vi "Core_Chem_User_Interface_v3.1.vi"() -> ()   [LabVIEW 2014]
uses:
  <vilib>/dex/Stream Element Allocation Mode.ctl
  C:/Program Files (x86)/National Instruments/LabVIEW 2014/examples/Data Communication/Network Streams/Simple Network Streams/support/Network Stream Command.ctl
  <vilib>/Platform/TimedLoop/XDataNode/timing_clust.ctl
  <vilib>/Platform/TimedLoop/XDataNode/nitl_modes.ctl
  <vilib>/Platform/TimedLoop/XDataNode/wakeup.ctl
  <vilib>/Utility/tcp.llb/UDP Multicast Read-Only Open.vi
  <vilib>/platform/TimedLoop/XDataNode/XDataNode.xnode
  <vilib>/Platform/TimedLoop/XDataNode/XDNodeRunTimeDep.lvlib
  <vilib>/FTP/NI_FTP.lvlib
panel:
  out "Network disconnected":bool
  out "cRIO connection status":bool
  out "Network Check error out":errorcluster
  out "SO2 Zeroing (Inflight)\nTime Remain (sec)":u32
  in  "eV6 User set time \n(Inflight) (sec)":i32=120
  in  "SO2 Inflight \nZeroing":bool
  out "Create folder error out 2":errorcluster
  out "Create folder error out":errorcluster
  in  "Confirm Flight Number":bool
  out "PRTAFT_UDP_In":string
  out "TWBOZO01":string
  out "CABOZO01":string
  out "TEIOZO01":string
  out "CHTSOO01":string
  out "CHFGGA01":string
  out "AL52CO01":string
  in  "Flight Number":string
  in  "Tab Control":T1(tab)
  out "FGGA preflight Des 17":string="Preflight - Start minimum 2 hours before take-off\n\n1. Ensure no bags/jackets are stowed on seat backs and behind seats in front of core chemistry rack at all times.\n\n2. Remove inlet covers if applicable.\n\n3. Connect Lilliput mini TFT/LCD VGA cable to FGGA VIDEO (back panel) and PS2 Keyboard/Mouse cables to FGGA Connectors (back panel). TFT/LCD screen kept in WAS/GAS rack Zargers Box. Keyboard/Mouse kept bottom of chemistry rack. (DO NOT disconnect PS2 cable). Connect TFT/LCD AC/DC PSU to 6026-8-98 Amphenol (SSP9) and make 230 Vac CB.\n\n4. Ensure all circuit breakers are pushed in, except 230Vac and 28Vdc, UPS switch off (down) and AL5002 CO Plasma Lamp switch off (down), WoW key to normal (horizontal).\n\n5. Wait for ALL network switches on the aircraft to be up and running before start-up. On the Flight Manager's Interface on the Flight Manager laptop, check SSP icons status (top row) should be all green.  \n\n6. Check AboutTime has synchronised laptop clock to aircraft timeservers (Filiberto/Gaston).\n\nClick the PowerUp Tab."
  out "FGGA preflight Des 16":string="PowerUp\n\n1.\tSSP9 forward face\tMake 3 CBs\n\n2.\tPWRDIST \t\tMake 230Vac CB \n                     Switch UPS On \t[UP]\n                     Make 28Vdc CB\n                     Check 28VDC OK Green Light comes on\n\n3.\tCore Chemistry e-Log\nComplete Core Chemistry e-Log in WordPad (Bnnn_CoreChemLog_v2.2), save on Flight Manager's laptop (192.168.101.180/      flt_folders/Bnnn); Fill in header with date, flight number and your name/initials.\n\n4. Wait for MFM flow rate to display non zero value.\n\n5.\tSAMPUMP\t\t\n - Switch WoW override key (vertical) to check pump starts, and MFM flowrate increase (>20 LPM) on the right hand plot. \n - Switch off WoW override\t\t\t\t [NORM, key horizontal]\n\nClick the 2B Ozone tab if operated, otherwise, click the UDP tab.\n\n\n"
  out "MFM":dbl(graph)
  in  "Ambient = OFF\nCabin = ON":bool
  out "FGGA preflight Des 15":string="2B Ozone Preflight\n\n1.\tSelect either Ambient or Cabin Air mode (default should be OFF for Ambient air mode).\n\n2. Check flowrate is greater than 2000 sccm on the right hand plot.\n\nClick the UDP tab."
  out "2B Ozone concentration":dbl(graph)
  out "2B Ozone flow rate":dbl(graph)
  out "2BOzone Event error out":errorcluster
  out "2BOzone command sender error out":errorcluster
  out "FGGA preflight Des 20":string="4. Check derived parameters in DECADES (192.168.101.110 & 192.168.101.108). 574 Ozone TEi49C; 588 CO AL5002; 611 SO2 TEi43i; 903 - 905 FGGA; 910 / 920 Ozone 2B."
  out "FGGA preflight Des 14":string="UDP Preflight\n1. Check all UDP packets are updating.  Unix time increasing by 1 sec (3rd parameter).\n2. Check flight number is correct.\n3. Confirm flight number and check it appears in the UDP packet (6th parameter). "
  in  "name":string="239.1.4.6"
  in  "Port":u16=50001
  out "FGGA":string
  out "CO":string
  out "TEi49 Ozone":string
  out "2B Cabin Ozone":string
  out "2B Ambient Ozone":string
  out "SO2":string
  in  "Ozone Zeroing Abort":bool
  out "Ozone Zeroing\nTime Remain (sec)":u32
  in  "Ozone Zeroing":bool
  out "TEI49 Sample Flow B":dbl(graph)
  out "TEi49 Concentration":dbl(graph)
  out "TEI49 Sample Flow A":dbl(graph)
  out "FGGA preflight Des 13":string="TEi49 Ozone PRE-FLIGHT - LAST ACTIONS BEFORE SEAT-BELTING DOWN (PRIOR TO ENGINES START)\n\n1. Ozone monitor zeroing\t\t[10 min minimum]\n\n\n2. Check TEi49 zero value and note down value in e-Log. \n"
  out "FGGA preflight Des 12":string="TEi49 Ozone Preflight\n\n1. Check nominal sample flowrate on both channels is ~0.7 LPM."
  out "Ozone Event error out":errorcluster
  out "Ozone command sender error out":errorcluster
  in  "Ozone UDP Time Offset":i32=1
  in  "eV8 span\n(sec)":i32=120
  in  "eV9 span\nflush (sec)":i32=60
  in  "SO2 Span Calibration":bool
  in  "eV9 zero\nflush (sec)":i32=15
  in  "SO2 Zero Calibration":bool
  in  "eV8 zero\n(sec)":i32=30
  in  "SO2 Calibration Abort":bool
  out "SO2 react pressure":dbl(graph)
  in  "Prepare SO2 Zero Gas":bool
  in  "Prepare SO2 Span Gas":bool
  in  "Auto Zeroing \ninterval (sec)":i32=600
  out "Next Auto Zero\nStarts in (sec)":u32
  out "Auto Zero\nIndicator":string="Auto Zero Inactive; Manual Zero Allow"
  out "SO2 Resume Zeroing\nCount down timer (sec)":u32
  in  "SO2 Pause\nAuto Zeroing":bool
  out "TEi43i Concentration scaled / raw":cluster{dbl, dbl}(graph)
  in  "SO2 Auto Zeroing":bool
  out "mean zero\ncal status":bool
  out "SO2 Sensitivity":dbl format="%.2g"
  out "SO2 Zero":dbl format="%.2g"
  in  "eV9 Flush User\nset time (sec)":i32=15
  in  "MFC_3 User Set Value":dbl=2.0
  in  "MFC_2 User Set Value":dbl=2.5
  in  "eV6 User\nset time (sec)":i32=600
  out "SO2 Flush\nTime Remain (sec)":u32
  out "TEI43i MFC3 Sample Flow":dbl(graph)
  out "TEI43C Sample Flow":dbl(graph)
  out "TEI43i MFC2 Cal Flow":dbl(graph)
  out "SO2 Zero CAL\nTime Remain (sec)":u32
  out "SO2 Zero CAL Flush\nTime Remain (sec)":u32
  in  "SO2 Zero CAL":bool
  out "FGGA preflight Des 11":string="TEi43 SO2 Inflight Zero Calibration"
  in  "SO2 GND Zeroing":bool
  out "SO2 Zeroing\nTime Remain (sec)":u32
  out "FGGA preflight Des 10":string="TEi43 SO2 PRE-FLIGHT - LAST ACTIONS BEFORE SEAT-BELTING DOWN (PRIOR TO ENGINES START)\n\n1. SO2 monitors zeroing\t\t[10 min minimum]\n\n2. Check TEi43i or TEi43C zero value and note down value in e-Log.\n\n3. Enable SO2 auto zeroing (if required) and check zeroing interval. "
  in  "SO2 Flush":bool
  out "FGGA preflight Des 9":string="TEi43 SO2 Preflight\n\n1. Check nominal sample flowrate is (2.0 LPM / 1.5 LPM) on the (TEi43i / TEi43c) right hand plot.\n\nSPAN GAS\n1. Connect SO2 Calibration gas to caldeck, then.\n\n2. Press SO2 flush button, MFC2 cal flow should increase to 2.5 SLPM.\nMonitor MFC2 flow rate to make sure the reading decreases from 2.5 SLPM to 0.0 SLPM.\nCheck pressure content and delivery gauges also reads zero.\nIf pressure content & delivery gauges do NOT read zero, press SO2 flush button again until they do.\n\n3. Back out V2, Quickly open and close cylinder valve 1, Set delivery pressure to 3 bar on V2. \n\n4. Repeat step 2) to 3) three times.\n\n5. Open cylinder valve 1, system is ready. Note down content pressure in elog.\n\n6. Press SO2 Span Calibration button to start Span calibration. \n\nZERO AIR\n1. Connect BTCA Zero Air gas to caldeck, then.\n\n2. Set ev9 flush user time to 60 secs and press SO2 Flush button.\n\n3. Press SO2 Zero Calibration button to start Zero Air calibration."
  in  "eV9 flush User\nset time (sec)":i32=30
  in  "eV8 User\nset time (sec)":i32=60
  out "SO2 Event error out":errorcluster
  out "SO2 command sender \nerror out":errorcluster
  in  "SO2 UDP Time Offset":i32=1
  in  "CO Monitor Troubleshooting":bool
  out "Lamp Temperature":dbl(graph)
  out "CO CAL Status":bool
  in  "CO CAL":bool
  out "FGGA preflight Des 8":string="CO Preflight and Inflight Calibrations\nHold down the CAL button for 2 secs then release, CAL status should then lit up.\nCheck CO LED lit up at front instrument. If not, refer to\nInflight calibration performed on 45 minutes interval or more frequently if lamp temperature > 35.5 degC."
  in  "Prepare Gases":bool
  out "FGGA preflight Des 7":string="AL5002 CO Preflight Checks\n\n1.\n\n2. Start CO Vacuum. NB: If there is problem with the software control, use manual override switch [up] on CALDECK front panel\n\n3. CO Checks - charts on the right hand side\n    Lamp Flow Controller ~ 40 ml/min\n    Monochromator Flow Controller ~ 30 ml/min\n    Fluorescence Cell Pressure ~ 7.5 Torr\n\nIf Lamp/Mono flows are low, manual valves (V1 -> V5) may still be shut, or pressure adjusting valves (ALREG1 & 2) have not been set > 2 bar\n\nIf Cell pressure is 10 Torr (max range), check that COPUMP is running and eV7 is opened (CO Vacuum eV7 is ON).\n\n4. Switch Plasma Lamp at the front panel UP\n\nDetector count rate (on 'Raw Signal' or F2 instrument touchscreen) should increase to >=10000 Hz within a minute.  Recycle plasma lamp switch (off/on) if no significant increase in count rate after 10 mins.  CO concentration should increase (100s ppb). \n     \n\n"
  in  "CO Vaccum (eV7)":bool
  out "Raw Signal":dbl(graph)
  out "CO Concentration":dbl(graph)
  out "Fluorescence Cell Pressure":dbl(graph)
  out "Monochromator Flow":dbl(graph)
  out "Lamp Flow Controller":dbl(graph)
  in  "CO UDP Time Offset":i32=1
  out "CO2 Pressure\nDelivery (PSIA)":dbl(slide) scale=0.0..100.0
  out "Std\nContent (barG)":dbl(slide) scale=0.0..220.0
  out "N2\nContent (barG)":dbl(slide) scale=0.0..220.0
  out "CO2\nContent (barG)":dbl(slide) scale=0.0..170.0
  out "CO Event error out":errorcluster
  out "CO command sender error out":errorcluster
  out "CO Zero":T2(array[cluster])
  out "CO Sensitivity":T3(array[cluster])
  in  "FGGA Calibration Abort":bool
  out "Ring Down Time RDA & RDB":cluster{dbl, dbl}(graph)
  in  "Line Lock Setting Change":bool
  out "Cell temperature":dbl(graph)
  out "Cell pressure":dbl(graph)
  in  "Manual FGGA Pump":bool
  out "CO2":dbl(graph)
  out "CH4":dbl(graph)
  out "H2O":dbl(graph)
  out "WoW Flag":string="0"
  in  "FGGA pump\nsync to WoW":bool
  out "CH4 Dry":dbl(graph)
  out "CO2 Dry":dbl(graph)
  out "MFC1 Cal Flow":dbl(graph)
  out "Flush Target Tank\nTime Remain (sec)":u32
  out "Flush Low Tank\nTime Remain (sec)":u32
  out "Flush High Tank\nTime Remain (sec)":u32
  in  "Flush Target Tank":bool
  in  "Flush Low Tank":bool
  in  "Flush High Tank":bool
  in  "FGGA Restart":bool
  out "FGGA preflight Des 6":string="FGGA Instrument Controls"
  in  "High Cal":bool
  out "High Cal\nFlush Time Remain (sec)":u32
  out "High Cal\nCal Time Remain (sec)":u32
  in  "Low Cal":bool
  in  "Target Cal":bool
  in  "Span Cal - \nHigh Cal, CO Cal, Low Cal":bool
  out "Low Cal\nFlush Time Remain (sec)":u32
  out "Low Cal\nCal Time Remain (sec)":u32
  out "Target Cal\nFlush Time Remain (sec)":u32
  out "Target Cal\nCal Time Remain (sec)":u32
  in  "MFC_1 User Set Value":dbl=2.0
  out "FGGA preflight Des 5":string="FGGA Inflight Calibrations"
  out "FGGA preflight Des 4":string="FGGA Ground Preflight Checks\n\n1. Switch FGGA pump ON\n\n2. Check cavity pressure ~50 Torr\n\n3. Switch FGGA pump OFF\n\n4. Enable FGGA pump sync to WoW\n\n5.. Check Time Synchronisation\n\n6. Check CO2 & CH4 values\n\nIf CO2 & CH4 values are -1 ppm, follow the \nchange linelock settings procedure.\n\n\n\n\n\nLAST ACTION BEFORE SEAT-BELTING \nDOWN (PRIOR TO ENGINES START)\n\n1. Disconnect Monitor & stow away. Leave Keyboard & Mouse connected. Place keyboard at the bottom\nof the rack.\n\n"
  out "FGGA preflight Des 3":string="FGGA CAL Gas Purge\n\nFor each cylinder in gas stowage, check that,\n\n1. V1 Closed\n    V3 Closed\n    V4 Make sure arrow positioned downwards (i.e. flow points to gas line)\n\n2. V3 Open (turn anti-clockwise)\n\n3. Use the button on the right according to the operating cylinder to flush the line. Monitor the MFC flow rate to make sure the reading decreases from 3 to zero. (ie fully flushed). Pressure content & delivery gauges should also read zero.\n\n4. V3 Close (turn clockwise)\n\n5. V1 Open / Close quickly\n         Check delivery pressure gauge is ~ 40 PSI \n         (Use V2 to increase if necessary)\n\n6. Repeat steps 2) to 5) three times\n\n7. V3 Close (turn clockwise)\n\n8. V1 Open, check V2 ~ 40 PSIG\n\n9. V3 Open - System is ready"
  out "FGGA command sender error out":errorcluster
  out "FGGA Event Error out":errorcluster
  in  "FGGA UDP Time Offset":i32=1
  in  "FGGA Shutdown":bool
  in  "Postflight Procedures":bool
  in  "FTP ASCII Files to Local":bool
  in  "Transfer FGGA Files":bool
  out "FGGA preflight Des 18":string="Postflight\n\n1. Perform SO2 Span Gas Calibration (if necessary). \n\n2. Press the FTP ASCII File to Local button to transfer ASCII files to flight folder.\n\n\n3. Press the Transfer FGGA Files button to transfer FGGA files to flight folder. \n\n\n4. Shutdown FGGA.\n\n\n5. View Postflight Procedures."
  out "File List":string[](array[string])
  out "FGGA File Transfer Error out":errorcluster
  out "Move to FM Error out":errorcluster
  out "USB Disk Space Used %":dbl(slide) scale=0.0..100.0
  out "PTP Sync":bool
  out "CPU Total %":dbl(graph)
  out "PRTAFT_DLU":string
  in  "Pause Auto Zero Count \nDown set time (sec)":i32=600
  out "Calibration gas cylinder \nconcentration (ppb)":dbl format="%.4g"
  in  "Save Calibration gas\ncylinder concentration to file":bool
  in  "Calibration gas cylinder \nconcentration (ppb)":dbl=500.0 format="%.4g"
  in  "Simulate MOCCA Conc":dbl
  in  "MOCCA window \ndelay time (sec)":i32=30
  in  "MOCCA Limit":i32=800
  in  "SO2 Inflight MOCCA Alarm\n(default = OFF)":bool
  in  "Offset Mean Zero Calculation (default = ON)\nOFF = User input\nOn = Mean zero calculated with ev8":bool=TRUE
  out "FGGA preflight Des 19":string="This tab controls ONLY for advanced operators."
  in  "Inst_alm_thresh":i32=220
  in  "3hr_alm_thresh":i32=80
  in  "Simulate Inst Conc":i32
  in  "Simulate 3hr Average Conc":dbl
  in  "Simulate 2B Conc":bool
  in  "Ozone eV6":bool
  in  "Simulate Conc":bool
  in  "8hr TWA Limit":i32=490
  in  "10mins STEL Limit":i32=800
  in  "SO2 Sensitivity":dbl=1.1
  in  "SO2 Zero":dbl
  in  "Simulate TWA Conc":dbl
  in  "Simulate STEL Conc":dbl
  in  "MFC_3\nSLPM Value":dbl=2.0
  in  "MFC_2\nSLPM Value":dbl
  in  "SO2 eV6":bool
  in  "eV8":bool
  in  "eV9":bool
  in  "eV4":bool
  in  "eV3":bool
  in  "MFC_1\nSLPM Value":dbl
  in  "eV2":bool
  in  "eV1":bool
  in  "cRIO File IO Stop\n(USB Flash Drive Unmount)":bool
  # "Unix time"
  # "Flight Number"
  # "concentration (scaled)\npmt_volt\nlamp_volt\nlamp_intens\ninternal_temper\nreact_temper\nreact_press\nflow\nflags\nten_min_so2\neight_hr_so2\nten_min_so2_alm\neight_hr_so2_alm\nMFC_2absolute_pres\nMFC_2temperature\nMFC_2volumetic_flow\nMFC_2mass_flow\nMFC_2set_point\nMFC_3_absolute_pres\nMFC_3_temperature\nMFC_3volumetic_flow\nMFC_3mass_flow\nMFC_3set_point\nV6\nV8\nV9\nMFC2_Set_Value\nMFC3_Set_Value\nconcentration (raw)\nmean calculation status\noffset\nsensitivity\nev8_user_set_time\nauto_zeroing_control\nev8_zero_interval\nMOCCA_inflight_alarm\nMOCCA_time_window_delay\nMOCCA_SO2_limit\n10 min STEL limit\n8 hour TWA limit\nSO2 cal gas cylin conc\nsimulate_SO2_conc_control\nMOCCA_SO2_sim_value\nMOCCA_SO2_alarm"
  # "Unix time"
  # "Unix time"
  # "Unix time"
  # "Unix time"
  # "Flight Number"
  # "Flight Number"
  # "Flight Number"
  # "Flight Number"
  # "conc\ntemp\npress\nflow\nthreehr_oz\nInst_alarm\nthreehr_alarm"
  # "ch4\nco2\nh2o\npress_torr\ntemp_c\nfit_flag\nrda_usec\nrdb_usec\nch4_dry\nco2_dry\nMFC_1_absolute_pres\nMFC_1_temperature\nMFC_1volumetic_flow\nMFC_1mass_flow\nMFC_1set_point\nV1\nV2\nV3\nV4\nrestart_FGGA\nFGGA_Pump\nCAL_MFC_1Set_Value"
  # "conc\ntemp\npress\nflow"
  # "conc\nbenchtemp\npress\ncellAint\ncellBint\nFlowA\nFlowB\nlamptemp\nflag\nV6"
  # "conc\ncounts\nsens\nzero\nlampflow\nlamptemp\nmonoflow\nmonotemp\nmonopress\ncellpress\ncalpress\ntemppmt\ncalconc\nerr\ncal_counter\nerr_counter\nCO_vacuum_status\nIn_Cal\nALEG1_press_delivery\nALREG1_press_content\nALREG2_press_content\nALREG3_press_content"
  # "TEi43c"
  # "TEi43i"
  # "SO2 Inflight ZERO CAL SETTINGS"
  # "FGGA"
  # "2B Ozone"
  # "TEi49C  - Ozone"
  # "TEi43 - SO2"
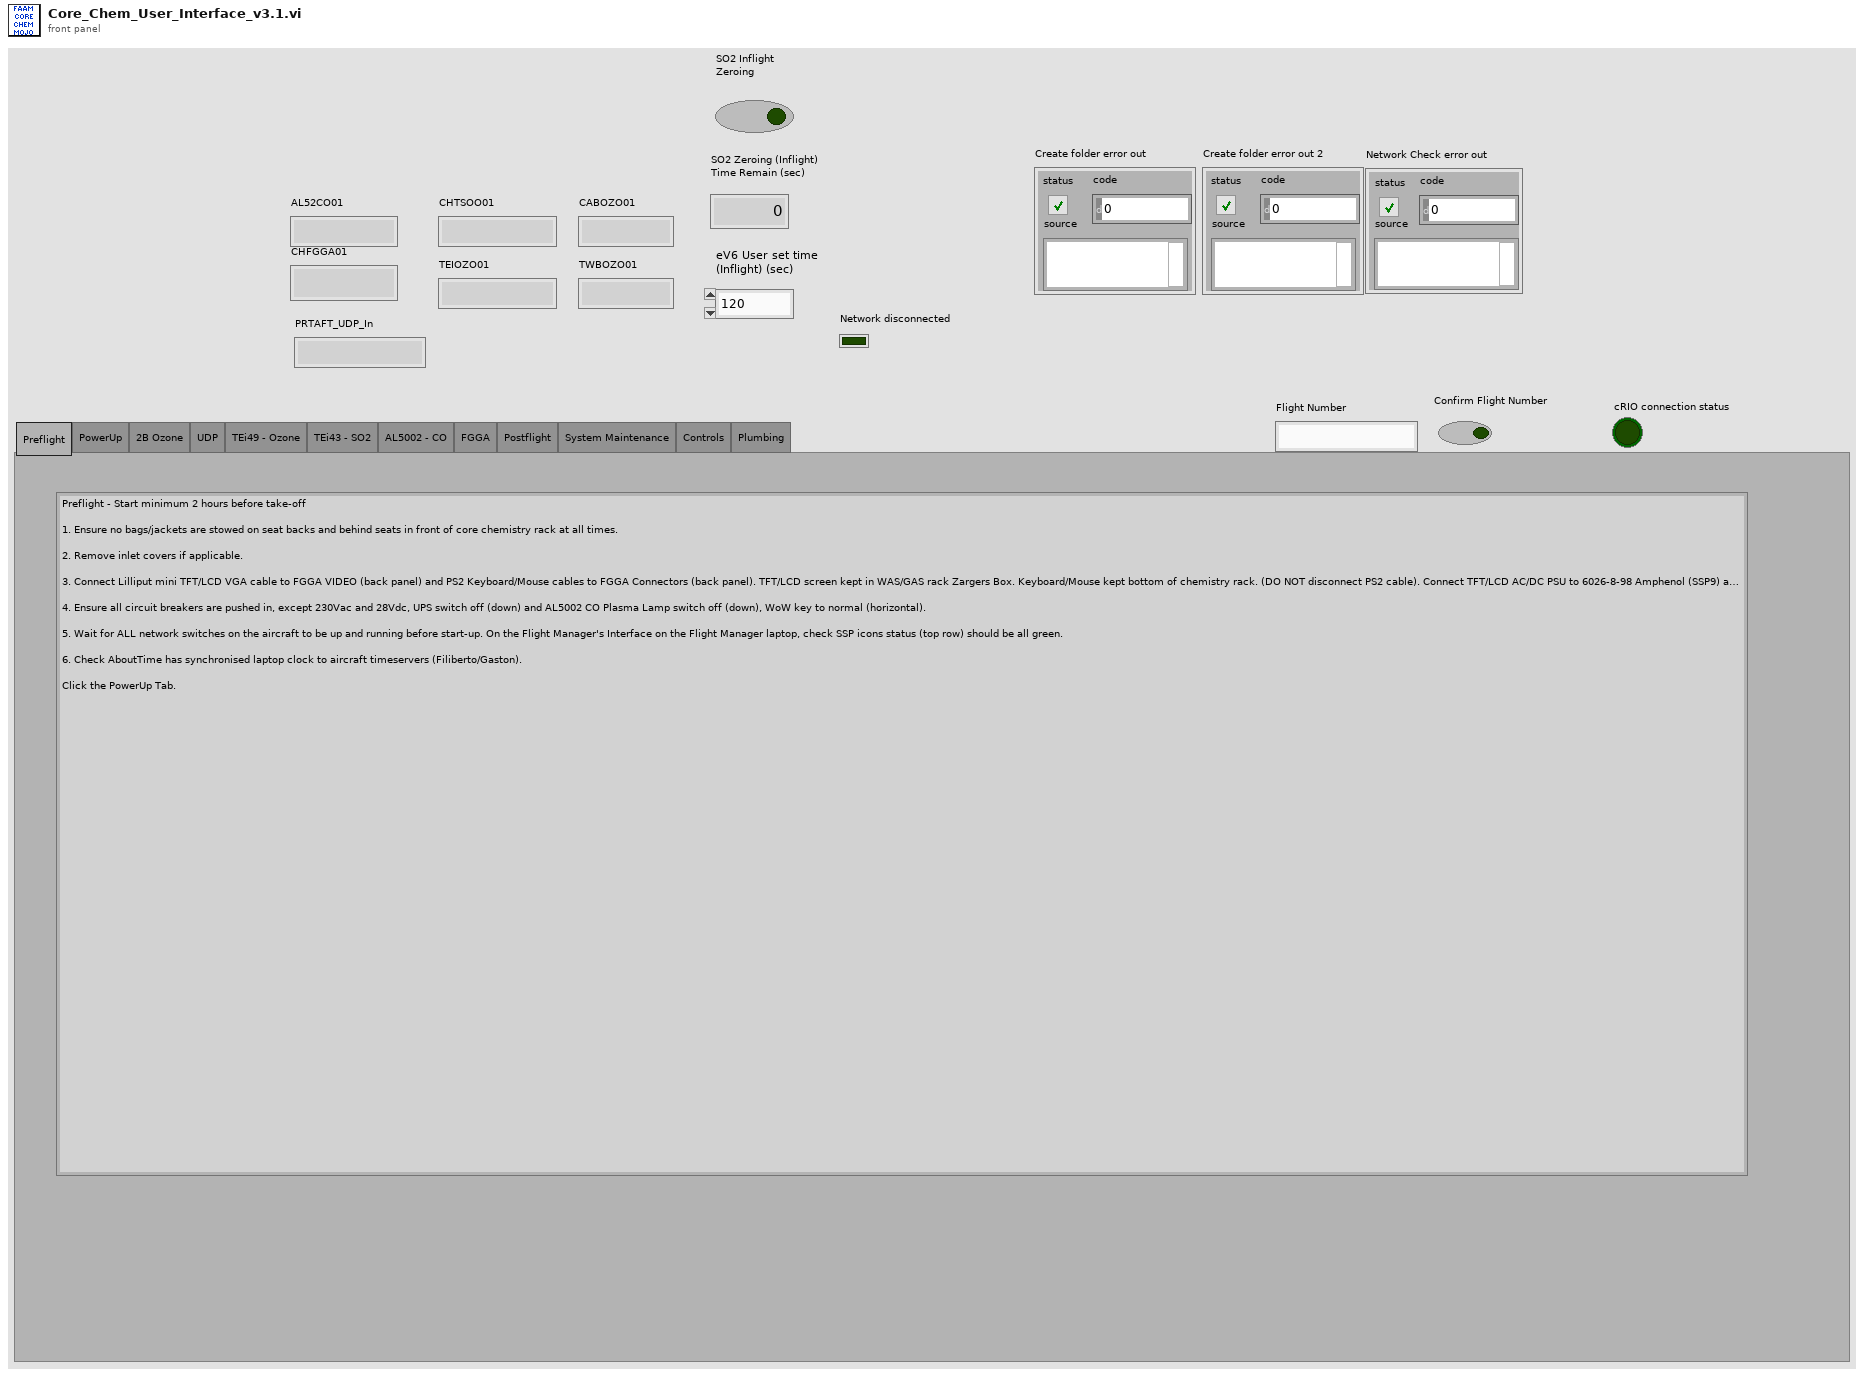
[diagram p1: front panel]
types:
  T1 = enum32{"Preflight", "PowerUp", "2B Ozone", "UDP", "TEi49 - Ozone", "TEi43 - SO2", "AL5002 - CO", "FGGA", "Postflight", "System Maintenance", "Controls", "Plumbing"}
  T2 = cluster{"time stamp":timestamp, "CO Offset":dbl}[]
  T3 = cluster{"time stamp":timestamp, "CO Sensitivity":dbl}[]
  T4 = typedef "Network Stream Command.ctl" = cluster{"Message":string, "Message Data":variant}
  T5 = typedef "Stream Element Allocation Mode.ctl" = u32
  T6 = typedef "XDNodeRunTimeDep.lvlib/timing_clust.ctl" = cluster{"Expected End [f-1]":u64, "Actual End [f-1]":u64, "Finished Late? [f-1]":bool, "Expected End [i-1]":u64, "Actual End [i-1]":u64, "Finished Late? [i-1]":bool, "Expected Start [i]":u64, "Actual Start [i]":u64, "Expected Start [f]":u64, "Actual Start [f]":u64, "Source Name":string, "Structure Name":string, "Period":i64, "Deadline":i64, "Offset":i64, "Start":i64, "Priority":i32, "Timeout":i32, "Mode":T7, "Wakeup Reason":T8, "Error":errorcluster, "Source Type":string, "Secondary Source Type":string, "Global End Time":u64, "Global Start Time":u64, "Frame Duration":u64, "Iteration Duration":u64, "Assigned CPU":i32, "I/O Scan Engine Mode":u32}
  T7 = typedef "XDNodeRunTimeDep.lvlib/nitl_modes.ctl" = enum32{"No Change", "Process missed periods, maintain original phase", "Discard missed periods, maintain original phase", "Process missed periods, ignore original phase", "Discard missed periods, ignore original phase"}
  T8 = typedef "XDNodeRunTimeDep.lvlib/wakeup.ctl" = enum32{"Normal", "Aborted", "Asynchronous wakeup", "Timing source error", "Timed loop error", "Timeout"}
  T9 = typedef "NI_FTP.lvlib/FTP Session.ctl" = refnum<k5>
  T10 = typedef "NI_FTP.lvlib/FTP File Info.ctl" = cluster{"type":enum16{"unknown", "file", "dir", "link"}, "permissions":string, "owner":string, "group":string, "size":i32, "date":string, "name":string, "link name":string}
  T11 = cluster{"Message":string, "Message 2":string, "Message 3":string}
  T12 = cluster{"Message":string, "Message 2":string, "Message 3":string, "Message 4":string}
  T13 = cluster{"Message":string, "Message 3":string, "Message 4":string}
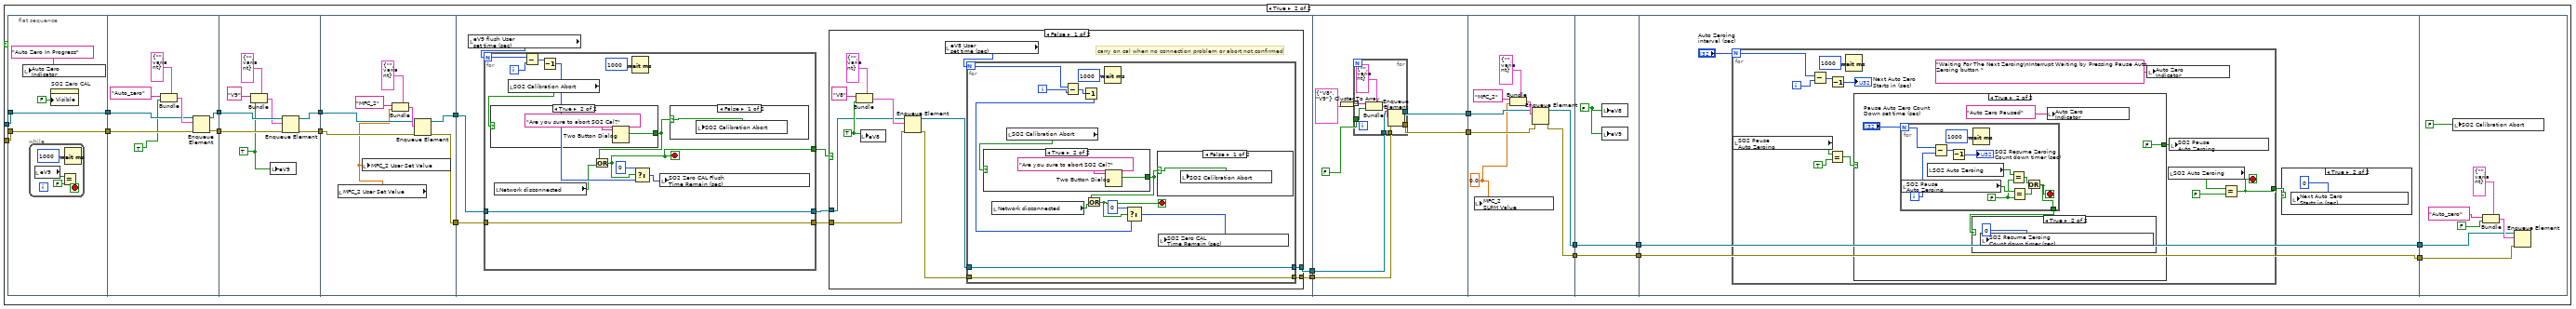
[diagram p6: hidden frame]
diagram:
  w8 = "XXXX"
  w10 = 0
  w11 = 0.0
  w17 = T4 {"Message"="", "Message Data"=variant} ("Message Cluster")
  w23 = T5 0 items=["allocate as needed", "pre-allocate"] ("element allocation mode")
  w29 = T4 {"Message"="", "Message Data"=variant} ("Message Cluster")
  w35 = T5 0 items=["allocate as needed", "pre-allocate"] ("element allocation mode")
  w40 = T4 {"Message"="", "Message Data"=variant} ("Message Cluster")
  w45 = T5 0 items=["allocate as needed", "pre-allocate"] ("element allocation mode")
  w54 = T5 0 items=["allocate as needed", "pre-allocate"] ("element allocation mode")
  w56 = T4 {"Message"="", "Message Data"=variant} ("Message Cluster")
  w63 = T5 0 items=["allocate as needed", "pre-allocate"] ("element allocation mode")
  w65 = T4 {"Message"="", "Message Data"=variant} ("Message Cluster")
  n1 = local write "cRIO File IO Stop\n(USB Flash Drive Unmount)"(FALSE ("Stop File Write")) -> ()
  n2 = local write "Flight Number"(w8) -> ()
  n3 = while {
    shift-right: [w69] -> _
    shift-left: w8 -> [w68]
    stop <- FALSE stop-if-true
    n4 = Not Equal?(x=w68, y="Flight Number") -> (x != y?=w71:bool)
    n5 = case shown="True" w71 {
      tunnel: [w74 w75] -> w69
      tunnel: "Flight Number" -> [_ w75]
      tunnel: w68 -> [w74 _]
      frame False {
      }
      frame True {
        n6 = One Button Dialog(message="Flight Number changed,\nPress flight number button to confirm") -> ()  [unwired: 1 in, 1 out]
      }
    }
    n7 = Wait (ms)(milliseconds to wait=u32 1000) -> ()  [unwired: 1 out]
  }
  n8 = while {
    stop <- FALSE stop-if-true
    # "UDP Read"
    n9 = String To IP(1:"name") -> (0:w82:u32)
    n10 = call-poly <vilib>:"UDP Multicast Open.vi"("multicast addr"=w82, "port"="Port") -> ("error out"=w80:errorcluster, "connection ID"=w79:refnum<k16>)  [unwired: 7 in, 1 out]
    n11 = Wait (ms)(milliseconds to wait=u32 1000) -> ()  [unwired: 1 out]
    n12 = case shown="No Error" w80 {
      selector: w80 -> [w86 _]
      tunnel: w79 -> [w85 _]
      frame No Error {
        w84 = ""
        n13 = while {
          tunnel: w86 -> [w132]
          tunnel: w85 -> [w131]
          shift-right: [w127] -> _
          shift-left: w84 -> [w128]
          shift-right: [w118] -> _
          shift-left: w84 -> [w120]
          shift-right: [w112] -> _
          shift-left: w84 -> [w114]
          shift-right: [w106] -> _
          shift-left: w84 -> [w107]
          shift-right: [w100] -> _
          shift-left: w84 -> [w101]
          shift-right: [w94] -> _
          shift-left: w84 -> [w95]
          shift-right: [w88] -> _
          shift-left: w84 -> [w89]
          stop <- w130 stop-if-true
          n14 = UDP Read(connection ID=w131, 8:w132) -> (data out=w87:string, error out=w130:errorcluster)  [unwired: 2 in, 3 out]
          n15 = Match Pattern(string=w87, regular expression="$TEIOZO") -> (match substring=w126:string, after substring=w125:string)  [unwired: 1 in, 2 out]
          n16 = Match Pattern(string=w87, regular expression="$TWBOZO01,") -> (match substring=w104:string, after substring=w103:string)  [unwired: 1 in, 2 out]
          n17 = Match Pattern(string=w87, regular expression="$CABOZO01,") -> (match substring=w110:string, after substring=w109:string)  [unwired: 1 in, 2 out]
          n18 = Match Pattern(string=w87, regular expression="$CHTSOO") -> (match substring=w98:string, after substring=w97:string)  [unwired: 1 in, 2 out]
          n19 = Match Pattern(string=w87, regular expression="$CHFGGA01,") -> (match substring=w122:string, after substring=w121:string)  [unwired: 1 in, 2 out]
          n20 = Match Pattern(string=w87, regular expression="$AL52CO01,") -> (match substring=w116:string, after substring=w115:string)  [unwired: 1 in, 2 out]
          n21 = Match Pattern(string=w87, regular expression="$PRTAFT01,") -> (match substring=w93:string, after substring=w92:string)  [unwired: 1 in, 2 out]
          n22 = Concatenate Strings(w126, w125) -> (w124:string)
          n23 = Concatenate Strings(w104, w103) -> (w102:string)
          n24 = Concatenate Strings(w110, w109) -> (w108:string)
          n25 = Concatenate Strings(w98, w97) -> (w96:string)
          n26 = Concatenate Strings(w122, w121) -> (w119:string)
          n27 = Concatenate Strings(w116, w115) -> (w113:string)
          n28 = Concatenate Strings(w93, w92) -> (w90:string)
          n29 = Replace Substring(4:w102, 5:w101) -> (1:w100:string)  [unwired: 2 in, 1 out]
          "TWBOZO01" <- w100
          n30 = Replace Substring(4:w124, 5:w128) -> (1:w127:string)  [unwired: 2 in, 1 out]
          "TEIOZO01" <- w127
          n31 = Replace Substring(4:w108, 5:w107) -> (1:w106:string)  [unwired: 2 in, 1 out]
          "CABOZO01" <- w106
          n32 = Replace Substring(4:w96, 5:w95) -> (1:w94:string)  [unwired: 2 in, 1 out]
          "CHTSOO01" <- w94
          n33 = Replace Substring(4:w113, 5:w114) -> (1:w112:string)  [unwired: 2 in, 1 out]
          "AL52CO01" <- w112
          n34 = Replace Substring(4:w119, 5:w120) -> (1:w118:string)  [unwired: 2 in, 1 out]
          "CHFGGA01" <- w118
          n35 = Replace Substring(4:w90, 5:w89) -> (1:w88:string)  [unwired: 2 in, 1 out]
          "PRTAFT_UDP_In" <- w88
        }
      }
      frame Error {
      }
    }
  }
  n36 = Obtain Queue(name (unnamed)="CO_Command", element data type=w65) -> (queue out=w16:refnum<queue>, error out=w59:errorcluster)  [unwired: 3 in, 1 out]
  n37 = Create Network Stream Writer Endpoint(6:w63, 7:10 ("writer buffer size"), 9:w65, 10:"//192.168.101.17/command/reader/CO" ("reader url"), 11:"/command/writer/CO" ("writer name")) -> (0:w62:errorcluster, 3:w61:refnum<k21>)  [unwired: 2 in]
  n38 = while {
    tunnel: w16 -> [w136]
    tunnel: w59 -> [w135]
    tunnel: [w133] -> _
    stop <- FALSE stop-if-true
    # "CO UI Event Handler Loop"
    n39 = event shown="[4] \"Confirm Flight Number\": Value Change" {
      selector: _ -> [_ _ _ _ _]
      dyn-events: _ -> [_ _ _ _ _]
      timeout: _ -> [_ _ _ _ _]
      tunnel: w136 -> [w143 w150 w154 w161 w169]
      tunnel: w135 -> [w142 w149 w153 w160 w168]
      tunnel: [w137 w144 w152 w159 w167] -> w133
      event "CO CAL": Value Change {
        n40 = event-data() -> ("NewVal"=w140:bool)  [unwired: 1 in]
        n41 = Bundle(cluster=T4 {"Message"="", "Message Data"=variant} ("Message Cluster"), "Message"="CO CAL", "Message Data"=w140) -> (w138:T4)
        n42 = Enqueue Element(queue=w143, element=w138, error in (no error)=w142) -> (error out=w137:errorcluster)  [unwired: 1 in, 2 out]
      }
      event "CO UDP Time Offset": Value Change {
        n43 = event-data() -> ("NewVal"=w147:i32)  [unwired: 1 in]
        n44 = Bundle(cluster=T4 {"Message"="", "Message Data"=variant} ("Message Cluster"), "Message"="UDP Time Offset", "Message Data"=w147) -> (w145:T4)
        n45 = Enqueue Element(queue=w150, element=w145, error in (no error)=w149) -> (error out=w144:errorcluster)  [unwired: 1 in, 2 out]
      }
      event "CO Vaccum (eV7)": Value Change {
        n46 = event-data() -> ("NewVal"=w151:bool)  [unwired: 1 in]
        n47 = Bundle(cluster=T4 {"Message"="", "Message Data"=variant} ("Message Cluster"), "Message"="CO Vacuum", "Message Data"=w151) -> (w155:T4)
        n48 = Enqueue Element(queue=w154, element=w155, error in (no error)=w153) -> (error out=w152:errorcluster)  [unwired: 1 in, 2 out]
      }
      event "cRIO File IO Stop\n(USB Flash Drive Unmount)": Value Change {
        n49 = event-data() -> ("NewVal"=w158:bool)  [unwired: 1 in]
        n50 = Bundle(cluster=T4 {"Message"="", "Message Data"=variant} ("Message Cluster"), "Message"="Stop File Write", "Message Data"=w158) -> (w162:T4)
        n51 = Enqueue Element(queue=w161, element=w162, error in (no error)=w160) -> (error out=w159:errorcluster)  [unwired: 1 in, 2 out]
      }
      event "Confirm Flight Number": Value Change {
        n52 = event-data() -> ()  [unwired: 1 in, 1 out]
        n53 = flat-sequence {
          tunnel: w168 -> [w171]
          tunnel: w169 -> [w172]
          tunnel: [w172] -> w166
          tunnel: [w171] -> w165
          tunnel: [w174] -> w167
          tunnel: w166 -> [w176]
          tunnel: w165 -> [w175]
          frame #0 {
            n54 = local write "cRIO File IO Stop\n(USB Flash Drive Unmount)"(FALSE ("cRIO File IO Stop\n(USB Flash Drive Unmount)")) -> ()
          }
          frame #1 {
            n55 = local read "Flight Number"() -> (w173:string)
            n56 = Bundle(cluster=T4 {"Message"="", "Message Data"=variant} ("Message Cluster"), "Message"="Flight Number", "Message Data"=w173) -> (w177:T4)
            n57 = Enqueue Element(queue=w176, element=w177, error in (no error)=w175) -> (error out=w174:errorcluster)  [unwired: 1 in, 2 out]
          }
        }
      }
    }
    "CO Event error out" <- w133
  }
  n58 = while {
    tunnel: w16 -> [w187]
    shift-right: [w182] -> _
    shift-left: w61 -> [w184]
    shift-right: [w180] -> w50
    shift-left: w62 -> [w186]
    tunnel: w59 -> [w181]
    stop <- w180 stop-if-true
    # "CO UI Command Sender"
    n59 = Dequeue Element(queue=w187, error in (no error)=w181) -> (element=w183:T4)  [unwired: 1 in, 3 out]
    n60 = Unbundle By Name(w183) -> ("Message"=w185:string)
    n61 = case shown="\"UDP Time Offset\"" w185 {
      tunnel: w186 -> [w188 w192 w199 w206 w213 w220]
      tunnel: w184 -> [w189 w195 w202 w209 w216 w223]
      tunnel: w183 -> [_ w194 w201 w208 w215 w222]
      tunnel: [w188 w191 w198 w205 w212 w219] -> w180
      tunnel: [w189 w190 w197 w204 w211 w218] -> w182
      frame "False", Default {
      }
      frame "CO CAL" {
        n62 = shared-variable-write(w195, w192, w194) -> (w193:refnum<k21>, w196:errorcluster)  [unwired: 1 in, 1 out]
        n63 = Flush Stream(8:w196, 11:w193) -> (0:w191:errorcluster, 3:w190:refnum<k21>)  [unwired: 2 in, 1 out]
      }
      frame "UDP Time Offset" {
        n64 = shared-variable-write(w202, w199, w201) -> (w200:refnum<k21>, w203:errorcluster)  [unwired: 1 in, 1 out]
        n65 = Flush Stream(8:w203, 11:w200) -> (0:w198:errorcluster, 3:w197:refnum<k21>)  [unwired: 2 in, 1 out]
      }
      frame "Stop File Write" {
        n66 = shared-variable-write(w209, w206, w208) -> (w207:refnum<k21>, w210:errorcluster)  [unwired: 1 in, 1 out]
        n67 = Flush Stream(8:w210, 11:w207) -> (0:w205:errorcluster, 3:w204:refnum<k21>)  [unwired: 2 in, 1 out]
      }
      frame "Flight Number" {
        n68 = shared-variable-write(w216, w213, w215) -> (w214:refnum<k21>, w217:errorcluster)  [unwired: 1 in, 1 out]
        n69 = Flush Stream(8:w217, 11:w214) -> (0:w212:errorcluster, 3:w211:refnum<k21>)  [unwired: 2 in, 1 out]
      }
      frame "CO Vacuum" {
        n70 = shared-variable-write(w223, w220, w222) -> (w221:refnum<k21>, w224:errorcluster)  [unwired: 1 in, 1 out]
        n71 = Flush Stream(8:w224, 11:w221) -> (0:w219:errorcluster, 3:w218:refnum<k21>)  [unwired: 2 in, 1 out]
      }
    }
  }
  "CO command sender error out" <- w50
  n72 = node-c288() -> (w15:T6)  [unwired: 4 in]
  n73 = Initialize Array(cluster{"time stamp":timestamp, "Y":dbl} {"time stamp"=timestamp(0 s since 1904-01-01), "Y"=0.0}, 30 ("dimension size")) -> (w12:cluster{"time stamp":timestamp, "Y":dbl}[])
  n74 = timed-loop {
    timing: w15 -> [_]
    timing-out: [_] -> w14
    stop <- _ stop-if-true
    # "PC Tasks"
    n75 = node-c288() -> ()  [unwired: 1 in, 1 out]
    n76 = event shown="[0] \"FTP ASCII Files to Local\": Value Change" {
      selector: _ -> [_ _ _ _]
      dyn-events: _ -> [_ _ _ _]
      timeout: _ -> [_ _ _ _]
      event "FTP ASCII Files to Local": Value Change {
        n77 = event-data() -> ()  [unwired: 1 in, 1 out]
        n78 = flat-sequence {
          tunnel: [w233] -> w227
          tunnel: [w245] -> w232
          tunnel: [w244] -> w230
          tunnel: [w243] -> w228
          tunnel: w227 -> [w243]
          tunnel: w232 -> [w303]
          tunnel: [w303] -> w231
          tunnel: w230 -> [w299]
          tunnel: [w298] -> w229
          tunnel: w228 -> [w298]
          tunnel: w231 -> [w309]
          tunnel: w229 -> [w304]
          frame #0 {
            n79 = local read "Flight Number"() -> (w235:string)
            n80 = Concatenate Strings("Confirm Flight Number" ("message"), "\n", w235) -> (w239:string)
            n81 = Two Button Dialog(message=w239, 1:"No" ("F button name (\"Cancel\")"), 2:"Yes" ("T button name (\"OK\")")) -> (T button?=w236:bool)
            n82 = case shown="False" w236 {
              tunnel: w235 -> [_ w242]
              tunnel: [w241 w242] -> w233
              frame False {
                n83 = call "Prompt User for Flight Number2"() -> ("Flight Number BXXX"=w241:string)  [unwired: 17 in, 2 out]
              }
              frame True {
              }
            }
          }
          frame #1 {
            n84 = Get Date/Time In Seconds() -> (seconds since 1Jan1904=w249:timestamp)
            n85 = Format Date/Time String(time format string (%c)="%Y%m%d", seconds (now)=w249) -> (date/time string=w247:string)  [unwired: 1 in]
            n86 = call <vilib>:"FTP Open Session.vi"("address"="192.168.101.17") -> ("error out"=w264:errorcluster, "ftp session"=w265:T9)  [unwired: 7 in, 2 out]
            n87 = Concatenate Strings("Use Today's Date" ("message"), "\r", w247) -> (w253:string)
            n88 = call <vilib>:"FTP Logon.vi"("error in (no error)"=w264, "password"="", "user"="anonymous", "ftp session"=w265) -> ("error out"=w261:errorcluster, "ftp session out"=w260:T9)  [unwired: 4 in, 2 out]
            n89 = Two Button Dialog(message=w253, 1:"No" ("F button name (\"Cancel\")"), 2:"Yes" ("T button name (\"OK\")")) -> (T button?=w250:bool)
            n90 = case shown="False" w250 {
              tunnel: [w268 w269] -> w244
              tunnel: w247 -> [_ w269]
              frame False {
                n91 = call "Prompt User for Date"() -> ("Date"=w268:string)  [unwired: 17 in, 2 out]
              }
              frame True {
              }
            }
            n92 = call <vilib>:"FTP Directory Listing.vi"("error in (no error)"=w261, "directory path"="/U:/data", "ftp session"=w260) -> ("dir list"=w259:T10[])  [unwired: 4 in, 4 out]
            n93 = for {
              tunnel: w259 -> [w289] mode=indexing
              tunnel: [w288] -> w256 mode=indexing
              tunnel: w244 -> [w287]
              # "Extract File Name According to the Date"
              n94 = Unbundle By Name(w289) -> ("name"=w295:string, "name"=w294:string)
              n95 = Match Pattern(string=w294, regular expression="_[0-9]+") -> (match substring=w292:string)  [unwired: 1 in, 3 out]
              n96 = String Subset(string=w292, offset (0)=1) -> (substring=w290:string)  [unwired: 1 in]
              n97 = Equal?(x=w290, y=w287) -> (x = y?=w296:bool)
              n98 = case shown="False" w296 {
                tunnel: w295 -> [_ w297]
                tunnel: [_ w297] -> w288
                frame False {
                }
                frame True {
                }
              }
            }
            n99 = Array Size(array=w256) -> (size(s)=w258:i32)
            n100 = for {
              N: w258 -> [_]
              shift-right: [w276] -> w246
              shift-left: w256 -> [w277]
              shift-right: [w274] -> _
              shift-left: 0 -> [w275]
              # "Remove Empty Array"
              n101 = Index Array(array=w277, index=w275) -> (element=w279:string)
              n102 = Equal?(x=w279, y="") -> (x = y?=w278:bool)
              n103 = case shown="True" w278 {
                tunnel: w277 -> [w283 w286]
                tunnel: w275 -> [w282 w284]
                tunnel: [w283 w285] -> w276
                tunnel: [w281 w284] -> w274
                frame False {
                  n104 = Increment(x=w282) -> (x+1=w281:i32)
                }
                frame True {
                  n105 = Delete From Array(array=w286, index=w284) -> (array with subset deleted=w285:string[])  [unwired: 1 in, 1 out]
                }
              }
            }
            "File List" <- w246
            n106 = for {
              tunnel: w246 -> [w272] mode=indexing
              tunnel: [w270] -> w245 mode=indexing
              # "Specify destination path for each file"
              n107 = Concatenate Strings("C:\\temp\\", w272) -> (w271:string)
              n108 = String To Path(string=w271) -> (path=w270:path)
            }
          }
          frame #2 {
            # "FTP a list of files"
            n109 = call <vilib>:"System Exec.vi"("wait until completion? (T)"=TRUE, "working directory"=path "C:/temp", "standard input"=w299, "command line"="C:\\temp\\transfer_ascii_files.bat") -> ()  [unwired: 4 in, 4 out]
          }
          frame #3 {
            # "Move file from local PC to Flight Folder"
            n110 = Build Path(base path=path "\\\\192.168.101.180\\flt_folders" ("path"), name or relative path=w304) -> (appended path=w311:path)
            n111 = Concatenate Strings(w304, "_" ("string"), "corechem" ("string")) -> (w310:string)
            n112 = Build Path(base path=w311, name or relative path=w310) -> (appended path=w306:path)
            n113 = Create Folder(path (use dialog)=w306) -> (created path=w305:path, error out=→"Create folder error out 2":errorcluster)  [unwired: 2 in, 1 out]
            n114 = for {
              tunnel: w305 -> [w318]
              tunnel: [w317] -> w308
              tunnel: w309 -> [w315] mode=indexing
              n115 = Copy(9:TRUE ("overwrite (F)"), 10:w318, 11:w315) -> (0:w317:errorcluster)  [unwired: 2 in, 2 out]
            }
            "Move to FM Error out" <- w308
          }
          frame #4 {
            n116 = local write "FTP ASCII Files to Local"(FALSE ("FTP Files to Local")) -> ()
          }
        }
      }
      event "Transfer FGGA Files": Value Change {
        n117 = event-data() -> ()  [unwired: 1 in, 6 out]
        n118 = flat-sequence {
          tunnel: [w324] -> w323
          tunnel: w323 -> [w336]
          tunnel: [w336] -> w322
          tunnel: [w335] -> w321
          tunnel: [w334] -> w320
          tunnel: w322 -> [w346]
          tunnel: w321 -> [w345]
          tunnel: w320 -> [w347]
          frame #0 {
            n119 = local read "Flight Number"() -> (w325:string)
            n120 = Concatenate Strings("Confirm Flight Number" ("message"), "\n", w325) -> (w327:string)
            n121 = Two Button Dialog(message=w327, 1:"No" ("F button name (\"Cancel\")"), 2:"Yes" ("T button name (\"OK\")")) -> (T button?=w331:bool)
            n122 = case shown="False" w331 {
              tunnel: w325 -> [_ w333]
              tunnel: [w332 w333] -> w324
              frame False {
                n123 = call "Prompt User for Flight Number"() -> ("Flight Number BXXX"=w332:string)  [unwired: 17 in, 2 out]
              }
              frame True {
              }
            }
          }
          frame #1 {
            n124 = Two Button Dialog(message="Get FGGA Files\nof Today's Date?", 1:"No" ("F button name (\"Cancel\")"), 2:"Yes" ("T button name (\"OK\")")) -> (T button?=w340:bool)
            n125 = case shown="False" w340 {
              selector: w340 -> [w342 w343]
              tunnel: [w342 w343] -> w334
              tunnel: [w341 _] -> w335
              frame False {
                n126 = call "Prompt User for Date"() -> ("Date"=w341:string)  [unwired: 17 in, 2 out]
              }
              frame True {
              }
            }
          }
          frame #2 {
            n127 = Build Path(base path=path "\\\\192.168.101.180\\flt_folders" ("path"), name or relative path=w346) -> (appended path=w351:path)
            n128 = Concatenate Strings(w346, "_" ("string"), "corechem" ("string")) -> (w350:string)
            n129 = Build Path(base path=w351, name or relative path=w350) -> (appended path=w344:path)
            n130 = Create Folder(path (use dialog)=w344) -> (error out=→"Create folder error out":errorcluster)  [unwired: 2 in, 2 out]
            n131 = call "labSSH_FGGA_Files_Transfer.vi"("Flight_num"=w346, "Get current?"=w347, "Date"=w345, "Flight Folder Path"=w344) -> ("error IO"=→"FGGA File Transfer Error out":errorcluster)  [unwired: 11 in]
          }
          frame #3 {
            n132 = local write "Transfer FGGA Files"(FALSE) -> ()
          }
        }
      }
      event "FGGA Restart": Value Change {
        n133 = event-data() -> ()  [unwired: 1 in, 6 out]
        n134 = flat-sequence {
          frame #0 {
            n135 = Two Button Dialog(message="FGGA will be restarted,\nARE YOU SURE?") -> (T button?=w357:bool)  [unwired: 2 in]
            n136 = case shown="True" w357 {
              frame False {
              }
              frame True {
                n137 = call "labSSH_Commands.vi"("Data"="reboot") -> ()  [unwired: 14 in, 1 out]
              }
            }
          }
          frame #1 {
            n138 = local write "FGGA Restart"(FALSE ("FGGA Restart")) -> ()
          }
        }
      }
      event "FGGA Shutdown": Value Change {
        n139 = event-data() -> ()  [unwired: 1 in, 6 out]
        n140 = flat-sequence {
          frame #0 {
            n141 = Two Button Dialog(message="FGGA will be shutdown,\nARE YOU SURE?") -> (T button?=w361:bool)  [unwired: 2 in]
            n142 = case shown="True" w361 {
              frame False {
              }
              frame True {
                n143 = call "labSSH_Commands.vi"("Data"="halt") -> ()  [unwired: 14 in, 1 out]
              }
            }
          }
          frame #1 {
            n144 = local write "FGGA Shutdown"(FALSE ("FGGA Restart")) -> ()
          }
        }
      }
    }
    n145 = node-c288() -> ()  [unwired: 1 in, 1 out]
  }
  n146 = local write "Network disconnected"(FALSE ("Network disconnect")) -> ()
  n147 = while {
    shift-right: [w485] -> _
    shift-left: w11 -> [w483]
    shift-right: [w487] -> _
    shift-left: w10 -> [w488]
    shift-right: [w486] -> _
    shift-left: w12 -> [w490]
    shift-right: [w479] -> _
    shift-left: w12 -> [w481]
    shift-right: [w476] -> _
    shift-left: w11 -> [w475]
    shift-right: [w478] -> _
    shift-left: w10 -> [w480]
    stop <- FALSE stop-if-true
    w421 = ""
    w416 = "%s" ("format string")
    w607 = "%s" ("format string")
    w612 = "%s" ("format string")
    w617 = "%s" ("format string")
    w623 = "%s" ("format string")
    w629 = "%s" ("format string")
    w633 = "%s" ("format string")
    # "UDP Data Processing"
    n148 = local read "CHFGGA01"() -> (w636:string)
    n149 = local read "TWBOZO01"() -> (w611:string)
    n150 = local read "AL52CO01"() -> (w628:string)
    n151 = local read "CABOZO01"() -> (w616:string)
    n152 = local read "TEIOZO01"() -> (w622:string)
    n153 = local read "CHTSOO01"() -> (w606:string)
    n154 = local read "Ambient = OFF\nCabin = ON"() -> (w511:bool)
    n155 = Spreadsheet String To Array(delimiter (Tab)=",", format string=w633, spreadsheet string=w636, array type (2D Dbl)=string[] []) -> (array=w583:string[])
    n156 = Spreadsheet String To Array(delimiter (Tab)=",", format string=w629, spreadsheet string=w628, array type (2D Dbl)=string[] []) -> (array=w604:string[])
    n157 = Spreadsheet String To Array(delimiter (Tab)=",", format string=w617, spreadsheet string=w616, array type (2D Dbl)=string[] []) -> (array=w508:string[])
    n158 = Spreadsheet String To Array(delimiter (Tab)=",", format string=w623, spreadsheet string=w622, array type (2D Dbl)=string[] []) -> (array=w581:string[])
    n159 = Spreadsheet String To Array(delimiter (Tab)=",", format string=w612, spreadsheet string=w611, array type (2D Dbl)=string[] []) -> (array=w507:string[])
    n160 = Spreadsheet String To Array(delimiter (Tab)=",", format string=w607, spreadsheet string=w606, array type (2D Dbl)=string[] []) -> (array=w579:string[])
    n161 = Array To Spreadsheet String(delimiter (Tab)="\r", array=w583, 3:w633) -> (spreadsheet string=→"FGGA":string)
    n162 = Array To Spreadsheet String(delimiter (Tab)="\r", array=w604, 3:w629) -> (spreadsheet string=→"CO":string)
    n163 = Array To Spreadsheet String(delimiter (Tab)="\r", array=w508, 3:w617) -> (spreadsheet string=→"2B Cabin Ozone":string)
    n164 = Array To Spreadsheet String(delimiter (Tab)="\r", array=w581, 3:w623) -> (spreadsheet string=→"TEi49 Ozone":string)
    n165 = Array To Spreadsheet String(delimiter (Tab)="\r", array=w507, 3:w612) -> (spreadsheet string=→"2B Ambient Ozone":string)
    n166 = Array To Spreadsheet String(delimiter (Tab)="\r", array=w579, 3:w607) -> (spreadsheet string=→"SO2":string)
    n167 = Select(t=w508, s=w511, f=w507) -> (s? t:f=w506:string[])
    n168 = Index Array(array=w579, index #1=6 ("index"), index #2=4 ("index"), index #3=3 ("index"), index #4=7 ("index"), index #5=8 ("index"), index #6=15 ("index"), index #7=24 ("index"), index #8=29 ("index"), index #9=36 ("index"), index #10=37 ("index"), index #11=38 ("index"), index #12=39 ("index"), index #13=48 ("index"), index #14=14 ("index")) -> (element #1=w498:string, element #2=w562:string, element #3=w557:string, element #4=w550:string, element #5=w526:string, element #6=w525:string, element #7=w439:string, element #8=w438:string, element #9=w387:string, element #10=w383:string, element #11=w379:string, element #12=w377:string, element #13=w369:string, element #14=w367:string)
    n169 = Index Array(array=w506, index #1=8 ("index"), index #2=11 ("index")) -> (element #1=w500:string, element #2=w501:string)
    n170 = Index Array(array=w581, index #1=6 ("index"), index #2=4 ("index"), index #3=3 ("index"), index #4=7 ("index"), index #5=9 ("index"), index #6=14 ("index"), index #7=15 ("index")) -> (element #1=w575:string, element #2=w563:string, element #3=w558:string, element #4=w543:string, element #5=w517:string, element #6=w516:string, element #7=w515:string)
    n171 = Scan Value(string=w500, format string="%f") -> (value=→"2B Ozone concentration":dbl)  [unwired: 1 in, 1 out]
    n172 = Scan Value(string=w501, format string="%4f") -> (value=→"2B Ozone flow rate":dbl)  [unwired: 1 in, 1 out]
    n173 = Index Array(array=w583, index #1=6 ("index"), index #2=4 ("index"), index #3=3 ("index"), index #4=7 ("index"), index #5=8 ("index"), index #6=9 ("index"), index #7=10 ("index"), index #8=17 ("index"), index #9=16 ("index"), index #10=11 ("index"), index #11=12 ("index"), index #12=21 ("index"), index #13=14 ("index"), index #14=15 ("index")) -> (element #1=w577:string, element #2=w565:string, element #3=w560:string, element #4=w545:string, element #5=w463:string, element #6=w460:string, element #7=w455:string, element #8=w453:string, element #9=w450:string, element #10=w445:string, element #11=w444:string, element #12=w431:string, element #13=w397:string, element #14=w396:string)
    n174 = Index Array(array=w604, index #1=2 ("index"), index #2=27 ("index"), index #3=28 ("index"), index #4=29 ("index"), index #5=30 ("index"), index #6=31 ("index"), index #7=6 ("index"), index #8=4 ("index"), index #9=3 ("index"), index #10=8 ("index"), index #11=14 ("index"), index #12=16 ("index"), index #13=19 ("index"), index #14=12 ("index"), index #15=13 ("index"), index #16=10 ("index"), index #17=11 ("index"), index #18=15 ("index")) -> (element #1=w473:string, element #2=w547:string, element #3=w594:string, element #4=w588:string, element #5=w586:string, element #6=w587:string, element #7=w576:string, element #8=w564:string, element #9=w559:string, element #10=w548:string, element #11=w535:string, element #12=w532:string, element #13=w531:string, element #14=w493:string, element #15=w492:string, element #16=w427:string, element #17=w408:string, element #18=w402:string)
    n175 = Scan Value(string=w369, format string="%f") -> (value=→"Calibration gas cylinder \nconcentration (ppb)":dbl)  [unwired: 1 in, 1 out]
    n176 = Scan Value(string=w439, format string="%f") -> (value=→"TEI43i MFC2 Cal Flow":dbl)  [unwired: 1 in, 1 out]
    n177 = Scan Value(string=w438, format string="%f") -> (value=→"TEI43i MFC3 Sample Flow":dbl)  [unwired: 1 in, 1 out]
    n178 = Scan Value(string=w387, format string="%f") -> (value=w373:dbl)  [unwired: 1 in, 1 out]
    n179 = Scan Value(string=w383, format string="%d", default (0 dbl)=0) -> (value=w381:i32)  [unwired: 1 out]
    n180 = Scan Value(string=w367, format string="%f") -> (value=→"SO2 react pressure":dbl)  [unwired: 1 in, 1 out]
    n181 = Scan Value(string=w377, format string="%f") -> (value=→"SO2 Sensitivity":dbl)  [unwired: 1 in, 1 out]
    n182 = Scan Value(string=w379, format string="%f") -> (value=→"SO2 Zero":dbl)  [unwired: 1 in, 1 out]
    n183 = Scan Value(string=w526, format string="%f") -> (value=w374:dbl)  [unwired: 1 in, 1 out]
    n184 = Scan Value(string=w525, format string="%f") -> (value=→"TEI43C Sample Flow":dbl)  [unwired: 1 in, 1 out]
    n185 = Not Equal To 0?(x=w381) -> (x != 0?=→"mean zero\ncal status":bool)
    n186 = Decimal String To Number(string=w473) -> (number=w471:i32)  [unwired: 2 in, 1 out]
    n187 = call "Find_Data_SubVI.vi"("FGGA"=w577, "CO"=w576, "Ozone"=w575, "SO2"=w498) -> ("Output Value"=→"CPU Total %":dbl)  [unwired: 11 in]
    n188 = call "Find_Data_SubVI.vi"("FGGA"=w565, "CO"=w564, "Ozone"=w563, "SO2"=w562) -> ("Output Value"=→"MFM":dbl)  [unwired: 11 in]
    n189 = call "Find_Data_SubVI.vi"("FGGA"=w560, "CO"=w559, "Ozone"=w558, "SO2"=w557) -> ("Output Value"=w556:dbl)  [unwired: 11 in]
    n190 = call "Find_Data_SubVI.vi"("FGGA"=w545, "CO"=w548, "Ozone"=w543, "SO2"=w550) -> ("Output Value"=→"USB Disk Space Used %":dbl)  [unwired: 11 in]
    n191 = Not Equal To 0?(x=w556) -> (x != 0?=→"PTP Sync":bool)
    n192 = Add(x=w471, y=u32 2082844800) -> (x+y=w470:u32)
    n193 = Scan Value(string=w431, format string="%f") -> (value=→"MFC1 Cal Flow":dbl)  [unwired: 1 in, 1 out]
    n194 = Scan Value(string=w397, format string="%f") -> (value=w395:dbl)  [unwired: 1 in, 1 out]
    n195 = Scan Value(string=w396, format string="%f") -> (value=w393:dbl)  [unwired: 1 in, 1 out]
    n196 = Scan Value(string=w444, format string="%f") -> (value=→"Cell temperature":dbl)  [unwired: 1 in, 1 out]
    n197 = Scan Value(string=w445, format string="%f") -> (value=→"Cell pressure":dbl)  [unwired: 1 in, 1 out]
    n198 = Scan Value(string=w450, format string="%f") -> (value=→"CH4 Dry":dbl)  [unwired: 1 in, 1 out]
    n199 = Scan Value(string=w453, format string="%f") -> (value=→"CO2 Dry":dbl)  [unwired: 1 in, 1 out]
    n200 = Scan Value(string=w455, format string="%f") -> (value=→"H2O":dbl)  [unwired: 1 in, 1 out]
    n201 = Scan Value(string=w460, format string="%f") -> (value=→"CO2":dbl)  [unwired: 1 in, 1 out]
    n202 = Scan Value(string=w463, format string="%f") -> (value=→"CH4":dbl)  [unwired: 1 in, 1 out]
    n203 = local read "PRTAFT_UDP_In"() -> (w414:string)
    n204 = Scan Value(string=w587, format string="%f") -> (value=→"Std\nContent (barG)":dbl)  [unwired: 1 in, 1 out]
    n205 = Scan Value(string=w547, format string="%d", default (0 dbl)=u32 0) -> (value=w601:u32)  [unwired: 1 out]
    n206 = Scan Value(string=w586, format string="%f") -> (value=→"N2\nContent (barG)":dbl)  [unwired: 1 in, 1 out]
    n207 = Scan Value(string=w588, format string="%f") -> (value=→"CO2\nContent (barG)":dbl)  [unwired: 1 in, 1 out]
    n208 = Scan Value(string=w594, format string="%f") -> (value=→"CO2 Pressure\nDelivery (PSIA)":dbl)  [unwired: 1 in, 1 out]
    n209 = Bundle(w374, w373) -> (→"TEi43i Concentration scaled / raw":cluster{dbl, dbl})  [unwired: 1 in]
    n210 = To Time Stamp(1:w470) -> (0:w474:timestamp)
    n211 = Scan Value(string=w535, format string="%f") -> (value=→"Lamp Flow Controller":dbl)  [unwired: 1 in, 1 out]
    n212 = Scan Value(string=w408, format string="%f") -> (value=→"Raw Signal":dbl)  [unwired: 1 in, 1 out]
    n213 = Scan Value(string=w402, format string="%f") -> (value=→"Lamp Temperature":dbl)  [unwired: 1 in, 1 out]
    n214 = Scan Value(string=w427, format string="%f") -> (value=→"CO Concentration":dbl)  [unwired: 1 in, 1 out]
    n215 = Scan Value(string=w532, format string="%f") -> (value=→"Monochromator Flow":dbl)  [unwired: 1 in, 1 out]
    n216 = Scan Value(string=w531, format string="%f") -> (value=→"Fluorescence Cell Pressure":dbl)  [unwired: 1 in, 1 out]
    n217 = Not Equal To 0?(x=w601) -> (x != 0?=→"CO CAL Status":bool)
    n218 = Scan Value(string=w515, format string="%f") -> (value=→"TEI49 Sample Flow B":dbl)  [unwired: 1 in, 1 out]
    n219 = Scan Value(string=w517, format string="%f") -> (value=→"TEi49 Concentration":dbl)  [unwired: 1 in, 1 out]
    n220 = Scan Value(string=w516, format string="%f") -> (value=→"TEI49 Sample Flow A":dbl)  [unwired: 1 in, 1 out]
    n221 = Scan Value(string=w493, format string="%f") -> (value=w484:dbl)  [unwired: 1 in, 1 out]
    n222 = Scan Value(string=w492, format string="%f") -> (value=w477:dbl)  [unwired: 1 in, 1 out]
    n223 = Not Equal?(x=w483, y=w484) -> (x != y?=w489:bool)
    n224 = Not Equal?(x=w475, y=w477) -> (x != y?=w482:bool)
    n225 = Spreadsheet String To Array(delimiter (Tab)=",", format string=w416, spreadsheet string=w414, array type (2D Dbl)=string[] []) -> (array=w415:string[])
    n226 = case shown="True" w489 {
      tunnel: w490 -> [w657 w666]
      tunnel: w488 -> [w658 w665]
      tunnel: [w658 w664] -> w487
      tunnel: w474 -> [_ w660]
      tunnel: w484 -> [_ w661]
      tunnel: [w657 w663] -> w486
      tunnel: [w656 w662] -> w485
      tunnel: w484 -> [_ w662]
      tunnel: w483 -> [w656 _]
      frame False {
      }
      frame True {
        n227 = Bundle(w660, w661) -> (w659:cluster{timestamp, dbl})  [unwired: 1 in]
        n228 = Replace Array Subset(array=w666, new element=w659, index=w665) -> (w663:cluster{"time stamp":timestamp, "Y":dbl}[])
        n229 = Increment(x=w665) -> (x+1=w664:i32)
      }
    }
    "CO Sensitivity" <- w486
    n230 = case shown="True" w482 {
      tunnel: w481 -> [w646 w655]
      tunnel: w480 -> [w647 w654]
      tunnel: [w647 w653] -> w478
      tunnel: w474 -> [_ w652]
      tunnel: w477 -> [_ w651]
      tunnel: [w646 w650] -> w479
      tunnel: [w645 w649] -> w476
      tunnel: w477 -> [_ w649]
      tunnel: w475 -> [w645 _]
      frame False {
      }
      frame True {
        n231 = Bundle(w652, w651) -> (w648:cluster{timestamp, dbl})  [unwired: 1 in]
        n232 = Replace Array Subset(array=w655, new element=w648, index=w654) -> (w650:cluster{"time stamp":timestamp, "Y":dbl}[])
        n233 = Increment(x=w654) -> (x+1=w653:i32)
      }
    }
    "CO Zero" <- w479
    n234 = Array To Spreadsheet String(delimiter (Tab)="\r", array=w415, 3:w416) -> (spreadsheet string=→"PRTAFT_DLU":string)
    n235 = Index Array(array=w415, index #1=5 ("index"), index #2=19 ("index")) -> (element #1=w419:string, element #2=w417:string)
    n236 = Not Equal?(x=w419, y=w421) -> (x != y?=w420:bool)
    n237 = Not Equal?(x=w417, y=w421) -> (x != y?=w418:bool)
    n238 = Bundle(w395, w393) -> (→"Ring Down Time RDA & RDB":cluster{dbl, dbl})  [unwired: 1 in]
    n239 = case shown="False" w418 {
      tunnel: ["1" w642] -> w411
      tunnel: w417 -> [_ w642]
      frame False {
      }
      frame True {
      }
    }
    n240 = case shown="False" w420 {
      tunnel: ["XXXX" w644] -> w412
      tunnel: w419 -> [_ w644]
      frame False {
      }
      frame True {
      }
    }
    n241 = Wait (ms)(milliseconds to wait=u32 1000) -> ()  [unwired: 1 out]
    n242 = local write "WoW Flag"(w411) -> ()
    n243 = local write "Flight Number"(w412) -> ()
  }
  n244 = while {
    stop <- FALSE stop-if-true
    # "Check Connection with the cRIO continuously"
    n245 = node-c288() -> (w668:T6)  [unwired: 4 in]
    n246 = TCP Open Connection(address="192.168.101.17", remote port or service name=u16 7001) -> (connection ID=w677:refnum<k5>, error out=w678:errorcluster)  [unwired: 3 in]
    n247 = timed-loop {
      tunnel: w678 -> [w693]
      tunnel: w677 -> [w690]
      tunnel: [w686] -> w670
      tunnel: [w687] -> w674
      shift-right: [w682] -> _
      shift-left: FALSE -> [w683]
      timing: w668 -> [_]
      timing-out: [_] -> w667
      stop <- w686 stop-if-true
      # "Maintain live connecton to cRIO for connection watchdog"
      n248 = node-c288() -> ()  [unwired: 1 in, 1 out]
      n249 = TCP Write(connection ID=w690, data in="1", error in (no error)=w693, 9:2000 ("timeout ms (25000)")) -> (connection ID out=w691:refnum<k5>, bytes written=w688:i32, error out=w692:errorcluster)
      n250 = Select(t=FALSE, s=w683, f=TRUE) -> (s? t:f=w682:bool)
      "cRIO connection status" <- w682
      n251 = local write "Network disconnected"(FALSE ("Network disconnect")) -> ()
      n252 = TCP Read(connection ID=w691, bytes to read=w688, error in (no error)=w692, 9:2000 ("timeout ms (25000)")) -> (connection ID out=w687:refnum<k5>, error out=w686:errorcluster)  [unwired: 1 in, 1 out]
      n253 = node-c288() -> ()  [unwired: 1 in, 1 out]
    }
    n254 = node-c288(w667) -> ()  [unwired: 1 out]
    n255 = TCP Close Connection(connection ID=w674, error in (no error)=w670) -> (error out=w669:errorcluster)  [unwired: 1 in, 1 out]
    "Network Check error out" <- w669
    n256 = Unbundle By Name(w669) -> ("status"=w671:bool)
    "Network disconnected" <- w671
    n257 = case shown="True" w671 {
      frame False {
      }
      frame True {
        n258 = One Button Dialog(message="Connection to cRIO lost\nAll Calibration(s) will be terminated") -> ()  [unwired: 1 in, 1 out]
      }
    }
  }
  n259 = while {
    stop <- FALSE stop-if-true
    # "Preflight Sub VI Descriptions"
    n260 = Wait (ms)(milliseconds to wait=u32 500) -> ()  [unwired: 1 out]
    n261 = case shown="True" "Line Lock Setting Change" {
      frame False {
      }
      frame True {
        n262 = call "FGGA Linelock Settings Procedures.vi"() -> ()  [unwired: 12 in]
      }
    }
  }
  n263 = while {
    stop <- FALSE stop-if-true
    # "Postflight Sub VI Descriptions"
    n264 = case shown="True" "Postflight Procedures" {
      frame False {
      }
      frame True {
        n265 = call "PostFlight Procedures.vi"() -> ()  [unwired: 12 in]
      }
    }
    n266 = Wait (ms)(milliseconds to wait=u32 500) -> ()  [unwired: 1 out]
  }
  n267 = while {
    stop <- FALSE stop-if-true
    # "Preflight Sub VI Descriptions"
    n268 = case shown="True" "Prepare Gases" {
      frame False {
      }
      frame True {
        n269 = call "CO Gas Preparation.vi"() -> ()  [unwired: 12 in]
      }
    }
    n270 = Wait (ms)(milliseconds to wait=u32 500) -> ()  [unwired: 1 out]
  }
  n271 = while {
    stop <- FALSE stop-if-true
    # "Preflight Sub VI Descriptions"
    n272 = case shown="True" "Prepare SO2 Span Gas" {
      frame False {
      }
      frame True {
        n273 = call "SO2 Span Gas Preparation.vi"() -> ()  [unwired: 12 in]
      }
    }
    n274 = Wait (ms)(milliseconds to wait=u32 500) -> ()  [unwired: 1 out]
  }
  n275 = while {
    stop <- FALSE stop-if-true
    # "Preflight Sub VI Descriptions"
    n276 = case shown="True" "Prepare SO2 Zero Gas" {
      frame False {
      }
      frame True {
        n277 = call "SO2 ZeroAir Gas Preparation.vi"() -> ()  [unwired: 12 in]
      }
    }
    n278 = Wait (ms)(milliseconds to wait=u32 500) -> ()  [unwired: 1 out]
  }
  n279 = Obtain Queue(name (unnamed)="FGGA_Command", element data type=w56) -> (queue out=w6:refnum<queue>, error out=w5:errorcluster)  [unwired: 3 in, 1 out]
  n280 = while {
    stop <- FALSE stop-if-true
    # "Preflight Sub VI Descriptions"
    n281 = case shown="True" "CO Monitor Troubleshooting" {
      frame False {
      }
      frame True {
        n282 = call "CO Monitor Troubleshooting.vi"() -> ()  [unwired: 12 in]
      }
    }
    n283 = Wait (ms)(milliseconds to wait=u32 500) -> ()  [unwired: 1 out]
  }
  n284 = while {
    shift-right: [w720] -> _
    shift-left: u8 1 -> [w721]
    tunnel: w6 -> [w718]
    tunnel: w5 -> [w717]
    stop <- FALSE stop-if-true
    # "FGGA pump synchronise to WoW Wait on Wheel Flag"
    n285 = Wait (ms)(milliseconds to wait=u32 1000) -> ()  [unwired: 1 out]
    n286 = case shown="True" "FGGA pump\nsync to WoW" {
      tunnel: [w724 w729] -> w720
      tunnel: w721 -> [w724 w728]
      tunnel: w718 -> [_ w727]
      tunnel: w717 -> [_ w726]
      frame False {
      }
      frame True {
        n287 = local read "WoW Flag"() -> (w725:string)
        n288 = Scan Value(string=w725, format string="%d", default (0 dbl)=u8 0) -> (value=w729:u8)  [unwired: 1 out]
        n289 = Not Equal?(x=w729, y=w728) -> (x != y?=w732:bool)
        n290 = case shown="True" w732 {
          tunnel: w729 -> [_ w735]
          tunnel: w727 -> [_ w734]
          tunnel: w726 -> [_ w733]
          frame False {
          }
          frame True {
            n291 = Equal?(x=w735, y=u8 0) -> (x = y?=w740:bool)
            n292 = case shown="True" w740 {
              selector: w740 -> [w742 w743]
              tunnel: [w742 w743] -> w736
              frame False {
              }
              frame True {
              }
            }
            n293 = local write "Manual FGGA Pump"(w736) -> ()
            n294 = Bundle(cluster=T4 {"Message"="", "Message Data"=variant} ("Message Cluster"), "Message"="FGGA_pump", "Message Data"=w736) -> (w737:T4)
            n295 = Enqueue Element(queue=w734, element=w737, error in (no error)=w733) -> ()  [unwired: 1 in, 3 out]
          }
        }
      }
    }
  }
  n296 = while {
    tunnel: w6 -> [w745]
    tunnel: w5 -> [w744]
    tunnel: [w747] -> _
    tunnel: w16 -> [w746]
    stop <- FALSE stop-if-true
    # "FGGA UI Event Handler Loop"
    n297 = event shown="[9] \"Span Cal -  High Cal, CO Cal, Low Cal\": Value Change" {
      selector: _ -> [_ _ _ _ _ _ _ _ _ _ _ _ _ _ _ _ _]
      dyn-events: _ -> [_ _ _ _ _ _ _ _ _ _ _ _ _ _ _ _ _]
      timeout: _ -> [_ _ _ _ _ _ _ _ _ _ _ _ _ _ _ _ _]
      tunnel: w745 -> [w755 w759 w766 w773 w780 w788 w802 w809 w824 w965 w1216 w1286 w1356 w1412 w1526 w1625 w1632]
      tunnel: w744 -> [w754 w758 w765 w772 w779 w787 w801 w808 w823 w964 w1215 w1285 w1355 w1411 w1525 w1624 w1631]
      tunnel: [w749 w757 w764 w771 w778 w786 w800 w807 w814 w938 w1208 w1278 w1348 w1402 w1518 w1623 w1630] -> w747
      tunnel: w746 -> [_ _ _ _ _ _ _ _ _ w952 _ _ _ _ _ _ _]
      event "eV1": Value Change {
        n298 = event-data() -> ("NewVal"=w752:bool)  [unwired: 1 in]
        n299 = Bundle(cluster=T4 {"Message"="", "Message Data"=variant} ("Message Cluster"), "Message"="V1", "Message Data"=w752) -> (w750:T4)
        n300 = Enqueue Element(queue=w755, element=w750, error in (no error)=w754) -> (error out=w749:errorcluster)  [unwired: 1 in, 2 out]
      }
      event "eV2": Value Change {
        n301 = event-data() -> ("NewVal"=w756:bool)  [unwired: 1 in]
        n302 = Bundle(cluster=T4 {"Message"="", "Message Data"=variant} ("Message Cluster"), "Message"="V2", "Message Data"=w756) -> (w760:T4)
        n303 = Enqueue Element(queue=w759, element=w760, error in (no error)=w758) -> (error out=w757:errorcluster)  [unwired: 1 in, 2 out]
      }
      event "eV3": Value Change {
        n304 = event-data() -> ("NewVal"=w763:bool)  [unwired: 1 in]
        n305 = Bundle(cluster=T4 {"Message"="", "Message Data"=variant} ("Message Cluster"), "Message"="V3", "Message Data"=w763) -> (w767:T4)
        n306 = Enqueue Element(queue=w766, element=w767, error in (no error)=w765) -> (error out=w764:errorcluster)  [unwired: 1 in, 2 out]
      }
      event "eV4": Value Change {
        n307 = event-data() -> ("NewVal"=w770:bool)  [unwired: 1 in]
        n308 = Bundle(cluster=T4 {"Message"="", "Message Data"=variant} ("Message Cluster"), "Message"="V4", "Message Data"=w770) -> (w774:T4)
        n309 = Enqueue Element(queue=w773, element=w774, error in (no error)=w772) -> (error out=w771:errorcluster)  [unwired: 1 in, 2 out]
      }
      event "Manual FGGA Pump": Value Change {
        n310 = event-data() -> ("NewVal"=w777:bool)  [unwired: 1 in]
        n311 = Bundle(cluster=T4 {"Message"="", "Message Data"=variant} ("Message Cluster"), "Message"="FGGA_pump", "Message Data"=w777) -> (w781:T4)
        n312 = Enqueue Element(queue=w780, element=w781, error in (no error)=w779) -> (error out=w778:errorcluster)  [unwired: 1 in, 2 out]
      }
      event "Confirm Flight Number": Value Change {
        n313 = event-data() -> ()  [unwired: 1 in, 6 out]
        n314 = flat-sequence {
          tunnel: w787 -> [w790]
          tunnel: w788 -> [w791]
          tunnel: [w791] -> w785
          tunnel: [w790] -> w784
          tunnel: [w793] -> w786
          tunnel: w785 -> [w795]
          tunnel: w784 -> [w794]
          frame #0 {
            n315 = local write "cRIO File IO Stop\n(USB Flash Drive Unmount)"(FALSE ("cRIO File IO Stop\n(USB Flash Drive Unmount)")) -> ()
          }
          frame #1 {
            n316 = local read "Flight Number"() -> (w792:string)
            n317 = Bundle(cluster=T4 {"Message"="", "Message Data"=variant} ("Message Cluster"), "Message"="Flight Number", "Message Data"=w792) -> (w796:T4)
            n318 = Enqueue Element(queue=w795, element=w796, error in (no error)=w794) -> (error out=w793:errorcluster)  [unwired: 1 in, 2 out]
          }
        }
      }
      event "FGGA Restart": Value Change {
        n319 = event-data() -> ("NewVal"=w799:bool)  [unwired: 1 in]
        n320 = Bundle(cluster=T4 {"Message"="", "Message Data"=variant} ("Message Cluster"), "Message"="FGGA_restart", "Message Data"=w799) -> (w803:T4)
        n321 = Enqueue Element(queue=w802, element=w803, error in (no error)=w801) -> (error out=w800:errorcluster)  [unwired: 1 in, 2 out]
      }
      event "cRIO File IO Stop\n(USB Flash Drive Unmount)": Value Change {
        n322 = event-data() -> ("NewVal"=w806:bool)  [unwired: 1 in]
        n323 = Bundle(cluster=T4 {"Message"="", "Message Data"=variant} ("Message Cluster"), "Message"="Stop File Write", "Message Data"=w806) -> (w810:T4)
        n324 = Enqueue Element(queue=w809, element=w810, error in (no error)=w808) -> (error out=w807:errorcluster)  [unwired: 1 in, 2 out]
      }
      event "High Cal": Value Change {
        n325 = event-data() -> ()  [unwired: 1 in, 1 out]
        n326 = flat-sequence {
          tunnel: w824 -> [w829]
          tunnel: w823 -> [w828]
          tunnel: [w827] -> w822
          tunnel: [w826] -> w821
          tunnel: w822 -> [w845]
          tunnel: w821 -> [w844]
          tunnel: [w842] -> w820
          tunnel: [w841] -> w819
          tunnel: [w849] -> w818
          tunnel: [w850] -> w817
          tunnel: w819 -> [w854]
          tunnel: w820 -> [w853]
          tunnel: w818 -> [w907]
          tunnel: w817 -> [w906]
          tunnel: [w904] -> w816
          tunnel: [w903] -> w815
          tunnel: w816 -> [w921]
          tunnel: w815 -> [w920]
          tunnel: [w918] -> w813
          tunnel: [w926] -> w814
          tunnel: w813 -> [w926]
          frame #0 {
            w825 = TRUE
            n327 = Cluster To Array(cluster=T11 {"Message"="V2", "Message 2"="V3", "Message 3"="V4"}) -> (array=w830:string[])
            n328 = for {
              tunnel: w830 -> [w837] mode=indexing
              tunnel: w829 -> [w836]
              tunnel: w828 -> [w835]
              tunnel: [w834] -> w827
              tunnel: [w833] -> w826
              tunnel: w825 -> [w832]
              n329 = Bundle(cluster=T4 {"Message"="", "Message Data"=variant} ("Message Cluster"), "Message"=w837, "Message Data"=w832) -> (w839:T4)
              n330 = Enqueue Element(queue=w836, element=w839, error in (no error)=w835) -> (queue out=w834:refnum<queue>, error out=w833:errorcluster)  [unwired: 1 in, 1 out]
            }
            n331 = local write "eV2"(w825) -> ()
            n332 = local write "eV4"(w825) -> ()
            n333 = local write "eV3"(w825) -> ()
          }
          frame #1 {
            n334 = local read "MFC_1 User Set Value"() -> (w840:dbl)
            n335 = local write "MFC_1\nSLPM Value"(w840) -> ()
            n336 = Bundle(cluster=T4 {"Message"="", "Message Data"=variant} ("Message Cluster"), "Message"="MFC_1", "Message Data"=w840) -> (w843:T4)
            n337 = Enqueue Element(queue=w845, element=w843, error in (no error)=w844) -> (queue out=w842:refnum<queue>, error out=w841:errorcluster)  [unwired: 1 in, 1 out]
          }
          frame #2 {
            n338 = for {
              N: 45 -> [w897]
              tunnel: w854 -> [w887]
              tunnel: w853 -> [w888]
              tunnel: [w888] -> w852
              tunnel: [w887] -> w851
              tunnel: [w886] -> w848
              i -> [w896]
              stop <- w886 stop-if-true
              n339 = Subtract(x=w897, y=w896) -> (x-y=w895:i32)
              n340 = Decrement(x=w895) -> (x-1=w894:i32)
              n341 = local read "FGGA Calibration Abort"() -> (w891:bool)
              n342 = case shown="True" w891 {
                selector: w891 -> [w900 _]
                tunnel: [w900 w901] -> w889
                frame False {
                }
                frame True {
                  n343 = Two Button Dialog(message="Are you sure to abort FGGA High Cal?") -> (T button?=w901:bool)  [unwired: 2 in]
                }
              }
              n344 = Wait (ms)(milliseconds to wait=u32 1000) -> ()  [unwired: 1 out]
              n345 = local read "Network disconnected"() -> (w890:bool)
              n346 = Or(x=w890, y=w889) -> (x .or. y?=w886:bool)
              n347 = case shown="False" w889 {
                selector: w889 -> [w899 _]
                frame False {
                  n348 = local write "FGGA Calibration Abort"(w899) -> ()
                }
                frame True {
                }
              }
              n349 = Select(t=0, s=w886, f=w894) -> (s? t:f=→"High Cal\nFlush Time Remain (sec)":i32)
            }
            n350 = case shown="False" w848 {
              tunnel: w852 -> [w861 w885]
              tunnel: w851 -> [w860 w884]
              tunnel: [w857 w884] -> w850
              tunnel: [w856 w885] -> w849
              frame False {
                w862 = TRUE
                # "Carry on if connection to cRIO is made\nor calibration not abort"
                n351 = Bundle(cluster=T4 {"Message"="", "Message Data"=variant} ("Message Cluster"), "Message"="V1", "Message Data"=w862) -> (w863:T4)
                n352 = local write "eV1"(w862) -> ()
                n353 = Enqueue Element(queue=w861, element=w863, error in (no error)=w860) -> (queue out=w858:refnum<queue>, error out=w859:errorcluster)  [unwired: 1 in, 1 out]
                n354 = for {
                  N: 60 -> [w878]
                  tunnel: w859 -> [w868]
                  tunnel: w858 -> [w867]
                  tunnel: [w868] -> w857
                  tunnel: [w867] -> w856
                  i -> [w877]
                  stop <- w869 stop-if-true
                  n355 = local read "FGGA Calibration Abort"() -> (w872:bool)
                  n356 = Subtract(x=w878, y=w877) -> (x-y=w876:i32)
                  n357 = case shown="True" w872 {
                    selector: w872 -> [w881 _]
                    tunnel: [w881 w882] -> w870
                    frame False {
                    }
                    frame True {
                      n358 = Two Button Dialog(message="Are you sure to abort FGGA High Cal?") -> (T button?=w882:bool)  [unwired: 2 in]
                    }
                  }
                  n359 = local read "Network disconnected"() -> (w871:bool)
                  n360 = Wait (ms)(milliseconds to wait=u32 1000) -> ()  [unwired: 1 out]
                  n361 = Decrement(x=w876) -> (x-1=w873:i32)
                  n362 = Or(x=w871, y=w870) -> (x .or. y?=w869:bool)
                  n363 = case shown="False" w870 {
                    selector: w870 -> [w880 _]
                    frame False {
                      n364 = local write "FGGA Calibration Abort"(w880) -> ()
                    }
                    frame True {
                    }
                  }
                  n365 = Select(t=0, s=w869, f=w873) -> (s? t:f=→"High Cal\nCal Time Remain (sec)":i32)
                }
              }
              frame True {
              }
            }
          }
          frame #3 {
            w905 = FALSE
            n366 = Cluster To Array(cluster=T12 {"Message"="V2", "Message 2"="V3", "Message 3"="V4", "Message 4"="V1"}) -> (array=w908:string[])
            n367 = for {
              tunnel: w908 -> [w915] mode=indexing
              tunnel: [w914] -> w904
              tunnel: [w913] -> w903
              tunnel: w905 -> [w912]
              tunnel: w907 -> [w911]
              tunnel: w906 -> [w910]
              n368 = Bundle(cluster=T4 {"Message"="", "Message Data"=variant} ("Message Cluster"), "Message"=w915, "Message Data"=w912) -> (w917:T4)
              n369 = Enqueue Element(queue=w911, element=w917, error in (no error)=w910) -> (queue out=w914:refnum<queue>, error out=w913:errorcluster)  [unwired: 1 in, 1 out]
            }
            n370 = local write "eV2"(w905) -> ()
            n371 = local write "eV4"(w905) -> ()
            n372 = local write "eV3"(w905) -> ()
            n373 = local write "eV1"(w905) -> ()
          }
          frame #4 {
            w919 = 0.0 ("MFC_1\nSLPM Value")
            n374 = local write "MFC_1\nSLPM Value"(w919) -> ()
            n375 = Bundle(cluster=T4 {"Message"="", "Message Data"=variant} ("Message Cluster"), "Message"="MFC_1", "Message Data"=w919) -> (w923:T4)
            n376 = Enqueue Element(queue=w921, element=w923, error in (no error)=w920) -> (error out=w918:errorcluster)  [unwired: 1 in, 2 out]
          }
          frame #5 {
            w925 = FALSE ("High Cal")
            n377 = local write "High Cal"(w925) -> ()
            n378 = local write "FGGA Calibration Abort"(w925) -> ()
          }
        }
      }
      event "Span Cal - \nHigh Cal, CO Cal, Low Cal": Value Change {
        n379 = event-data() -> ()  [unwired: 1 in, 1 out]
        n380 = flat-sequence {
          tunnel: w965 -> [w971]
          tunnel: w964 -> [w970]
          tunnel: [w969] -> w963
          tunnel: [w968] -> w962
          tunnel: w963 -> [w987]
          tunnel: w962 -> [w986]
          tunnel: [w984] -> w960
          tunnel: [w983] -> w958
          tunnel: [w993] -> w961
          tunnel: w960 -> [w993]
          tunnel: [w992] -> w959
          tunnel: w958 -> [w992]
          tunnel: [w990] -> w937
          tunnel: [w990] -> w934
          tunnel: w961 -> [w1011]
          tunnel: w959 -> [w1012]
          tunnel: [w1012] -> w944
          tunnel: w952 -> [w1013]
          tunnel: [w1013] -> w942
          tunnel: [w1011] -> w940
          tunnel: w937 -> [w1010]
          tunnel: [w1009] -> w935
          tunnel: w934 -> [w1009]
          tunnel: w944 -> [w1023]
          tunnel: [w1023] -> w943
          tunnel: w942 -> [w1022]
          tunnel: [w1022] -> w941
          tunnel: w940 -> [w1020]
          tunnel: [w1020] -> w939
          tunnel: [w1019] -> w936
          tunnel: w935 -> [w1019]
          tunnel: [w1027] -> w957
          tunnel: [w1026] -> w956
          tunnel: w939 -> [w1028]
          tunnel: w941 -> [w1034]
          tunnel: w943 -> [w1029]
          tunnel: w936 -> [w1025]
          tunnel: [w1025] -> w930
          tunnel: [w1024] -> w927
          tunnel: w957 -> [w1073]
          tunnel: w956 -> [w1072]
          tunnel: [w1070] -> w955
          tunnel: [w1069] -> w954
          tunnel: [w1068] -> w931
          tunnel: w930 -> [w1068]
          tunnel: [w1067] -> w928
          tunnel: w927 -> [w1067]
          tunnel: w955 -> [w1090]
          tunnel: w954 -> [w1089]
          tunnel: [w1087] -> w953
          tunnel: [w1086] -> w949
          tunnel: [w1085] -> w932
          tunnel: w931 -> [w1085]
          tunnel: [w1084] -> w929
          tunnel: w928 -> [w1084]
          tunnel: w953 -> [w1099]
          tunnel: [w1099] -> w951
          tunnel: [w1097] -> w950
          tunnel: w949 -> [w1097]
          tunnel: [w1096] -> w933
          tunnel: w932 -> [w1095]
          tunnel: w929 -> [w1094]
          tunnel: [w1104] -> w948
          tunnel: [w1103] -> w947
          tunnel: w951 -> [w1101]
          tunnel: w950 -> [w1102]
          tunnel: w933 -> [w1100]
          tunnel: w948 -> [w1186]
          tunnel: w947 -> [w1185]
          tunnel: [w1183] -> w946
          tunnel: [w1182] -> w945
          tunnel: w946 -> [w1201]
          tunnel: w945 -> [w1200]
          tunnel: [w1198] -> w938
          frame #0 {
            w967 = TRUE
            n381 = Cluster To Array(cluster=T11 {"Message"="V2", "Message 2"="V3", "Message 3"="V4"}) -> (array=w972:string[])
            n382 = for {
              tunnel: w972 -> [w979] mode=indexing
              tunnel: w971 -> [w978]
              tunnel: w970 -> [w977]
              tunnel: [w976] -> w969
              tunnel: [w975] -> w968
              tunnel: w967 -> [w974]
              n383 = Bundle(cluster=T4 {"Message"="", "Message Data"=variant} ("Message Cluster"), "Message"=w979, "Message Data"=w974) -> (w981:T4)
              n384 = Enqueue Element(queue=w978, element=w981, error in (no error)=w977) -> (queue out=w976:refnum<queue>, error out=w975:errorcluster)  [unwired: 1 in, 1 out]
            }
            n385 = local write "High Cal"(TRUE ("High Cal")) -> ()
            n386 = local write "eV2"(w967) -> ()
            n387 = local write "eV4"(w967) -> ()
            n388 = local write "eV3"(w967) -> ()
          }
          frame #1 {
            n389 = local read "MFC_1 User Set Value"() -> (w982:dbl)
            n390 = local write "MFC_1\nSLPM Value"(w982) -> ()
            n391 = Bundle(cluster=T4 {"Message"="", "Message Data"=variant} ("Message Cluster"), "Message"="MFC_1", "Message Data"=w982) -> (w985:T4)
            n392 = Enqueue Element(queue=w987, element=w985, error in (no error)=w986) -> (queue out=w984:refnum<queue>, error out=w983:errorcluster)  [unwired: 1 in, 1 out]
          }
          frame #2 {
            n393 = for {
              N: 45 -> [w1003]
              tunnel: [w995] -> w990
              i -> [w1002]
              stop <- w995 stop-if-true
              n394 = local read "FGGA Calibration Abort"() -> (w996:bool)
              n395 = case shown="True" w996 {
                selector: w996 -> [w1006 _]
                tunnel: [w1006 w1007] -> w994
                frame False {
                }
                frame True {
                  n396 = Two Button Dialog(message="Are you sure to abort FGGA Span Cal?") -> (T button?=w1007:bool)  [unwired: 2 in]
                }
              }
              n397 = local read "Network disconnected"() -> (w997:bool)
              n398 = Subtract(x=w1003, y=w1002) -> (x-y=w1001:i32)
              n399 = Decrement(x=w1001) -> (x-1=w999:i32)
              n400 = Wait (ms)(milliseconds to wait=u32 1000) -> ()  [unwired: 1 out]
              n401 = Or(x=w997, y=w994) -> (x .or. y?=w995:bool)
              n402 = case shown="False" w994 {
                selector: w994 -> [w1005 _]
                frame False {
                  n403 = local write "FGGA Calibration Abort"(w1005) -> ()
                }
                frame True {
                }
              }
              n404 = Select(t=0, s=w995, f=w999) -> (s? t:f=w998:i32)
              n405 = local write "High Cal\nFlush Time Remain (sec)"(w998) -> ()
            }
          }
          frame #3 {
            n406 = case shown="False" w1010 {
              tunnel: w1013 -> [w1014 _]
              frame False {
                # "CO Cal if no network\ndisconnect or abort cal"
                n407 = Bundle(cluster=T4 {"Message"="", "Message Data"=variant} ("Message Cluster"), "Message"="CO CAL", "Message Data"=TRUE) -> (w1016:T4)
                n408 = Enqueue Element(queue=w1014, element=w1016) -> ()  [unwired: 2 in, 3 out]
              }
              frame True {
              }
            }
          }
          frame #4 {
            # "To Ensure\nCO CAL\nis certain"
            n409 = Wait (ms)(milliseconds to wait=u32 1000) -> ()  [unwired: 1 out]
          }
          frame #5 {
            n410 = Bundle(cluster=T4 {"Message"="", "Message Data"=variant} ("Message Cluster"), "Message"="CO CAL", "Message Data"=FALSE) -> (w1030:T4)
            n411 = Enqueue Element(queue=w1034, element=w1030) -> ()  [unwired: 2 in, 3 out]
            n412 = case shown="False" w1025 {
              selector: w1025 -> [_ w1064]
              tunnel: w1029 -> [w1041 w1065]
              tunnel: w1028 -> [w1040 w1066]
              tunnel: [w1037 w1066] -> w1027
              tunnel: [w1036 w1065] -> w1026
              tunnel: [w1035 w1064] -> w1024
              frame False {
                w1045 = TRUE
                # "Carry on if connection to cRIO is made\nor calibration not abort"
                n413 = Bundle(cluster=T4 {"Message"="", "Message Data"=variant} ("Message Cluster"), "Message"="V1", "Message Data"=w1045) -> (w1044:T4)
                n414 = local write "eV1"(w1045) -> ()
                n415 = Enqueue Element(queue=w1040, element=w1044, error in (no error)=w1041) -> (queue out=w1039:refnum<queue>, error out=w1038:errorcluster)  [unwired: 1 in, 1 out]
                n416 = for {
                  N: 60 -> [w1058]
                  tunnel: w1039 -> [w1049]
                  tunnel: w1038 -> [w1048]
                  tunnel: [w1049] -> w1037
                  tunnel: [w1048] -> w1036
                  tunnel: [w1047] -> w1035
                  i -> [w1057]
                  stop <- w1047 stop-if-true
                  n417 = local read "FGGA Calibration Abort"() -> (w1052:bool)
                  n418 = case shown="True" w1052 {
                    selector: w1052 -> [w1061 _]
                    tunnel: [w1061 w1062] -> w1050
                    frame False {
                    }
                    frame True {
                      n419 = Two Button Dialog(message="Are you sure to abort FGGA Span Cal?") -> (T button?=w1062:bool)  [unwired: 2 in]
                    }
                  }
                  n420 = Subtract(x=w1058, y=w1057) -> (x-y=w1056:i32)
                  n421 = Decrement(x=w1056) -> (x-1=w1054:i32)
                  n422 = Wait (ms)(milliseconds to wait=u32 1000) -> ()  [unwired: 1 out]
                  n423 = local read "Network disconnected"() -> (w1051:bool)
                  n424 = Or(x=w1051, y=w1050) -> (x .or. y?=w1047:bool)
                  n425 = Select(t=0, s=w1047, f=w1054) -> (s? t:f=w1053:i32)
                  n426 = local write "High Cal\nCal Time Remain (sec)"(w1053) -> ()
                  n427 = case shown="False" w1050 {
                    selector: w1050 -> [w1060 _]
                    frame False {
                      n428 = local write "FGGA Calibration Abort"(w1060) -> ()
                    }
                    frame True {
                    }
                  }
                }
              }
              frame True {
              }
            }
          }
          frame #6 {
            w1071 = FALSE
            n429 = Cluster To Array(cluster=T12 {"Message"="V2", "Message 2"="V3", "Message 3"="V4", "Message 4"="V1"}) -> (array=w1074:string[])
            n430 = for {
              tunnel: w1074 -> [w1081] mode=indexing
              tunnel: [w1080] -> w1070
              tunnel: [w1079] -> w1069
              tunnel: w1071 -> [w1078]
              tunnel: w1073 -> [w1077]
              tunnel: w1072 -> [w1076]
              n431 = Bundle(cluster=T4 {"Message"="", "Message Data"=variant} ("Message Cluster"), "Message"=w1081, "Message Data"=w1078) -> (w1083:T4)
              n432 = Enqueue Element(queue=w1077, element=w1083, error in (no error)=w1076) -> (queue out=w1080:refnum<queue>, error out=w1079:errorcluster)  [unwired: 1 in, 1 out]
            }
            n433 = local write "eV2"(w1071) -> ()
            n434 = local write "eV4"(w1071) -> ()
            n435 = local write "eV3"(w1071) -> ()
            n436 = local write "eV1"(w1071) -> ()
          }
          frame #7 {
            w1088 = 0.0 ("MFC_1\nSLPM Value")
            n437 = local write "MFC_1\nSLPM Value"(w1088) -> ()
            n438 = Bundle(cluster=T4 {"Message"="", "Message Data"=variant} ("Message Cluster"), "Message"="MFC_1", "Message Data"=w1088) -> (w1092:T4)
            n439 = Enqueue Element(queue=w1090, element=w1092, error in (no error)=w1089) -> (queue out=w1086:refnum<queue>, error out=w1087:errorcluster)  [unwired: 1 in, 1 out]
          }
          frame #8 {
            n440 = local write "High Cal"(FALSE ("High Cal")) -> ()
            n441 = Or(x=w1095, y=w1094) -> (x .or. y?=w1096:bool)
          }
          frame #9 {
            n442 = case shown="False" w1100 {
              tunnel: [w1107 w1181] -> w1104
              tunnel: [w1106 w1180] -> w1103
              tunnel: w1102 -> [w1116 w1181]
              tunnel: w1101 -> [w1114 w1180]
              frame False {
                w1112 = TRUE
                n443 = Cluster To Array(cluster=cluster{"Message":string, "Message 3":string} {"Message"="V2", "Message 3"="V4"}) -> (array=w1117:string[])
                n444 = for {
                  tunnel: w1117 -> [w1160] mode=indexing
                  tunnel: w1116 -> [w1159]
                  tunnel: [w1158] -> w1118
                  tunnel: [w1157] -> w1120
                  tunnel: w1112 -> [w1156]
                  tunnel: w1114 -> [w1155]
                  n445 = Bundle(cluster=T4 {"Message"="", "Message Data"=variant} ("Message Cluster"), "Message"=w1160, "Message Data"=w1156) -> (w1162:T4)
                  n446 = Enqueue Element(queue=w1159, element=w1162, error in (no error)=w1155) -> (queue out=w1158:refnum<queue>, error out=w1157:errorcluster)  [unwired: 1 in, 1 out]
                }
                n447 = local write "eV4"(w1112) -> ()
                n448 = local write "eV2"(w1112) -> ()
                n449 = local write "Low Cal"(TRUE ("Low Cal")) -> ()
                n450 = local read "MFC_1 User Set Value"() -> (w1121:dbl)
                n451 = local write "MFC_1\nSLPM Value"(w1121) -> ()
                n452 = Bundle(cluster=T4 {"Message"="", "Message Data"=variant} ("Message Cluster"), "Message"="MFC_1", "Message Data"=w1121) -> (w1122:T4)
                n453 = Enqueue Element(queue=w1118, element=w1122, error in (no error)=w1120) -> (queue out=w1111:refnum<queue>, error out=w1109:errorcluster)  [unwired: 1 in, 1 out]
                n454 = for {
                  N: 45 -> [w1174]
                  tunnel: [w1165] -> w1110
                  tunnel: w1111 -> [w1165]
                  tunnel: [w1164] -> w1108
                  tunnel: w1109 -> [w1164]
                  tunnel: [w1163] -> w1105
                  i -> [w1173]
                  stop <- w1163 stop-if-true
                  n455 = local read "FGGA Calibration Abort"() -> (w1168:bool)
                  n456 = case shown="True" w1168 {
                    selector: w1168 -> [w1177 _]
                    tunnel: [w1177 w1178] -> w1166
                    frame False {
                    }
                    frame True {
                      n457 = Two Button Dialog(message="Are you sure to abort FGGA Span Cal?") -> (T button?=w1178:bool)  [unwired: 2 in]
                    }
                  }
                  n458 = Subtract(x=w1174, y=w1173) -> (x-y=w1172:i32)
                  n459 = Decrement(x=w1172) -> (x-1=w1169:i32)
                  n460 = Wait (ms)(milliseconds to wait=u32 1000) -> ()  [unwired: 1 out]
                  n461 = local read "Network disconnected"() -> (w1167:bool)
                  n462 = Or(x=w1167, y=w1166) -> (x .or. y?=w1163:bool)
                  n463 = Select(t=0, s=w1163, f=w1169) -> (s? t:f=w1170:i32)
                  n464 = local write "Low Cal\nFlush Time Remain (sec)"(w1170) -> ()
                  n465 = case shown="False" w1166 {
                    selector: w1166 -> [w1176 _]
                    frame False {
                      n466 = local write "FGGA Calibration Abort"(w1176) -> ()
                    }
                    frame True {
                    }
                  }
                }
                n467 = case shown="False" w1105 {
                  tunnel: w1110 -> [w1130 w1154]
                  tunnel: w1108 -> [w1129 w1153]
                  tunnel: [w1127 w1154] -> w1107
                  tunnel: [w1125 w1153] -> w1106
                  frame False {
                    w1131 = TRUE
                    n468 = local write "eV1"(w1131) -> ()
                    n469 = Bundle(cluster=T4 {"Message"="", "Message Data"=variant} ("Message Cluster"), "Message"="V1", "Message Data"=w1131) -> (w1133:T4)
                    n470 = Enqueue Element(queue=w1130, element=w1133, error in (no error)=w1129) -> (queue out=w1128:refnum<queue>, error out=w1126:errorcluster)  [unwired: 1 in, 1 out]
                    n471 = for {
                      N: 60 -> [w1147]
                      tunnel: [w1137] -> w1127
                      tunnel: w1128 -> [w1137]
                      tunnel: w1126 -> [w1136]
                      tunnel: [w1136] -> w1125
                      i -> [w1146]
                      stop <- w1138 stop-if-true
                      n472 = local read "FGGA Calibration Abort"() -> (w1141:bool)
                      n473 = case shown="True" w1141 {
                        selector: w1141 -> [w1150 _]
                        tunnel: [w1150 w1151] -> w1139
                        frame False {
                        }
                        frame True {
                          n474 = Two Button Dialog(message="Are you sure to abort FGGA Span Cal?") -> (T button?=w1151:bool)  [unwired: 2 in]
                        }
                      }
                      n475 = Wait (ms)(milliseconds to wait=u32 1000) -> ()  [unwired: 1 out]
                      n476 = local read "Network disconnected"() -> (w1140:bool)
                      n477 = Subtract(x=w1147, y=w1146) -> (x-y=w1145:i32)
                      n478 = Decrement(x=w1145) -> (x-1=w1142:i32)
                      n479 = Or(x=w1140, y=w1139) -> (x .or. y?=w1138:bool)
                      n480 = Select(t=0, s=w1138, f=w1142) -> (s? t:f=w1143:i32)
                      n481 = local write "Low Cal\nCal Time Remain (sec)"(w1143) -> ()
                      n482 = case shown="False" w1139 {
                        selector: w1139 -> [w1149 _]
                        frame False {
                          n483 = local write "FGGA Calibration Abort"(w1149) -> ()
                        }
                        frame True {
                        }
                      }
                    }
                  }
                  frame True {
                    # "Ignore Cal if connection problem or abort button pressed"
                  }
                }
              }
              frame True {
                # "Ignore Cal if connection problem or abort button pressed"
              }
            }
          }
          frame #10 {
            w1184 = FALSE
            n484 = Cluster To Array(cluster=T13 {"Message"="V2", "Message 3"="V4", "Message 4"="V1"}) -> (array=w1187:string[])
            n485 = local write "eV1"(w1184) -> ()
            n486 = local write "eV2"(w1184) -> ()
            n487 = local write "eV4"(w1184) -> ()
            n488 = for {
              tunnel: w1187 -> [w1194] mode=indexing
              tunnel: [w1193] -> w1183
              tunnel: [w1192] -> w1182
              tunnel: w1184 -> [w1191]
              tunnel: w1186 -> [w1190]
              tunnel: w1185 -> [w1189]
              n489 = Bundle(cluster=T4 {"Message"="", "Message Data"=variant} ("Message Cluster"), "Message"=w1194, "Message Data"=w1191) -> (w1196:T4)
              n490 = Enqueue Element(queue=w1190, element=w1196, error in (no error)=w1189) -> (queue out=w1193:refnum<queue>, error out=w1192:errorcluster)  [unwired: 1 in, 1 out]
            }
          }
          frame #11 {
            w1197 = FALSE
            w1199 = 0.0 ("MFC_1\nSLPM Value")
            n491 = local write "MFC_1\nSLPM Value"(w1199) -> ()
            n492 = local write "Span Cal - \nHigh Cal, CO Cal, Low Cal"(w1197) -> ()
            n493 = local write "FGGA Calibration Abort"(w1197) -> ()
            n494 = local write "Low Cal"(w1197) -> ()
            n495 = Bundle(cluster=T4 {"Message"="", "Message Data"=variant} ("Message Cluster"), "Message"="MFC_1", "Message Data"=w1199) -> (w1203:T4)
            n496 = Enqueue Element(queue=w1201, element=w1203, error in (no error)=w1200) -> (error out=w1198:errorcluster)  [unwired: 1 in, 2 out]
          }
        }
      }
      event "Flush High Tank": Value Change {
        n497 = event-data() -> ()  [unwired: 1 in, 6 out]
        n498 = flat-sequence {
          tunnel: w1216 -> [w1221]
          tunnel: w1215 -> [w1220]
          tunnel: [w1219] -> w1214
          tunnel: [w1218] -> w1213
          tunnel: w1214 -> [w1237]
          tunnel: w1213 -> [w1236]
          tunnel: [w1234] -> w1212
          tunnel: [w1233] -> w1211
          tunnel: w1212 -> [w1240]
          tunnel: w1211 -> [w1241]
          tunnel: [w1241] -> w1206
          tunnel: [w1240] -> w1205
          tunnel: [w1254] -> w1210
          tunnel: [w1253] -> w1209
          tunnel: w1206 -> [w1252]
          tunnel: w1205 -> [w1251]
          tunnel: w1210 -> [w1269]
          tunnel: w1209 -> [w1268]
          tunnel: [w1266] -> w1207
          tunnel: [w1274] -> w1208
          tunnel: w1207 -> [w1274]
          frame #0 {
            w1217 = TRUE
            n499 = Cluster To Array(cluster=T11 {"Message"="V2", "Message 2"="V3", "Message 3"="V4"}) -> (array=w1222:string[])
            n500 = for {
              tunnel: w1222 -> [w1229] mode=indexing
              tunnel: w1221 -> [w1228]
              tunnel: w1220 -> [w1227]
              tunnel: [w1226] -> w1219
              tunnel: [w1225] -> w1218
              tunnel: w1217 -> [w1224]
              n501 = Bundle(cluster=T4 {"Message"="", "Message Data"=variant} ("Message Cluster"), "Message"=w1229, "Message Data"=w1224) -> (w1231:T4)
              n502 = Enqueue Element(queue=w1228, element=w1231, error in (no error)=w1227) -> (queue out=w1226:refnum<queue>, error out=w1225:errorcluster)  [unwired: 1 in, 1 out]
            }
            n503 = local write "eV2"(w1217) -> ()
            n504 = local write "eV4"(w1217) -> ()
            n505 = local write "eV3"(w1217) -> ()
          }
          frame #1 {
            n506 = local read "MFC_1 User Set Value"() -> (w1232:dbl)
            n507 = local write "MFC_1\nSLPM Value"(w1232) -> ()
            n508 = Bundle(cluster=T4 {"Message"="", "Message Data"=variant} ("Message Cluster"), "Message"="MFC_1", "Message Data"=w1232) -> (w1235:T4)
            n509 = Enqueue Element(queue=w1237, element=w1235, error in (no error)=w1236) -> (queue out=w1234:refnum<queue>, error out=w1233:errorcluster)  [unwired: 1 in, 1 out]
          }
          frame #2 {
            n510 = for {
              N: 15 -> [w1249]
              i -> [w1248]
              stop <- w1244 stop-if-true
              n511 = Subtract(x=w1249, y=w1248) -> (x-y=w1247:i32)
              n512 = Decrement(x=w1247) -> (x-1=w1245:i32)
              n513 = local read "Network disconnected"() -> (w1244:bool)
              n514 = Wait (ms)(milliseconds to wait=u32 1000) -> ()  [unwired: 1 out]
              n515 = Select(t=0, s=w1244, f=w1245) -> (s? t:f=→"Flush High Tank\nTime Remain (sec)":i32)
            }
          }
          frame #3 {
            w1255 = FALSE
            n516 = Cluster To Array(cluster=T11 {"Message"="V2", "Message 2"="V3", "Message 3"="V4"}) -> (array=w1256:string[])
            n517 = for {
              tunnel: w1256 -> [w1263] mode=indexing
              tunnel: [w1262] -> w1254
              tunnel: [w1261] -> w1253
              tunnel: w1255 -> [w1260]
              tunnel: w1251 -> [w1259]
              tunnel: w1252 -> [w1258]
              n518 = Bundle(cluster=T4 {"Message"="", "Message Data"=variant} ("Message Cluster"), "Message"=w1263, "Message Data"=w1260) -> (w1265:T4)
              n519 = Enqueue Element(queue=w1259, element=w1265, error in (no error)=w1258) -> (queue out=w1262:refnum<queue>, error out=w1261:errorcluster)  [unwired: 1 in, 1 out]
            }
            n520 = local write "eV2"(w1255) -> ()
            n521 = local write "eV4"(w1255) -> ()
            n522 = local write "eV3"(w1255) -> ()
          }
          frame #4 {
            w1267 = 0.0 ("MFC_1\nSLPM Value")
            n523 = local write "MFC_1\nSLPM Value"(w1267) -> ()
            n524 = Bundle(cluster=T4 {"Message"="", "Message Data"=variant} ("Message Cluster"), "Message"="MFC_1", "Message Data"=w1267) -> (w1271:T4)
            n525 = Enqueue Element(queue=w1269, element=w1271, error in (no error)=w1268) -> (error out=w1266:errorcluster)  [unwired: 1 in, 2 out]
          }
          frame #5 {
            n526 = local write "Flush High Tank"(FALSE ("High Cal")) -> ()
          }
        }
      }
      event "Flush Low Tank": Value Change {
        n527 = event-data() -> ()  [unwired: 1 in, 1 out]
        n528 = flat-sequence {
          tunnel: w1286 -> [w1291]
          tunnel: w1285 -> [w1290]
          tunnel: [w1289] -> w1284
          tunnel: [w1288] -> w1283
          tunnel: w1284 -> [w1307]
          tunnel: w1283 -> [w1306]
          tunnel: [w1304] -> w1282
          tunnel: [w1303] -> w1281
          tunnel: w1282 -> [w1310]
          tunnel: w1281 -> [w1311]
          tunnel: [w1311] -> w1276
          tunnel: [w1310] -> w1275
          tunnel: [w1324] -> w1280
          tunnel: [w1323] -> w1279
          tunnel: w1276 -> [w1322]
          tunnel: w1275 -> [w1321]
          tunnel: w1280 -> [w1339]
          tunnel: w1279 -> [w1338]
          tunnel: [w1336] -> w1277
          tunnel: [w1344] -> w1278
          tunnel: w1277 -> [w1344]
          frame #0 {
            w1287 = TRUE
            n529 = Cluster To Array(cluster=cluster{"Message":string, "Message 3":string} {"Message"="V2", "Message 3"="V4"}) -> (array=w1292:string[])
            n530 = for {
              tunnel: w1292 -> [w1299] mode=indexing
              tunnel: w1291 -> [w1298]
              tunnel: w1290 -> [w1297]
              tunnel: [w1296] -> w1289
              tunnel: [w1295] -> w1288
              tunnel: w1287 -> [w1294]
              n531 = Bundle(cluster=T4 {"Message"="", "Message Data"=variant} ("Message Cluster"), "Message"=w1299, "Message Data"=w1294) -> (w1301:T4)
              n532 = Enqueue Element(queue=w1298, element=w1301, error in (no error)=w1297) -> (queue out=w1296:refnum<queue>, error out=w1295:errorcluster)  [unwired: 1 in, 1 out]
            }
            n533 = local write "eV2"(w1287) -> ()
            n534 = local write "eV4"(w1287) -> ()
          }
          frame #1 {
            n535 = local read "MFC_1 User Set Value"() -> (w1302:dbl)
            n536 = local write "MFC_1\nSLPM Value"(w1302) -> ()
            n537 = Bundle(cluster=T4 {"Message"="", "Message Data"=variant} ("Message Cluster"), "Message"="MFC_1", "Message Data"=w1302) -> (w1305:T4)
            n538 = Enqueue Element(queue=w1307, element=w1305, error in (no error)=w1306) -> (queue out=w1304:refnum<queue>, error out=w1303:errorcluster)  [unwired: 1 in, 1 out]
          }
          frame #2 {
            n539 = for {
              N: 15 -> [w1319]
              i -> [w1318]
              stop <- w1313 stop-if-true
              n540 = Subtract(x=w1319, y=w1318) -> (x-y=w1317:i32)
              n541 = Decrement(x=w1317) -> (x-1=w1314:i32)
              n542 = local read "Network disconnected"() -> (w1313:bool)
              n543 = Wait (ms)(milliseconds to wait=u32 1000) -> ()  [unwired: 1 out]
              n544 = Select(t=0, s=w1313, f=w1314) -> (s? t:f=→"Flush Low Tank\nTime Remain (sec)":i32)
            }
          }
          frame #3 {
            w1325 = FALSE
            n545 = Cluster To Array(cluster=cluster{"Message":string, "Message 3":string} {"Message"="V2", "Message 3"="V4"}) -> (array=w1326:string[])
            n546 = for {
              tunnel: w1326 -> [w1333] mode=indexing
              tunnel: [w1332] -> w1324
              tunnel: [w1331] -> w1323
              tunnel: w1325 -> [w1330]
              tunnel: w1321 -> [w1329]
              tunnel: w1322 -> [w1328]
              n547 = Bundle(cluster=T4 {"Message"="", "Message Data"=variant} ("Message Cluster"), "Message"=w1333, "Message Data"=w1330) -> (w1335:T4)
              n548 = Enqueue Element(queue=w1329, element=w1335, error in (no error)=w1328) -> (queue out=w1332:refnum<queue>, error out=w1331:errorcluster)  [unwired: 1 in, 1 out]
            }
            n549 = local write "eV2"(w1325) -> ()
            n550 = local write "eV4"(w1325) -> ()
          }
          frame #4 {
            w1337 = 0.0 ("MFC_1\nSLPM Value")
            n551 = local write "MFC_1\nSLPM Value"(w1337) -> ()
            n552 = Bundle(cluster=T4 {"Message"="", "Message Data"=variant} ("Message Cluster"), "Message"="MFC_1", "Message Data"=w1337) -> (w1341:T4)
            n553 = Enqueue Element(queue=w1339, element=w1341, error in (no error)=w1338) -> (error out=w1336:errorcluster)  [unwired: 1 in, 2 out]
          }
          frame #5 {
            n554 = local write "Flush Low Tank"(FALSE ("High Cal")) -> ()
          }
        }
      }
      event "Flush Target Tank": Value Change {
        n555 = event-data() -> ()  [unwired: 1 in, 1 out]
        n556 = flat-sequence {
          tunnel: w1356 -> [w1364]
          tunnel: w1355 -> [w1363]
          tunnel: [w1362] -> w1354
          tunnel: [w1361] -> w1353
          tunnel: w1354 -> [w1370]
          tunnel: w1353 -> [w1369]
          tunnel: [w1367] -> w1352
          tunnel: [w1366] -> w1351
          tunnel: w1352 -> [w1373]
          tunnel: w1351 -> [w1374]
          tunnel: [w1374] -> w1346
          tunnel: [w1373] -> w1345
          tunnel: [w1390] -> w1350
          tunnel: [w1389] -> w1349
          tunnel: w1346 -> [w1388]
          tunnel: w1345 -> [w1387]
          tunnel: w1350 -> [w1395]
          tunnel: w1349 -> [w1394]
          tunnel: [w1392] -> w1347
          tunnel: [w1400] -> w1348
          tunnel: w1347 -> [w1400]
          frame #0 {
            w1360 = TRUE
            n557 = local write "eV4"(w1360) -> ()
            n558 = Bundle(cluster=T4 {"Message"="", "Message Data"=variant} ("Message Cluster"), "Message"="V4" ("Message 3"), "Message Data"=w1360) -> (w1359:T4)
            n559 = Enqueue Element(queue=w1364, element=w1359, error in (no error)=w1363) -> (queue out=w1362:refnum<queue>, error out=w1361:errorcluster)  [unwired: 1 in, 1 out]
          }
          frame #1 {
            n560 = local read "MFC_1 User Set Value"() -> (w1365:dbl)
            n561 = local write "MFC_1\nSLPM Value"(w1365) -> ()
            n562 = Bundle(cluster=T4 {"Message"="", "Message Data"=variant} ("Message Cluster"), "Message"="MFC_1", "Message Data"=w1365) -> (w1368:T4)
            n563 = Enqueue Element(queue=w1370, element=w1368, error in (no error)=w1369) -> (queue out=w1367:refnum<queue>, error out=w1366:errorcluster)  [unwired: 1 in, 1 out]
          }
          frame #2 {
            n564 = for {
              N: 15 -> [w1382]
              i -> [w1381]
              stop <- w1377 stop-if-true
              n565 = Subtract(x=w1382, y=w1381) -> (x-y=w1380:i32)
              n566 = Decrement(x=w1380) -> (x-1=w1378:i32)
              n567 = Wait (ms)(milliseconds to wait=u32 1000) -> ()  [unwired: 1 out]
              n568 = local read "Network disconnected"() -> (w1377:bool)
              n569 = Select(t=0, s=w1377, f=w1378) -> (s? t:f=→"Flush Target Tank\nTime Remain (sec)":i32)
            }
          }
          frame #3 {
            w1391 = FALSE
            n570 = Bundle(cluster=T4 {"Message"="", "Message Data"=variant} ("Message Cluster"), "Message"="V4" ("Message 3"), "Message Data"=w1391) -> (w1386:T4)
            n571 = local write "eV4"(w1391) -> ()
            n572 = Enqueue Element(queue=w1387, element=w1386, error in (no error)=w1388) -> (queue out=w1390:refnum<queue>, error out=w1389:errorcluster)  [unwired: 1 in, 1 out]
          }
          frame #4 {
            w1393 = 0.0 ("MFC_1\nSLPM Value")
            n573 = local write "MFC_1\nSLPM Value"(w1393) -> ()
            n574 = Bundle(cluster=T4 {"Message"="", "Message Data"=variant} ("Message Cluster"), "Message"="MFC_1", "Message Data"=w1393) -> (w1397:T4)
            n575 = Enqueue Element(queue=w1395, element=w1397, error in (no error)=w1394) -> (error out=w1392:errorcluster)  [unwired: 1 in, 2 out]
          }
          frame #5 {
            n576 = local write "Flush Target Tank"(FALSE ("High Cal")) -> ()
          }
        }
      }
      event "Low Cal": Value Change {
        n577 = event-data() -> ()  [unwired: 1 in, 1 out]
        n578 = flat-sequence {
          tunnel: w1412 -> [w1417]
          tunnel: w1411 -> [w1416]
          tunnel: [w1415] -> w1410
          tunnel: [w1414] -> w1409
          tunnel: w1410 -> [w1433]
          tunnel: w1409 -> [w1432]
          tunnel: [w1430] -> w1408
          tunnel: [w1429] -> w1407
          tunnel: [w1438] -> w1406
          tunnel: [w1437] -> w1405
          tunnel: w1407 -> [w1441]
          tunnel: w1408 -> [w1442]
          tunnel: w1406 -> [w1495]
          tunnel: w1405 -> [w1494]
          tunnel: [w1492] -> w1404
          tunnel: [w1491] -> w1403
          tunnel: w1404 -> [w1509]
          tunnel: w1403 -> [w1508]
          tunnel: [w1506] -> w1401
          tunnel: [w1514] -> w1402
          tunnel: w1401 -> [w1514]
          frame #0 {
            w1413 = TRUE
            n579 = Cluster To Array(cluster=cluster{"Message":string, "Message 3":string} {"Message"="V2", "Message 3"="V4"}) -> (array=w1418:string[])
            n580 = for {
              tunnel: w1418 -> [w1425] mode=indexing
              tunnel: w1417 -> [w1424]
              tunnel: w1416 -> [w1423]
              tunnel: [w1422] -> w1415
              tunnel: [w1421] -> w1414
              tunnel: w1413 -> [w1420]
              n581 = Bundle(cluster=T4 {"Message"="", "Message Data"=variant} ("Message Cluster"), "Message"=w1425, "Message Data"=w1420) -> (w1427:T4)
              n582 = Enqueue Element(queue=w1424, element=w1427, error in (no error)=w1423) -> (queue out=w1422:refnum<queue>, error out=w1421:errorcluster)  [unwired: 1 in, 1 out]
            }
            n583 = local write "eV2"(w1413) -> ()
            n584 = local write "eV4"(w1413) -> ()
          }
          frame #1 {
            n585 = local read "MFC_1 User Set Value"() -> (w1428:dbl)
            n586 = local write "MFC_1\nSLPM Value"(w1428) -> ()
            n587 = Bundle(cluster=T4 {"Message"="", "Message Data"=variant} ("Message Cluster"), "Message"="MFC_1", "Message Data"=w1428) -> (w1431:T4)
            n588 = Enqueue Element(queue=w1433, element=w1431, error in (no error)=w1432) -> (queue out=w1430:refnum<queue>, error out=w1429:errorcluster)  [unwired: 1 in, 1 out]
          }
          frame #2 {
            n589 = for {
              N: 45 -> [w1485]
              tunnel: w1442 -> [w1476]
              tunnel: w1441 -> [w1475]
              tunnel: [w1476] -> w1440
              tunnel: [w1475] -> w1439
              tunnel: [w1474] -> w1436
              i -> [w1484]
              stop <- w1474 stop-if-true
              n590 = local read "FGGA Calibration Abort"() -> (w1479:bool)
              n591 = case shown="True" w1479 {
                selector: w1479 -> [w1488 _]
                tunnel: [w1488 w1489] -> w1477
                frame False {
                }
                frame True {
                  n592 = Two Button Dialog(message="Are you sure to abort FGGA Low Cal?") -> (T button?=w1489:bool)  [unwired: 2 in]
                }
              }
              n593 = local read "Network disconnected"() -> (w1478:bool)
              n594 = Subtract(x=w1485, y=w1484) -> (x-y=w1483:i32)
              n595 = Decrement(x=w1483) -> (x-1=w1481:i32)
              n596 = Wait (ms)(milliseconds to wait=u32 1000) -> ()  [unwired: 1 out]
              n597 = Or(x=w1478, y=w1477) -> (x .or. y?=w1474:bool)
              n598 = case shown="False" w1477 {
                selector: w1477 -> [w1487 _]
                frame False {
                  n599 = local write "FGGA Calibration Abort"(w1487) -> ()
                }
                frame True {
                }
              }
              n600 = Select(t=0, s=w1474, f=w1481) -> (s? t:f=→"Low Cal\nFlush Time Remain (sec)":i32)
            }
            n601 = case shown="False" w1436 {
              tunnel: w1440 -> [w1449 w1473]
              tunnel: w1439 -> [w1448 w1472]
              tunnel: [w1446 w1473] -> w1438
              tunnel: [w1444 w1472] -> w1437
              frame False {
                w1450 = TRUE
                # "Carry on if connection to cRIO is made\nor calibration not abort"
                n602 = Bundle(cluster=T4 {"Message"="", "Message Data"=variant} ("Message Cluster"), "Message"="V1", "Message Data"=w1450) -> (w1451:T4)
                n603 = local write "eV1"(w1450) -> ()
                n604 = Enqueue Element(queue=w1449, element=w1451, error in (no error)=w1448) -> (queue out=w1447:refnum<queue>, error out=w1445:errorcluster)  [unwired: 1 in, 1 out]
                n605 = for {
                  N: 60 -> [w1466]
                  tunnel: w1447 -> [w1456]
                  tunnel: [w1456] -> w1446
                  tunnel: w1445 -> [w1455]
                  tunnel: [w1455] -> w1444
                  i -> [w1465]
                  stop <- w1457 stop-if-true
                  n606 = Subtract(x=w1466, y=w1465) -> (x-y=w1464:i32)
                  n607 = local read "FGGA Calibration Abort"() -> (w1459:bool)
                  n608 = case shown="True" w1459 {
                    selector: w1459 -> [w1469 _]
                    tunnel: [w1469 w1470] -> w1458
                    frame False {
                    }
                    frame True {
                      n609 = Two Button Dialog(message="Are you sure to abort FGGA Low Cal?") -> (T button?=w1470:bool)  [unwired: 2 in]
                    }
                  }
                  n610 = Decrement(x=w1464) -> (x-1=w1461:i32)
                  n611 = local read "Network disconnected"() -> (w1460:bool)
                  n612 = Wait (ms)(milliseconds to wait=u32 1000) -> ()  [unwired: 1 out]
                  n613 = Or(x=w1460, y=w1458) -> (x .or. y?=w1457:bool)
                  n614 = case shown="False" w1458 {
                    selector: w1458 -> [w1468 _]
                    frame False {
                      n615 = local write "FGGA Calibration Abort"(w1468) -> ()
                    }
                    frame True {
                    }
                  }
                  n616 = Select(t=0, s=w1457, f=w1461) -> (s? t:f=→"Low Cal\nCal Time Remain (sec)":i32)
                }
              }
              frame True {
              }
            }
          }
          frame #3 {
            w1493 = FALSE
            n617 = Cluster To Array(cluster=T13 {"Message"="V2", "Message 3"="V4", "Message 4"="V1"}) -> (array=w1496:string[])
            n618 = for {
              tunnel: w1496 -> [w1503] mode=indexing
              tunnel: [w1502] -> w1492
              tunnel: [w1501] -> w1491
              tunnel: w1493 -> [w1500]
              tunnel: w1495 -> [w1499]
              tunnel: w1494 -> [w1498]
              n619 = Bundle(cluster=T4 {"Message"="", "Message Data"=variant} ("Message Cluster"), "Message"=w1503, "Message Data"=w1500) -> (w1505:T4)
              n620 = Enqueue Element(queue=w1499, element=w1505, error in (no error)=w1498) -> (queue out=w1502:refnum<queue>, error out=w1501:errorcluster)  [unwired: 1 in, 1 out]
            }
            n621 = local write "eV2"(w1493) -> ()
            n622 = local write "eV4"(w1493) -> ()
            n623 = local write "eV1"(w1493) -> ()
          }
          frame #4 {
            w1507 = 0.0 ("MFC_1\nSLPM Value")
            n624 = local write "MFC_1\nSLPM Value"(w1507) -> ()
            n625 = Bundle(cluster=T4 {"Message"="", "Message Data"=variant} ("Message Cluster"), "Message"="MFC_1", "Message Data"=w1507) -> (w1511:T4)
            n626 = Enqueue Element(queue=w1509, element=w1511, error in (no error)=w1508) -> (error out=w1506:errorcluster)  [unwired: 1 in, 2 out]
          }
          frame #5 {
            w1513 = FALSE ("High Cal")
            n627 = local write "Low Cal"(w1513) -> ()
            n628 = local write "FGGA Calibration Abort"(w1513) -> ()
          }
        }
      }
      event "Target Cal": Value Change {
        n629 = event-data() -> ()  [unwired: 1 in, 1 out]
        n630 = flat-sequence {
          tunnel: w1526 -> [w1534]
          tunnel: w1525 -> [w1533]
          tunnel: [w1532] -> w1524
          tunnel: [w1531] -> w1523
          tunnel: w1524 -> [w1540]
          tunnel: w1523 -> [w1539]
          tunnel: [w1537] -> w1522
          tunnel: [w1536] -> w1521
          tunnel: w1521 -> [w1547]
          tunnel: w1522 -> [w1548]
          tunnel: [w1545] -> w1516
          tunnel: [w1544] -> w1515
          tunnel: [w1600] -> w1520
          tunnel: [w1601] -> w1519
          tunnel: w1516 -> [w1599]
          tunnel: w1515 -> [w1598]
          tunnel: w1520 -> [w1616]
          tunnel: w1519 -> [w1615]
          tunnel: [w1613] -> w1517
          tunnel: [w1621] -> w1518
          tunnel: w1517 -> [w1621]
          frame #0 {
            w1530 = TRUE
            n631 = local write "eV4"(w1530) -> ()
            n632 = Bundle(cluster=T4 {"Message"="", "Message Data"=variant} ("Message Cluster"), "Message"="V4" ("Message 3"), "Message Data"=w1530) -> (w1529:T4)
            n633 = Enqueue Element(queue=w1534, element=w1529, error in (no error)=w1533) -> (queue out=w1532:refnum<queue>, error out=w1531:errorcluster)  [unwired: 1 in, 1 out]
          }
          frame #1 {
            n634 = local read "MFC_1 User Set Value"() -> (w1535:dbl)
            n635 = local write "MFC_1\nSLPM Value"(w1535) -> ()
            n636 = Bundle(cluster=T4 {"Message"="", "Message Data"=variant} ("Message Cluster"), "Message"="MFC_1", "Message Data"=w1535) -> (w1538:T4)
            n637 = Enqueue Element(queue=w1540, element=w1538, error in (no error)=w1539) -> (queue out=w1537:refnum<queue>, error out=w1536:errorcluster)  [unwired: 1 in, 1 out]
          }
          frame #2 {
            n638 = for {
              N: 45 -> [w1592]
              tunnel: [w1583] -> w1549
              tunnel: w1548 -> [w1583]
              tunnel: [w1582] -> w1546
              tunnel: w1547 -> [w1582]
              tunnel: [w1581] -> w1543
              i -> [w1591]
              stop <- w1581 stop-if-true
              n639 = Subtract(x=w1592, y=w1591) -> (x-y=w1590:i32)
              n640 = Decrement(x=w1590) -> (x-1=w1587:i32)
              n641 = local read "FGGA Calibration Abort"() -> (w1586:bool)
              n642 = local read "Network disconnected"() -> (w1585:bool)
              n643 = case shown="True" w1586 {
                selector: w1586 -> [w1595 _]
                tunnel: [w1595 w1596] -> w1584
                frame False {
                }
                frame True {
                  n644 = Two Button Dialog(message="Are you sure to abort FGGA Target Cal?") -> (T button?=w1596:bool)  [unwired: 2 in]
                }
              }
              n645 = Wait (ms)(milliseconds to wait=u32 1000) -> ()  [unwired: 1 out]
              n646 = Or(x=w1585, y=w1584) -> (x .or. y?=w1581:bool)
              n647 = case shown="False" w1584 {
                selector: w1584 -> [w1594 _]
                frame False {
                  n648 = local write "FGGA Calibration Abort"(w1594) -> ()
                }
                frame True {
                }
              }
              n649 = Select(t=0, s=w1581, f=w1587) -> (s? t:f=→"Target Cal\nFlush Time Remain (sec)":i32)
            }
            n650 = case shown="False" w1543 {
              tunnel: w1549 -> [w1556 w1580]
              tunnel: w1546 -> [w1555 w1579]
              tunnel: [w1552 w1580] -> w1545
              tunnel: [w1551 w1579] -> w1544
              frame False {
                w1557 = TRUE
                # "Carry on if connection to cRIO is made\nor calibration not abort"
                n651 = Bundle(cluster=T4 {"Message"="", "Message Data"=variant} ("Message Cluster"), "Message"="V1", "Message Data"=w1557) -> (w1558:T4)
                n652 = local write "eV1"(w1557) -> ()
                n653 = Enqueue Element(queue=w1556, element=w1558, error in (no error)=w1555) -> (queue out=w1554:refnum<queue>, error out=w1553:errorcluster)  [unwired: 1 in, 1 out]
                n654 = for {
                  N: 60 -> [w1573]
                  tunnel: w1554 -> [w1563]
                  tunnel: w1553 -> [w1562]
                  tunnel: [w1563] -> w1552
                  tunnel: [w1562] -> w1551
                  i -> [w1572]
                  stop <- w1564 stop-if-true
                  n655 = Subtract(x=w1573, y=w1572) -> (x-y=w1571:i32)
                  n656 = Decrement(x=w1571) -> (x-1=w1569:i32)
                  n657 = local read "FGGA Calibration Abort"() -> (w1567:bool)
                  n658 = case shown="True" w1567 {
                    selector: w1567 -> [w1576 _]
                    tunnel: [w1576 w1577] -> w1565
                    frame False {
                    }
                    frame True {
                      n659 = Two Button Dialog(message="Are you sure to abort FGGA Target Cal?") -> (T button?=w1577:bool)  [unwired: 2 in]
                    }
                  }
                  n660 = Wait (ms)(milliseconds to wait=u32 1000) -> ()  [unwired: 1 out]
                  n661 = local read "Network disconnected"() -> (w1566:bool)
                  n662 = Or(x=w1566, y=w1565) -> (x .or. y?=w1564:bool)
                  n663 = case shown="False" w1565 {
                    selector: w1565 -> [w1575 _]
                    frame False {
                      n664 = local write "FGGA Calibration Abort"(w1575) -> ()
                    }
                    frame True {
                    }
                  }
                  n665 = Select(t=0, s=w1564, f=w1569) -> (s? t:f=→"Target Cal\nCal Time Remain (sec)":i32)
                }
              }
              frame True {
              }
            }
          }
          frame #3 {
            w1604 = FALSE
            n666 = Cluster To Array(cluster=cluster{"Message 3":string, "Message":string} {"Message 3"="V4", "Message"="V1"}) -> (array=w1602:string[])
            n667 = for {
              tunnel: w1602 -> [w1610] mode=indexing
              tunnel: [w1609] -> w1600
              tunnel: [w1608] -> w1601
              tunnel: w1604 -> [w1607]
              tunnel: w1599 -> [w1606]
              tunnel: w1598 -> [w1605]
              n668 = Bundle(cluster=T4 {"Message"="", "Message Data"=variant} ("Message Cluster"), "Message"=w1610, "Message Data"=w1607) -> (w1612:T4)
              n669 = Enqueue Element(queue=w1606, element=w1612, error in (no error)=w1605) -> (queue out=w1609:refnum<queue>, error out=w1608:errorcluster)  [unwired: 1 in, 1 out]
            }
            n670 = local write "eV4"(w1604) -> ()
            n671 = local write "eV1"(w1604) -> ()
          }
          frame #4 {
            w1614 = 0.0 ("MFC_1\nSLPM Value")
            n672 = local write "MFC_1\nSLPM Value"(w1614) -> ()
            n673 = Bundle(cluster=T4 {"Message"="", "Message Data"=variant} ("Message Cluster"), "Message"="MFC_1", "Message Data"=w1614) -> (w1618:T4)
            n674 = Enqueue Element(queue=w1616, element=w1618, error in (no error)=w1615) -> (error out=w1613:errorcluster)  [unwired: 1 in, 2 out]
          }
          frame #5 {
            w1620 = FALSE ("High Cal")
            n675 = local write "Target Cal"(w1620) -> ()
            n676 = local write "FGGA Calibration Abort"(w1620) -> ()
          }
        }
      }
      event "MFC_1\nSLPM Value": Value Change {
        n677 = event-data() -> ()  [unwired: 1 in, 1 out]
        n678 = local read "MFC_1\nSLPM Value"() -> (w1622:dbl)
        n679 = Bundle(cluster=T4 {"Message"="", "Message Data"=variant} ("Message Cluster"), "Message"="MFC_1", "Message Data"=w1622) -> (w1626:T4)
        n680 = Enqueue Element(queue=w1625, element=w1626, error in (no error)=w1624) -> (error out=w1623:errorcluster)  [unwired: 1 in, 2 out]
      }
      event "FGGA UDP Time Offset": Value Change {
        n681 = event-data() -> ("NewVal"=w1629:i32)  [unwired: 1 in, 5 out]
        n682 = Bundle(cluster=T4 {"Message"="", "Message Data"=variant} ("Message Cluster"), "Message"="UDP Time Offset", "Message Data"=w1629) -> (w1633:T4)
        n683 = Enqueue Element(queue=w1632, element=w1633, error in (no error)=w1631) -> (error out=w1630:errorcluster)  [unwired: 1 in, 2 out]
      }
    }
    "FGGA Event Error out" <- w747
  }
  n684 = node-c288(w14) -> ()  [unwired: 1 out]
  n685 = Create Network Stream Writer Endpoint(6:w54, 7:10 ("writer buffer size"), 9:w56, 10:"//192.168.101.17/command/reader/FGGA" ("reader url"), 11:"/command/writer/FGGA" ("writer name")) -> (0:w53:errorcluster, 3:w52:refnum<k21>)  [unwired: 2 in]
  n686 = while {
    tunnel: w6 -> [w1643]
    shift-right: [w1638] -> _
    shift-left: w52 -> [w1640]
    shift-right: [w1636] -> w49
    shift-left: w53 -> [w1642]
    tunnel: w5 -> [w1637]
    stop <- w1636 stop-if-true
    # "FGGA UI Command Sender"
    n687 = Dequeue Element(queue=w1643, error in (no error)=w1637) -> (element=w1639:T4)  [unwired: 1 in, 3 out]
    n688 = Unbundle By Name(w1639) -> ("Message"=w1641:string)
    n689 = case shown="\"UDP Time Offset\"" w1641 {
      tunnel: w1642 -> [w1644 w1648 w1655 w1662 w1669 w1676 w1683 w1690 w1697 w1704 w1711]
      tunnel: w1640 -> [w1645 w1651 w1658 w1665 w1672 w1679 w1686 w1693 w1700 w1707 w1714]
      tunnel: w1639 -> [_ w1650 w1657 w1664 w1671 w1678 w1685 w1692 w1699 w1706 w1713]
      tunnel: [w1644 w1647 w1654 w1661 w1668 w1675 w1682 w1689 w1696 w1703 w1710] -> w1636
      tunnel: [w1645 w1646 w1653 w1660 w1667 w1674 w1681 w1688 w1695 w1702 w1709] -> w1638
      frame "False", Default {
      }
      frame "V1" {
        n690 = shared-variable-write(w1651, w1648, w1650) -> (w1649:refnum<k21>, w1652:errorcluster)  [unwired: 1 in, 1 out]
        n691 = Flush Stream(8:w1652, 11:w1649) -> (0:w1647:errorcluster, 3:w1646:refnum<k21>)  [unwired: 2 in, 1 out]
      }
      frame "MFC_1" {
        n692 = shared-variable-write(w1658, w1655, w1657) -> (w1656:refnum<k21>, w1659:errorcluster)  [unwired: 1 in, 1 out]
        n693 = Flush Stream(8:w1659, 11:w1656) -> (0:w1654:errorcluster, 3:w1653:refnum<k21>)  [unwired: 2 in, 1 out]
      }
      frame "UDP Time Offset" {
        n694 = shared-variable-write(w1665, w1662, w1664) -> (w1663:refnum<k21>, w1666:errorcluster)  [unwired: 1 in, 1 out]
        n695 = Flush Stream(8:w1666, 11:w1663) -> (0:w1661:errorcluster, 3:w1660:refnum<k21>)  [unwired: 2 in, 1 out]
      }
      frame "V2" {
        n696 = shared-variable-write(w1672, w1669, w1671) -> (w1670:refnum<k21>, w1673:errorcluster)  [unwired: 1 in, 1 out]
        n697 = Flush Stream(8:w1673, 11:w1670) -> (0:w1668:errorcluster, 3:w1667:refnum<k21>)  [unwired: 2 in, 1 out]
      }
      frame "V3" {
        n698 = shared-variable-write(w1679, w1676, w1678) -> (w1677:refnum<k21>, w1680:errorcluster)  [unwired: 1 in, 1 out]
        n699 = Flush Stream(8:w1680, 11:w1677) -> (0:w1675:errorcluster, 3:w1674:refnum<k21>)  [unwired: 2 in, 1 out]
      }
      frame "V4" {
        n700 = shared-variable-write(w1686, w1683, w1685) -> (w1684:refnum<k21>, w1687:errorcluster)  [unwired: 1 in, 1 out]
        n701 = Flush Stream(8:w1687, 11:w1684) -> (0:w1682:errorcluster, 3:w1681:refnum<k21>)  [unwired: 2 in, 1 out]
      }
      frame "FGGA_pump" {
        n702 = shared-variable-write(w1693, w1690, w1692) -> (w1691:refnum<k21>, w1694:errorcluster)  [unwired: 1 in, 1 out]
        n703 = Flush Stream(8:w1694, 11:w1691) -> (0:w1689:errorcluster, 3:w1688:refnum<k21>)  [unwired: 2 in, 1 out]
      }
      frame "Flight Number" {
        n704 = shared-variable-write(w1700, w1697, w1699) -> (w1698:refnum<k21>, w1701:errorcluster)  [unwired: 1 in, 1 out]
        n705 = Flush Stream(8:w1701, 11:w1698) -> (0:w1696:errorcluster, 3:w1695:refnum<k21>)  [unwired: 2 in, 1 out]
      }
      frame "FGGA_restart" {
        n706 = shared-variable-write(w1707, w1704, w1706) -> (w1705:refnum<k21>, w1708:errorcluster)  [unwired: 1 in, 1 out]
        n707 = Flush Stream(8:w1708, 11:w1705) -> (0:w1703:errorcluster, 3:w1702:refnum<k21>)  [unwired: 2 in, 1 out]
      }
      frame "Stop File Write" {
        n708 = shared-variable-write(w1714, w1711, w1713) -> (w1712:refnum<k21>, w1715:errorcluster)  [unwired: 1 in, 1 out]
        n709 = Flush Stream(8:w1715, 11:w1712) -> (0:w1710:errorcluster, 3:w1709:refnum<k21>)  [unwired: 2 in, 1 out]
      }
    }
  }
  "FGGA command sender error out" <- w49
  n710 = local write "FGGA Calibration Abort"(FALSE ("FGGA Calibration Abort")) -> ()
  n711 = Obtain Queue(name (unnamed)="SO2_Command", element data type=w40) -> (queue out=w4:refnum<queue>, error out=w3:errorcluster)  [unwired: 3 in, 1 out]
  n712 = while {
    tunnel: w4 -> [w1719]
    tunnel: w3 -> [w1718]
    tunnel: [w1716] -> _
    stop <- FALSE stop-if-true
    # "SO2 UI Event Handler Loop"
    n713 = event shown="[7] \"SO2 Zero Calibration\": Value Change" {
      selector: _ -> [_ _ _ _ _ _ _ _ _ _ _ _ _ _ _ _ _ _ _ _ _ _ _ _ _ _ _ _ _ _]
      dyn-events: _ -> [_ _ _ _ _ _ _ _ _ _ _ _ _ _ _ _ _ _ _ _ _ _ _ _ _ _ _ _ _ _]
      timeout: _ -> [_ _ _ _ _ _ _ _ _ _ _ _ _ _ _ _ _ _ _ _ _ _ _ _ _ _ _ _ _ _]
      tunnel: w1719 -> [w1726 w1738 w1785 w1796 w1839 w1874 w1985 w2133 w2259 w2265 w2276 w2279 w2287 w2293 w2300 w2306 w2312 w2322 w2326 w2333 w2340 w2347 w2354 w2361 w2368 w2375 w2382 w2389 w2397 w2411]
      tunnel: w1718 -> [w1725 w1737 w1784 w1795 w1838 w1873 w1984 w2132 w2258 w2264 w2275 w2278 w2285 w2292 w2299 w2305 w2311 w2321 w2325 w2332 w2339 w2346 w2353 w2360 w2367 w2374 w2381 w2388 w2396 w2410]
      tunnel: [w1720 w1736 _ w1794 w1837 _ _ _ _ _ w2270 w2277 w2284 _ w2298 _ _ w2316 w2324 w2331 w2338 w2345 w2352 w2359 w2366 w2373 w2380 w2387 w2395 w2409] -> w1716
      event "eV9": Value Change {
        n714 = event-data() -> ("NewVal"=w1723:bool)  [unwired: 1 in]
        n715 = Bundle(cluster=T4 {"Message"="", "Message Data"=variant} ("Message Cluster"), "Message"="V9", "Message Data"=w1723) -> (w1721:T4)
        n716 = Enqueue Element(queue=w1726, element=w1721, error in (no error)=w1725) -> (error out=w1720:errorcluster)  [unwired: 1 in, 2 out]
      }
      event "SO2 Flush": Value Change {
        n717 = event-data() -> ()  [unwired: 1 in, 1 out]
        n718 = flat-sequence {
          tunnel: w1738 -> [w1746]
          tunnel: w1737 -> [w1745]
          tunnel: [w1741] -> w1733
          tunnel: [w1739] -> w1731
          tunnel: w1733 -> [w1748]
          tunnel: [w1750] -> w1732
          tunnel: w1731 -> [w1749]
          tunnel: [w1751] -> w1730
          tunnel: w1732 -> [w1757]
          tunnel: [w1757] -> w1735
          tunnel: [w1755] -> w1734
          tunnel: w1730 -> [w1755]
          tunnel: w1735 -> [w1769]
          tunnel: [w1768] -> w1729
          tunnel: w1734 -> [w1770]
          tunnel: [w1766] -> w1727
          tunnel: w1729 -> [w1776]
          tunnel: [w1777] -> w1728
          tunnel: w1727 -> [w1775]
          tunnel: [w1782] -> w1736
          tunnel: w1728 -> [w1782]
          frame #0 {
            w1740 = TRUE ("SO2 Flush")
            n719 = Bundle(cluster=T4 {"Message"="", "Message Data"=variant} ("Message Cluster"), "Message"="V9", "Message Data"=w1740) -> (w1742:T4)
            n720 = local write "eV9"(w1740) -> ()
            n721 = Enqueue Element(queue=w1746, element=w1742, error in (no error)=w1745) -> (queue out=w1739:refnum<queue>, error out=w1741:errorcluster)  [unwired: 1 in, 1 out]
          }
          frame #1 {
            n722 = local read "MFC_2 User Set Value"() -> (w1747:dbl)
            n723 = local write "MFC_2\nSLPM Value"(w1747) -> ()
            n724 = Bundle(cluster=T4 {"Message"="", "Message Data"=variant} ("Message Cluster"), "Message"="MFC_2", "Message Data"=w1747) -> (w1752:T4)
            n725 = Enqueue Element(queue=w1749, element=w1752, error in (no error)=w1748) -> (queue out=w1751:refnum<queue>, error out=w1750:errorcluster)  [unwired: 1 in, 1 out]
          }
          frame #2 {
            n726 = for {
              N: "eV9 Flush User\nset time (sec)" -> [w1764]
              i -> [w1763]
              stop <- w1758 stop-if-true
              n727 = local read "Network disconnected"() -> (w1758:bool)
              n728 = Subtract(x=w1764, y=w1763) -> (x-y=w1762:i32)
              n729 = Decrement(x=w1762) -> (x-1=w1760:i32)
              n730 = Wait (ms)(milliseconds to wait=u32 1000) -> ()  [unwired: 1 out]
              n731 = Select(t=0, s=w1758, f=w1760) -> (s? t:f=w1759:i32)
              n732 = local write "SO2 Flush\nTime Remain (sec)"(w1759) -> ()
            }
          }
          frame #3 {
            w1767 = FALSE
            n733 = Bundle(cluster=T4 {"Message"="", "Message Data"=variant} ("Message Cluster"), "Message"="V9", "Message Data"=w1767) -> (w1771:T4)
            n734 = local write "eV9"(w1767) -> ()
            n735 = Enqueue Element(queue=w1770, element=w1771, error in (no error)=w1769) -> (queue out=w1766:refnum<queue>, error out=w1768:errorcluster)  [unwired: 1 in, 1 out]
          }
          frame #4 {
            w1774 = 0.0 ("MFC_2\nSLPM Value")
            n736 = local write "MFC_2\nSLPM Value"(w1774) -> ()
            n737 = Bundle(cluster=T4 {"Message"="", "Message Data"=variant} ("Message Cluster"), "Message"="MFC_2", "Message Data"=w1774) -> (w1778:T4)
            n738 = Enqueue Element(queue=w1775, element=w1778, error in (no error)=w1776) -> (error out=w1777:errorcluster)  [unwired: 1 in, 2 out]
          }
          frame #5 {
            n739 = local write "SO2 Flush"(FALSE ("SO2 Flush")) -> ()
          }
        }
      }
      event "Auto Zeroing \ninterval (sec)": Value Change {
        n740 = event-data() -> ("NewVal"=w1783:i32)  [unwired: 1 in]
        n741 = Bundle(cluster=T4 {"Message"="", "Message Data"=variant} ("Message Cluster"), "Message"="zeroing_interval", "Message Data"=w1783) -> (w1786:T4)
        n742 = Enqueue Element(queue=w1785, element=w1786, error in (no error)=w1784) -> ()  [unwired: 1 in, 3 out]
      }
      event "SO2 GND Zeroing": Value Change {
        n743 = event-data() -> ()  [unwired: 1 in, 1 out]
        n744 = flat-sequence {
          tunnel: w1796 -> [w1804]
          tunnel: w1795 -> [w1803]
          tunnel: [w1799] -> w1793
          tunnel: [w1797] -> w1789
          tunnel: w1793 -> [w1807]
          tunnel: [w1807] -> w1792
          tunnel: [w1806] -> w1790
          tunnel: w1789 -> [w1806]
          tunnel: w1792 -> [w1825]
          tunnel: [w1824] -> w1791
          tunnel: w1790 -> [w1826]
          tunnel: [w1831] -> w1794
          tunnel: w1791 -> [w1831]
          frame #0 {
            w1798 = TRUE ("SO2 Flush")
            n745 = local write "SO2 eV6"(w1798) -> ()
            n746 = Bundle(cluster=T4 {"Message"="", "Message Data"=variant} ("Message Cluster"), "Message"="V6", "Message Data"=w1798) -> (w1800:T4)
            n747 = Enqueue Element(queue=w1804, element=w1800, error in (no error)=w1803) -> (queue out=w1797:refnum<queue>, error out=w1799:errorcluster)  [unwired: 1 in, 1 out]
          }
          frame #1 {
            # "10 Mins Count down"
            n748 = for {
              N: "eV6 User\nset time (sec)" -> [w1817]
              i -> [w1816]
              stop <- w1808 stop-if-true
              n749 = local read "SO2 Calibration Abort"() -> (w1814:bool)
              n750 = case shown="True" w1814 {
                selector: w1814 -> [w1820 _]
                tunnel: [w1820 w1821] -> w1809
                frame False {
                }
                frame True {
                  n751 = Two Button Dialog(message="Are you sure to abort SO2 Zeroing?") -> (T button?=w1821:bool)  [unwired: 2 in]
                }
              }
              n752 = Subtract(x=w1817, y=w1816) -> (x-y=w1815:i32)
              n753 = Decrement(x=w1815) -> (x-1=w1811:i32)
              n754 = Wait (ms)(milliseconds to wait=u32 1000) -> ()  [unwired: 1 out]
              n755 = local read "Network disconnected"() -> (w1812:bool)
              n756 = Or(x=w1812, y=w1809) -> (x .or. y?=w1808:bool)
              n757 = case shown="False" w1809 {
                selector: w1809 -> [w1819 _]
                frame False {
                  n758 = local write "SO2 Calibration Abort"(w1819) -> ()
                }
                frame True {
                }
              }
              n759 = Select(t=0, s=w1808, f=w1811) -> (s? t:f=w1810:i32)
              n760 = local write "SO2 Zeroing\nTime Remain (sec)"(w1810) -> ()
            }
          }
          frame #2 {
            w1823 = FALSE
            n761 = Bundle(cluster=T4 {"Message"="", "Message Data"=variant} ("Message Cluster"), "Message"="V6", "Message Data"=w1823) -> (w1827:T4)
            n762 = local write "SO2 eV6"(w1823) -> ()
            n763 = Enqueue Element(queue=w1826, element=w1827, error in (no error)=w1825) -> (error out=w1824:errorcluster)  [unwired: 1 in, 2 out]
          }
          frame #3 {
            n764 = local write "SO2 GND Zeroing"(FALSE ("SO2 Flush")) -> ()
          }
        }
      }
      event "SO2 Inflight \nZeroing": Value Change {
        n765 = event-data() -> ()  [unwired: 1 in, 1 out]
        n766 = flat-sequence {
          tunnel: w1839 -> [w1847]
          tunnel: w1838 -> [w1846]
          tunnel: [w1842] -> w1836
          tunnel: [w1840] -> w1832
          tunnel: w1836 -> [w1850]
          tunnel: [w1850] -> w1835
          tunnel: [w1849] -> w1833
          tunnel: w1832 -> [w1849]
          tunnel: w1835 -> [w1858]
          tunnel: [w1857] -> w1834
          tunnel: w1833 -> [w1859]
          tunnel: [w1864] -> w1837
          tunnel: w1834 -> [w1864]
          frame #0 {
            w1841 = TRUE ("SO2 Flush")
            n767 = local write "SO2 eV6"(w1841) -> ()
            n768 = Bundle(cluster=T4 {"Message"="", "Message Data"=variant} ("Message Cluster"), "Message"="V6", "Message Data"=w1841) -> (w1843:T4)
            n769 = Enqueue Element(queue=w1847, element=w1843, error in (no error)=w1846) -> (queue out=w1840:refnum<queue>, error out=w1842:errorcluster)  [unwired: 1 in, 1 out]
          }
          frame #1 {
            n770 = for {
              N: "eV6 User set time \n(Inflight) (sec)" -> [w1854]
              i -> [w1853]
              n771 = Subtract(x=w1854, y=w1853) -> (x-y=w1852:i32)
              n772 = Decrement(x=w1852) -> (x-1=w1851:i32)
              n773 = local write "SO2 Zeroing (Inflight)\nTime Remain (sec)"(w1851) -> ()
              n774 = Wait (ms)(milliseconds to wait=u32 1000) -> ()  [unwired: 1 out]
            }
          }
          frame #2 {
            w1856 = FALSE
            n775 = Bundle(cluster=T4 {"Message"="", "Message Data"=variant} ("Message Cluster"), "Message"="V6", "Message Data"=w1856) -> (w1860:T4)
            n776 = local write "SO2 eV6"(w1856) -> ()
            n777 = Enqueue Element(queue=w1859, element=w1860, error in (no error)=w1858) -> (error out=w1857:errorcluster)  [unwired: 1 in, 2 out]
          }
          frame #3 {
            n778 = local write "SO2 Inflight \nZeroing"(FALSE ("SO2 Flush")) -> ()
          }
        }
      }
      event "SO2 Zero CAL": Value Change {
        n779 = event-data() -> ()  [unwired: 1 in, 1 out]
        n780 = flat-sequence {
          tunnel: [w1877] -> w1872
          tunnel: [w1876] -> w1870
          tunnel: w1874 -> [w1882]
          tunnel: w1873 -> [w1881]
          tunnel: w1872 -> [w1886]
          tunnel: [w1885] -> w1871
          tunnel: w1870 -> [w1887]
          tunnel: [w1883] -> w1869
          tunnel: [w1893] -> w1868
          tunnel: [w1892] -> w1867
          tunnel: w1869 -> [w1897]
          tunnel: w1871 -> [w1895]
          tunnel: w1868 -> [w1949]
          tunnel: w1867 -> [w1948]
          tunnel: [w1947] -> w1866
          tunnel: [w1946] -> w1865
          tunnel: w1866 -> [w1963]
          tunnel: w1865 -> [w1962]
          frame #0 {
            w1875 = TRUE ("SO2 Flush")
            n781 = Bundle(cluster=T4 {"Message"="", "Message Data"=variant} ("Message Cluster"), "Message"="V9", "Message Data"=w1875) -> (w1878:T4)
            n782 = local write "eV9"(w1875) -> ()
            n783 = Enqueue Element(queue=w1882, element=w1878, error in (no error)=w1881) -> (queue out=w1876:refnum<queue>, error out=w1877:errorcluster)  [unwired: 1 in, 1 out]
          }
          frame #1 {
            n784 = local read "MFC_2 User Set Value"() -> (w1884:dbl)
            n785 = local write "MFC_2\nSLPM Value"(w1884) -> ()
            n786 = Bundle(cluster=T4 {"Message"="", "Message Data"=variant} ("Message Cluster"), "Message"="MFC_2", "Message Data"=w1884) -> (w1888:T4)
            n787 = Enqueue Element(queue=w1887, element=w1888, error in (no error)=w1886) -> (queue out=w1883:refnum<queue>, error out=w1885:errorcluster)  [unwired: 1 in, 1 out]
          }
          frame #2 {
            n788 = for {
              N: "eV9 flush User\nset time (sec)" -> [w1940]
              tunnel: [w1931] -> w1896
              tunnel: w1897 -> [w1931]
              tunnel: [w1930] -> w1894
              tunnel: w1895 -> [w1930]
              tunnel: [w1929] -> w1891
              i -> [w1939]
              stop <- w1929 stop-if-true
              n789 = local read "SO2 Calibration Abort"() -> (w1936:bool)
              n790 = case shown="True" w1936 {
                selector: w1936 -> [w1943 _]
                tunnel: [w1943 w1944] -> w1934
                frame False {
                }
                frame True {
                  n791 = Two Button Dialog(message="Are you sure to abort SO2 Cal?") -> (T button?=w1944:bool)  [unwired: 2 in]
                }
              }
              n792 = Subtract(x=w1940, y=w1939) -> (x-y=w1938:i32)
              n793 = Decrement(x=w1938) -> (x-1=w1932:i32)
              n794 = Wait (ms)(milliseconds to wait=u32 1000) -> ()  [unwired: 1 out]
              n795 = local read "Network disconnected"() -> (w1935:bool)
              n796 = Or(x=w1935, y=w1934) -> (x .or. y?=w1929:bool)
              n797 = Select(t=0, s=w1929, f=w1932) -> (s? t:f=w1933:i32)
              n798 = local write "SO2 Zero CAL Flush\nTime Remain (sec)"(w1933) -> ()
              n799 = case shown="False" w1934 {
                selector: w1934 -> [w1942 _]
                frame False {
                  n800 = local write "SO2 Calibration Abort"(w1942) -> ()
                }
                frame True {
                }
              }
            }
            n801 = case shown="False" w1891 {
              tunnel: w1896 -> [w1904 w1928]
              tunnel: w1894 -> [w1903 w1927]
              tunnel: [w1901 w1928] -> w1893
              tunnel: [w1899 w1927] -> w1892
              frame False {
                w1905 = TRUE ("SO2 Flush")
                # "carry on cal when no connection problem or abort not confirmed"
                n802 = Bundle(cluster=T4 {"Message"="", "Message Data"=variant} ("Message Cluster"), "Message"="V8", "Message Data"=w1905) -> (w1906:T4)
                n803 = local write "eV8"(w1905) -> ()
                n804 = Enqueue Element(queue=w1904, element=w1906, error in (no error)=w1903) -> (queue out=w1902:refnum<queue>, error out=w1900:errorcluster)  [unwired: 1 in, 1 out]
                n805 = for {
                  N: "eV8 User\nset time (sec)" -> [w1921]
                  tunnel: [w1911] -> w1901
                  tunnel: w1902 -> [w1911]
                  tunnel: [w1910] -> w1899
                  tunnel: w1900 -> [w1910]
                  i -> [w1920]
                  stop <- w1912 stop-if-true
                  n806 = local read "SO2 Calibration Abort"() -> (w1918:bool)
                  n807 = case shown="True" w1918 {
                    selector: w1918 -> [w1924 _]
                    tunnel: [w1924 w1925] -> w1915
                    frame False {
                    }
                    frame True {
                      n808 = Two Button Dialog(message="Are you sure to abort SO2 Cal?") -> (T button?=w1925:bool)  [unwired: 2 in]
                    }
                  }
                  n809 = Subtract(x=w1921, y=w1920) -> (x-y=w1919:i32)
                  n810 = local read "Network disconnected"() -> (w1916:bool)
                  n811 = Decrement(x=w1919) -> (x-1=w1914:i32)
                  n812 = Or(x=w1916, y=w1915) -> (x .or. y?=w1912:bool)
                  n813 = Select(t=0, s=w1912, f=w1914) -> (s? t:f=w1913:i32)
                  n814 = case shown="False" w1915 {
                    selector: w1915 -> [w1923 _]
                    frame False {
                      n815 = local write "SO2 Calibration Abort"(w1923) -> ()
                    }
                    frame True {
                    }
                  }
                  n816 = local write "SO2 Zero CAL\nTime Remain (sec)"(w1913) -> ()
                  n817 = Wait (ms)(milliseconds to wait=u32 1000) -> ()  [unwired: 1 out]
                }
              }
              frame True {
                # "Ignore the rest of the cal when there is connection problem or abort confirmed"
              }
            }
          }
          frame #3 {
            n818 = Cluster To Array(cluster=cluster{"Message":string, "Message 2":string} {"Message"="V8", "Message 2"="V9"}) -> (array=w1951:string[])
            n819 = for {
              tunnel: w1951 -> [w1958] mode=indexing
              tunnel: FALSE ("SO2 Flush") -> [w1957]
              tunnel: w1949 -> [w1956]
              tunnel: w1948 -> [w1955]
              tunnel: [w1954] -> w1947
              tunnel: [w1953] -> w1946
              n820 = Bundle(cluster=T4 {"Message"="", "Message Data"=variant} ("Message Cluster"), "Message"=w1958, "Message Data"=w1957) -> (w1959:T4)
              n821 = Enqueue Element(queue=w1956, element=w1959, error in (no error)=w1955) -> (queue out=w1954:refnum<queue>, error out=w1953:errorcluster)  [unwired: 1 in, 1 out]
            }
          }
          frame #4 {
            w1961 = 0.0 ("MFC_2\nSLPM Value")
            n822 = local write "MFC_2\nSLPM Value"(w1961) -> ()
            n823 = Bundle(cluster=T4 {"Message"="", "Message Data"=variant} ("Message Cluster"), "Message"="MFC_2", "Message Data"=w1961) -> (w1964:T4)
            n824 = Enqueue Element(queue=w1963, element=w1964, error in (no error)=w1962) -> ()  [unwired: 1 in, 3 out]
          }
          frame #5 {
            w1967 = FALSE ("SO2 Flush")
            n825 = local write "eV9"(w1967) -> ()
            n826 = local write "eV8"(w1967) -> ()
            n827 = local write "SO2 Zero CAL"(w1967) -> ()
            n828 = local write "SO2 Calibration Abort"(w1967) -> ()
          }
        }
      }
      event "SO2 Span Calibration": Value Change {
        n829 = event-data() -> ()  [unwired: 1 in, 1 out]
        n830 = flat-sequence {
          tunnel: w1984 -> [w1989]
          tunnel: w1985 -> [w1990]
          tunnel: [w1987] -> w1973
          tunnel: [w1988] -> w1972
          tunnel: [w1997] -> w1971
          tunnel: [w1995] -> w1969
          tunnel: w1973 -> [w1998]
          tunnel: w1972 -> [w1999]
          tunnel: w1971 -> [w2006]
          tunnel: [w2005] -> w1970
          tunnel: w1969 -> [w2004]
          tunnel: [w2003] -> w1968
          tunnel: [w2020] -> w1983
          tunnel: [w2019] -> w1981
          tunnel: w1970 -> [w2024]
          tunnel: w1968 -> [w2017]
          tunnel: w1983 -> [w2028]
          tunnel: [w2027] -> w1982
          tunnel: w1981 -> [w2029]
          tunnel: [w2025] -> w1980
          tunnel: [w2036] -> w1979
          tunnel: [w2035] -> w1978
          tunnel: w1980 -> [w2040]
          tunnel: w1982 -> [w2038]
          tunnel: w1979 -> [w2091]
          tunnel: w1978 -> [w2090]
          tunnel: [w2089] -> w1977
          tunnel: [w2088] -> w1976
          tunnel: w1977 -> [w2107]
          tunnel: w1976 -> [w2106]
          tunnel: [w2104] -> w1975
          tunnel: [w2103] -> w1974
          tunnel: w1975 -> [w2112]
          tunnel: w1974 -> [w2111]
          frame #0 {
            n831 = local write "SO2 Auto Zeroing"(FALSE ("SO2 Auto Zeroing")) -> ()
            n832 = Bundle(cluster=T4 {"Message"="", "Message Data"=variant} ("Message Cluster"), "Message"="Auto_zero", "Message Data"=FALSE) -> (w1992:T4)
            n833 = Enqueue Element(queue=w1990, element=w1992, error in (no error)=w1989) -> (queue out=w1987:refnum<queue>, error out=w1988:errorcluster)  [unwired: 1 in, 1 out]
          }
          frame #1 {
            n834 = Bundle(cluster=T4 {"Message"="", "Message Data"=variant} ("Message Cluster"), "Message"="mean_cal_status", "Message Data"=FALSE) -> (w2000:T4)
            n835 = Enqueue Element(queue=w1998, element=w2000, error in (no error)=w1999) -> (queue out=w1995:refnum<queue>, error out=w1997:errorcluster)  [unwired: 1 in, 1 out]
          }
          frame #2 {
            n836 = node-c288() -> (w2008:T6)  [unwired: 4 in]
            n837 = timed-loop {
              timing: w2008 -> [_]
              timing-out: [_] -> w2007
              tunnel: [w2010] -> w2005
              tunnel: w2006 -> [w2010]
              tunnel: w2004 -> [w2009]
              tunnel: [w2009] -> w2003
              stop <- w2011 stop-if-true
              n838 = node-c288() -> ()  [unwired: 1 in, 1 out]
              n839 = node-c288() -> ()  [unwired: 1 in, 1 out]
              n840 = One Button Dialog(message="Is Span Gas connected to CALDECK?") -> (true=w2011:bool)  [unwired: 1 in]
            }
            n841 = node-c288(w2007) -> ()  [unwired: 1 out]
          }
          frame #3 {
            w2018 = TRUE ("SO2 Flush")
            n842 = Bundle(cluster=T4 {"Message"="", "Message Data"=variant} ("Message Cluster"), "Message"="V9", "Message Data"=w2018) -> (w2021:T4)
            n843 = local write "eV9"(w2018) -> ()
            n844 = Enqueue Element(queue=w2017, element=w2021, error in (no error)=w2024) -> (queue out=w2019:refnum<queue>, error out=w2020:errorcluster)  [unwired: 1 in, 1 out]
          }
          frame #4 {
            n845 = local read "MFC_2 User Set Value"() -> (w2026:dbl)
            n846 = local write "MFC_2\nSLPM Value"(w2026) -> ()
            n847 = Bundle(cluster=T4 {"Message"="", "Message Data"=variant} ("Message Cluster"), "Message"="MFC_2", "Message Data"=w2026) -> (w2030:T4)
            n848 = Enqueue Element(queue=w2029, element=w2030, error in (no error)=w2028) -> (queue out=w2025:refnum<queue>, error out=w2027:errorcluster)  [unwired: 1 in, 1 out]
          }
          frame #5 {
            n849 = for {
              N: "eV9 span\nflush (sec)" -> [w2082]
              tunnel: [w2073] -> w2039
              tunnel: w2040 -> [w2073]
              tunnel: [w2072] -> w2037
              tunnel: w2038 -> [w2072]
              tunnel: [w2071] -> w2034
              i -> [w2081]
              stop <- w2071 stop-if-true
              n850 = local read "SO2 Calibration Abort"() -> (w2078:bool)
              n851 = case shown="True" w2078 {
                selector: w2078 -> [w2085 _]
                tunnel: [w2085 w2086] -> w2076
                frame False {
                }
                frame True {
                  n852 = Two Button Dialog(message="Are you sure to abort SO2 Cal?") -> (T button?=w2086:bool)  [unwired: 2 in]
                }
              }
              n853 = Subtract(x=w2082, y=w2081) -> (x-y=w2080:i32)
              n854 = Decrement(x=w2080) -> (x-1=w2074:i32)
              n855 = Wait (ms)(milliseconds to wait=u32 1000) -> ()  [unwired: 1 out]
              n856 = local read "Network disconnected"() -> (w2077:bool)
              n857 = Or(x=w2077, y=w2076) -> (x .or. y?=w2071:bool)
              n858 = Select(t=0, s=w2071, f=w2074) -> (s? t:f=w2075:i32)
              n859 = local write "SO2 Zero CAL Flush\nTime Remain (sec)"(w2075) -> ()
              n860 = case shown="False" w2076 {
                selector: w2076 -> [w2084 _]
                frame False {
                  n861 = local write "SO2 Calibration Abort"(w2084) -> ()
                }
                frame True {
                }
              }
            }
            n862 = case shown="False" w2034 {
              tunnel: w2039 -> [w2047 w2070]
              tunnel: w2037 -> [w2046 w2069]
              tunnel: [w2044 w2070] -> w2036
              tunnel: [w2042 w2069] -> w2035
              frame False {
                w2048 = TRUE ("SO2 Flush")
                # "carry on cal when no connection problem or abort not confirmed"
                n863 = Bundle(cluster=T4 {"Message"="", "Message Data"=variant} ("Message Cluster"), "Message"="V8", "Message Data"=w2048) -> (w2049:T4)
                n864 = local write "eV8"(w2048) -> ()
                n865 = Enqueue Element(queue=w2047, element=w2049, error in (no error)=w2046) -> (queue out=w2045:refnum<queue>, error out=w2043:errorcluster)  [unwired: 1 in, 1 out]
                n866 = for {
                  N: "eV8 span\n(sec)" -> [w2063]
                  tunnel: [w2053] -> w2044
                  tunnel: w2045 -> [w2053]
                  tunnel: [w2052] -> w2042
                  tunnel: w2043 -> [w2052]
                  i -> [w2062]
                  stop <- w2054 stop-if-true
                  n867 = local read "SO2 Calibration Abort"() -> (w2060:bool)
                  n868 = case shown="True" w2060 {
                    selector: w2060 -> [w2066 _]
                    tunnel: [w2066 w2067] -> w2057
                    frame False {
                    }
                    frame True {
                      n869 = Two Button Dialog(message="Are you sure to abort SO2 Cal?") -> (T button?=w2067:bool)  [unwired: 2 in]
                    }
                  }
                  n870 = Subtract(x=w2063, y=w2062) -> (x-y=w2061:i32)
                  n871 = local read "Network disconnected"() -> (w2058:bool)
                  n872 = Decrement(x=w2061) -> (x-1=w2056:i32)
                  n873 = Or(x=w2058, y=w2057) -> (x .or. y?=w2054:bool)
                  n874 = Select(t=0, s=w2054, f=w2056) -> (s? t:f=w2055:i32)
                  n875 = case shown="False" w2057 {
                    selector: w2057 -> [w2065 _]
                    frame False {
                      n876 = local write "SO2 Calibration Abort"(w2065) -> ()
                    }
                    frame True {
                    }
                  }
                  n877 = local write "SO2 Zero CAL\nTime Remain (sec)"(w2055) -> ()
                  n878 = Wait (ms)(milliseconds to wait=u32 1000) -> ()  [unwired: 1 out]
                }
              }
              frame True {
                # "Ignore the rest of the cal when there is connection problem or abort confirmed"
              }
            }
          }
          frame #6 {
            n879 = Cluster To Array(cluster=cluster{"Message":string, "Message 2":string} {"Message"="V8", "Message 2"="V9"}) -> (array=w2093:string[])
            n880 = for {
              tunnel: w2093 -> [w2100] mode=indexing
              tunnel: FALSE ("SO2 Flush") -> [w2099]
              tunnel: w2091 -> [w2098]
              tunnel: w2090 -> [w2097]
              tunnel: [w2096] -> w2089
              tunnel: [w2095] -> w2088
              n881 = Bundle(cluster=T4 {"Message"="", "Message Data"=variant} ("Message Cluster"), "Message"=w2100, "Message Data"=w2099) -> (w2101:T4)
              n882 = Enqueue Element(queue=w2098, element=w2101, error in (no error)=w2097) -> (queue out=w2096:refnum<queue>, error out=w2095:errorcluster)  [unwired: 1 in, 1 out]
            }
          }
          frame #7 {
            w2105 = 0.0 ("MFC_2\nSLPM Value")
            n883 = local write "MFC_2\nSLPM Value"(w2105) -> ()
            n884 = Bundle(cluster=T4 {"Message"="", "Message Data"=variant} ("Message Cluster"), "Message"="MFC_2", "Message Data"=w2105) -> (w2108:T4)
            n885 = Enqueue Element(queue=w2107, element=w2108, error in (no error)=w2106) -> (queue out=w2104:refnum<queue>, error out=w2103:errorcluster)  [unwired: 1 in, 1 out]
          }
          frame #8 {
            n886 = Bundle(cluster=T4 {"Message"="", "Message Data"=variant} ("Message Cluster"), "Message"="mean_cal_status", "Message Data"=TRUE) -> (w2114:T4)
            n887 = Enqueue Element(queue=w2112, element=w2114, error in (no error)=w2111) -> ()  [unwired: 1 in, 3 out]
          }
          frame #9 {
            w2117 = FALSE ("SO2 Flush")
            n888 = local write "eV8"(w2117) -> ()
            n889 = local write "eV9"(w2117) -> ()
            n890 = local write "SO2 Span Calibration"(w2117) -> ()
            n891 = local write "SO2 Calibration Abort"(w2117) -> ()
          }
        }
      }
      event "SO2 Zero Calibration": Value Change {
        n892 = event-data() -> ()  [unwired: 1 in, 1 out]
        n893 = flat-sequence {
          tunnel: w2132 -> [w2138]
          tunnel: w2133 -> [w2139]
          tunnel: [w2136] -> w2123
          tunnel: [w2137] -> w2122
          tunnel: [w2145] -> w2121
          tunnel: [w2143] -> w2119
          tunnel: w2123 -> [w2146]
          tunnel: w2122 -> [w2147]
          tunnel: w2121 -> [w2153]
          tunnel: [w2152] -> w2120
          tunnel: w2119 -> [w2154]
          tunnel: [w2151] -> w2118
          tunnel: [w2168] -> w2131
          tunnel: [w2167] -> w2129
          tunnel: w2120 -> [w2172]
          tunnel: w2118 -> [w2165]
          tunnel: w2131 -> [w2176]
          tunnel: [w2175] -> w2130
          tunnel: w2129 -> [w2177]
          tunnel: [w2173] -> w2128
          tunnel: [w2184] -> w2127
          tunnel: [w2183] -> w2126
          tunnel: w2128 -> [w2188]
          tunnel: w2130 -> [w2186]
          tunnel: w2127 -> [w2239]
          tunnel: w2126 -> [w2238]
          tunnel: [w2237] -> w2125
          tunnel: [w2236] -> w2124
          tunnel: w2125 -> [w2253]
          tunnel: w2124 -> [w2252]
          frame #0 {
            n894 = local write "SO2 Auto Zeroing"(FALSE) -> ()
            n895 = Bundle(cluster=T4 {"Message"="", "Message Data"=variant} ("Message Cluster"), "Message"="Auto_zero", "Message Data"=FALSE) -> (w2142:T4)
            n896 = Enqueue Element(queue=w2139, element=w2142, error in (no error)=w2138) -> (queue out=w2136:refnum<queue>, error out=w2137:errorcluster)  [unwired: 1 in, 1 out]
          }
          frame #1 {
            n897 = Bundle(cluster=T4 {"Message"="", "Message Data"=variant} ("Message Cluster"), "Message"="mean_cal_status", "Message Data"=TRUE) -> (w2148:T4)
            n898 = Enqueue Element(queue=w2146, element=w2148, error in (no error)=w2147) -> (queue out=w2143:refnum<queue>, error out=w2145:errorcluster)  [unwired: 1 in, 1 out]
          }
          frame #2 {
            n899 = node-c288() -> (w2156:T6)  [unwired: 4 in]
            n900 = timed-loop {
              timing: w2156 -> [_]
              timing-out: [_] -> w2155
              tunnel: [w2158] -> w2152
              tunnel: w2153 -> [w2158]
              tunnel: w2154 -> [w2157]
              tunnel: [w2157] -> w2151
              stop <- w2159 stop-if-true
              n901 = node-c288() -> ()  [unwired: 1 in, 1 out]
              n902 = node-c288() -> ()  [unwired: 1 in, 1 out]
              n903 = One Button Dialog(message="Is Zero Gas connected to CALDECK?") -> (true=w2159:bool)  [unwired: 1 in]
            }
            n904 = node-c288(w2155) -> ()  [unwired: 1 out]
          }
          frame #3 {
            w2166 = TRUE ("SO2 Flush")
            n905 = Bundle(cluster=T4 {"Message"="", "Message Data"=variant} ("Message Cluster"), "Message"="V9", "Message Data"=w2166) -> (w2169:T4)
            n906 = local write "eV9"(w2166) -> ()
            n907 = Enqueue Element(queue=w2165, element=w2169, error in (no error)=w2172) -> (queue out=w2167:refnum<queue>, error out=w2168:errorcluster)  [unwired: 1 in, 1 out]
          }
          frame #4 {
            n908 = local read "MFC_2 User Set Value"() -> (w2174:dbl)
            n909 = local write "MFC_2\nSLPM Value"(w2174) -> ()
            n910 = Bundle(cluster=T4 {"Message"="", "Message Data"=variant} ("Message Cluster"), "Message"="MFC_2", "Message Data"=w2174) -> (w2178:T4)
            n911 = Enqueue Element(queue=w2177, element=w2178, error in (no error)=w2176) -> (queue out=w2173:refnum<queue>, error out=w2175:errorcluster)  [unwired: 1 in, 1 out]
          }
          frame #5 {
            n912 = for {
              N: "eV9 zero\nflush (sec)" -> [w2230]
              tunnel: [w2221] -> w2187
              tunnel: w2188 -> [w2221]
              tunnel: [w2220] -> w2185
              tunnel: w2186 -> [w2220]
              tunnel: [w2219] -> w2182
              i -> [w2229]
              stop <- w2219 stop-if-true
              n913 = local read "SO2 Calibration Abort"() -> (w2226:bool)
              n914 = case shown="True" w2226 {
                selector: w2226 -> [w2233 _]
                tunnel: [w2233 w2234] -> w2224
                frame False {
                }
                frame True {
                  n915 = Two Button Dialog(message="Are you sure to abort SO2 Cal?") -> (T button?=w2234:bool)  [unwired: 2 in]
                }
              }
              n916 = Subtract(x=w2230, y=w2229) -> (x-y=w2228:i32)
              n917 = Decrement(x=w2228) -> (x-1=w2222:i32)
              n918 = Wait (ms)(milliseconds to wait=u32 1000) -> ()  [unwired: 1 out]
              n919 = local read "Network disconnected"() -> (w2225:bool)
              n920 = Or(x=w2225, y=w2224) -> (x .or. y?=w2219:bool)
              n921 = Select(t=0, s=w2219, f=w2222) -> (s? t:f=w2223:i32)
              n922 = local write "SO2 Zero CAL Flush\nTime Remain (sec)"(w2223) -> ()
              n923 = case shown="False" w2224 {
                selector: w2224 -> [w2232 _]
                frame False {
                  n924 = local write "SO2 Calibration Abort"(w2232) -> ()
                }
                frame True {
                }
              }
            }
            n925 = case shown="False" w2182 {
              tunnel: w2187 -> [w2195 w2218]
              tunnel: w2185 -> [w2194 w2217]
              tunnel: [w2192 w2218] -> w2184
              tunnel: [w2190 w2217] -> w2183
              frame False {
                w2196 = TRUE ("SO2 Flush")
                # "carry on cal when no connection problem or abort not confirmed"
                n926 = Bundle(cluster=T4 {"Message"="", "Message Data"=variant} ("Message Cluster"), "Message"="V8", "Message Data"=w2196) -> (w2197:T4)
                n927 = local write "eV8"(w2196) -> ()
                n928 = Enqueue Element(queue=w2195, element=w2197, error in (no error)=w2194) -> (queue out=w2193:refnum<queue>, error out=w2191:errorcluster)  [unwired: 1 in, 1 out]
                n929 = for {
                  N: "eV8 zero\n(sec)" -> [w2211]
                  tunnel: [w2201] -> w2192
                  tunnel: w2193 -> [w2201]
                  tunnel: [w2200] -> w2190
                  tunnel: w2191 -> [w2200]
                  i -> [w2210]
                  stop <- w2202 stop-if-true
                  n930 = local read "SO2 Calibration Abort"() -> (w2208:bool)
                  n931 = case shown="True" w2208 {
                    selector: w2208 -> [w2214 _]
                    tunnel: [w2214 w2215] -> w2205
                    frame False {
                    }
                    frame True {
                      n932 = Two Button Dialog(message="Are you sure to abort SO2 Cal?") -> (T button?=w2215:bool)  [unwired: 2 in]
                    }
                  }
                  n933 = Subtract(x=w2211, y=w2210) -> (x-y=w2209:i32)
                  n934 = local read "Network disconnected"() -> (w2206:bool)
                  n935 = Decrement(x=w2209) -> (x-1=w2204:i32)
                  n936 = Or(x=w2206, y=w2205) -> (x .or. y?=w2202:bool)
                  n937 = Select(t=0, s=w2202, f=w2204) -> (s? t:f=w2203:i32)
                  n938 = case shown="False" w2205 {
                    selector: w2205 -> [w2213 _]
                    frame False {
                      n939 = local write "SO2 Calibration Abort"(w2213) -> ()
                    }
                    frame True {
                    }
                  }
                  n940 = local write "SO2 Zero CAL\nTime Remain (sec)"(w2203) -> ()
                  n941 = Wait (ms)(milliseconds to wait=u32 1000) -> ()  [unwired: 1 out]
                }
              }
              frame True {
                # "Ignore the rest of the cal when there is connection problem or abort confirmed"
              }
            }
          }
          frame #6 {
            n942 = Cluster To Array(cluster=cluster{"Message":string, "Message 2":string} {"Message"="V8", "Message 2"="V9"}) -> (array=w2241:string[])
            n943 = for {
              tunnel: w2241 -> [w2248] mode=indexing
              tunnel: FALSE ("SO2 Flush") -> [w2247]
              tunnel: w2239 -> [w2246]
              tunnel: w2238 -> [w2245]
              tunnel: [w2244] -> w2237
              tunnel: [w2243] -> w2236
              n944 = Bundle(cluster=T4 {"Message"="", "Message Data"=variant} ("Message Cluster"), "Message"=w2248, "Message Data"=w2247) -> (w2249:T4)
              n945 = Enqueue Element(queue=w2246, element=w2249, error in (no error)=w2245) -> (queue out=w2244:refnum<queue>, error out=w2243:errorcluster)  [unwired: 1 in, 1 out]
            }
          }
          frame #7 {
            w2251 = 0.0 ("MFC_2\nSLPM Value")
            n946 = local write "MFC_2\nSLPM Value"(w2251) -> ()
            n947 = Bundle(cluster=T4 {"Message"="", "Message Data"=variant} ("Message Cluster"), "Message"="MFC_2", "Message Data"=w2251) -> (w2254:T4)
            n948 = Enqueue Element(queue=w2253, element=w2254, error in (no error)=w2252) -> ()  [unwired: 1 in, 3 out]
          }
          frame #8 {
            w2257 = FALSE ("SO2 Flush")
            n949 = local write "eV8"(w2257) -> ()
            n950 = local write "eV9"(w2257) -> ()
            n951 = local write "SO2 Zero Calibration"(w2257) -> ()
            n952 = local write "SO2 Calibration Abort"(w2257) -> ()
          }
        }
      }
      event "eV8 User\nset time (sec)": Value Change {
        n953 = event-data() -> ("NewVal"=w2260:i32)  [unwired: 1 in]
        n954 = Bundle(cluster=T4 {"Message"="", "Message Data"=variant} ("Message Cluster"), "Message"="eV8_user_set_time", "Message Data"=w2260) -> (w2261:T4)
        n955 = Enqueue Element(queue=w2259, element=w2261, error in (no error)=w2258) -> ()  [unwired: 1 in, 3 out]
      }
      event "Offset Mean Zero Calculation (default = ON)\nOFF = User input\nOn = Mean zero calculated with ev8": Value Change {
        n956 = event-data() -> ("NewVal"=w2266:bool)  [unwired: 1 in]
        n957 = Bundle(cluster=T4 {"Message"="", "Message Data"=variant} ("Message Cluster"), "Message"="mean_cal_status", "Message Data"=w2266) -> (w2267:T4)
        n958 = Enqueue Element(queue=w2265, element=w2267, error in (no error)=w2264) -> ()  [unwired: 1 in, 3 out]
      }
      event "MFC_2\nSLPM Value": Value Change {
        n959 = event-data() -> ("NewVal"=w2273:dbl)  [unwired: 1 in]
        n960 = Bundle(cluster=T4 {"Message"="", "Message Data"=variant} ("Message Cluster"), "Message"="MFC_2", "Message Data"=w2273) -> (w2271:T4)
        n961 = Enqueue Element(queue=w2276, element=w2271, error in (no error)=w2275) -> (error out=w2270:errorcluster)  [unwired: 1 in, 2 out]
      }
      event "SO2 Inflight MOCCA Alarm\n(default = OFF)": Value Change {
        n962 = event-data() -> ("NewVal"=w2280:bool)  [unwired: 1 in]
        n963 = Bundle(cluster=T4 {"Message"="", "Message Data"=variant} ("Message Cluster"), "Message"="SO2_MOCCA_Alarm", "Message Data"=w2280) -> (w2281:T4)
        n964 = Enqueue Element(queue=w2279, element=w2281, error in (no error)=w2278) -> (error out=w2277:errorcluster)  [unwired: 1 in, 2 out]
      }
      event "MOCCA window \ndelay time (sec)": Value Change {
        n965 = event-data() -> ("NewVal"=w2286:i32)  [unwired: 1 in]
        n966 = Bundle(cluster=T4 {"Message"="", "Message Data"=variant} ("Message Cluster"), "Message"="MOCCA_window_delay_time", "Message Data"=w2286) -> (w2288:T4)
        n967 = Enqueue Element(queue=w2287, element=w2288, error in (no error)=w2285) -> (error out=w2284:errorcluster)  [unwired: 1 in, 2 out]
      }
      event "MOCCA Limit": Value Change {
        n968 = event-data() -> ("NewVal"=w2291:i32)  [unwired: 1 in]
        n969 = Bundle(cluster=T4 {"Message"="", "Message Data"=variant} ("Message Cluster"), "Message"="MOCCA_limit", "Message Data"=w2291) -> (w2294:T4)
        n970 = Enqueue Element(queue=w2293, element=w2294, error in (no error)=w2292) -> ()  [unwired: 1 in, 3 out]
      }
      event "Save Calibration gas\ncylinder concentration to file": Value Change {
        n971 = event-data() -> ("NewVal"=w2297:bool)  [unwired: 1 in]
        n972 = Bundle(cluster=T4 {"Message"="", "Message Data"=variant} ("Message Cluster"), "Message"="calcon_save", "Message Data"=w2297) -> (w2301:T4)
        n973 = Enqueue Element(queue=w2300, element=w2301, error in (no error)=w2299) -> (error out=w2298:errorcluster)  [unwired: 1 in, 2 out]
      }
      event "Calibration gas cylinder \nconcentration (ppb)": Value Change {
        n974 = event-data() -> ("NewVal"=w2304:dbl)  [unwired: 1 in]
        n975 = Bundle(cluster=T4 {"Message"="", "Message Data"=variant} ("Message Cluster"), "Message"="cal_gas_cylin_conc", "Message Data"=w2304) -> (w2307:T4)
        n976 = Enqueue Element(queue=w2306, element=w2307, error in (no error)=w2305) -> ()  [unwired: 1 in, 3 out]
      }
      event "Simulate MOCCA Conc": Value Change {
        n977 = event-data() -> ("NewVal"=w2310:dbl)  [unwired: 1 in]
        n978 = Bundle(cluster=T4 {"Message"="", "Message Data"=variant} ("Message Cluster"), "Message"="sim_MOCCA_conc", "Message Data"=w2310) -> (w2313:T4)
        n979 = Enqueue Element(queue=w2312, element=w2313, error in (no error)=w2311) -> ()  [unwired: 1 in, 3 out]
      }
      event "MFC_3\nSLPM Value": Value Change {
        n980 = event-data() -> ("NewVal"=w2319:dbl)  [unwired: 1 in]
        n981 = Bundle(cluster=T4 {"Message"="", "Message Data"=variant} ("Message Cluster"), "Message"="MFC_3", "Message Data"=w2319) -> (w2317:T4)
        n982 = Enqueue Element(queue=w2322, element=w2317, error in (no error)=w2321) -> (error out=w2316:errorcluster)  [unwired: 1 in, 2 out]
      }
      event "eV8": Value Change {
        n983 = event-data() -> ("NewVal"=w2323:bool)  [unwired: 1 in]
        n984 = Bundle(cluster=T4 {"Message"="", "Message Data"=variant} ("Message Cluster"), "Message"="V8", "Message Data"=w2323) -> (w2327:T4)
        n985 = Enqueue Element(queue=w2326, element=w2327, error in (no error)=w2325) -> (error out=w2324:errorcluster)  [unwired: 1 in, 2 out]
      }
      event "SO2 eV6": Value Change {
        n986 = event-data() -> ("NewVal"=w2330:bool)  [unwired: 1 in]
        n987 = Bundle(cluster=T4 {"Message"="", "Message Data"=variant} ("Message Cluster"), "Message"="V6", "Message Data"=w2330) -> (w2334:T4)
        n988 = Enqueue Element(queue=w2333, element=w2334, error in (no error)=w2332) -> (error out=w2331:errorcluster)  [unwired: 1 in, 2 out]
      }
      event "Simulate Conc": Value Change {
        n989 = event-data() -> ("NewVal"=w2337:bool)  [unwired: 1 in]
        n990 = Bundle(cluster=T4 {"Message"="", "Message Data"=variant} ("Message Cluster"), "Message"="Simulate Conc", "Message Data"=w2337) -> (w2341:T4)
        n991 = Enqueue Element(queue=w2340, element=w2341, error in (no error)=w2339) -> (error out=w2338:errorcluster)  [unwired: 1 in, 2 out]
      }
      event "SO2 UDP Time Offset": Value Change {
        n992 = event-data() -> ("NewVal"=w2344:i32)  [unwired: 1 in]
        n993 = Bundle(cluster=T4 {"Message"="", "Message Data"=variant} ("Message Cluster"), "Message"="UDP Time Offset", "Message Data"=w2344) -> (w2348:T4)
        n994 = Enqueue Element(queue=w2347, element=w2348, error in (no error)=w2346) -> (error out=w2345:errorcluster)  [unwired: 1 in, 2 out]
      }
      event "Simulate STEL Conc": Value Change {
        n995 = event-data() -> ("NewVal"=w2351:dbl)  [unwired: 1 in]
        n996 = Bundle(cluster=T4 {"Message"="", "Message Data"=variant} ("Message Cluster"), "Message"="Simulate STEL Conc", "Message Data"=w2351) -> (w2355:T4)
        n997 = Enqueue Element(queue=w2354, element=w2355, error in (no error)=w2353) -> (error out=w2352:errorcluster)  [unwired: 1 in, 2 out]
      }
      event "Simulate TWA Conc": Value Change {
        n998 = event-data() -> ("NewVal"=w2358:dbl)  [unwired: 1 in]
        n999 = Bundle(cluster=T4 {"Message"="", "Message Data"=variant} ("Message Cluster"), "Message"="Simulate TWA Conc", "Message Data"=w2358) -> (w2362:T4)
        n1000 = Enqueue Element(queue=w2361, element=w2362, error in (no error)=w2360) -> (error out=w2359:errorcluster)  [unwired: 1 in, 2 out]
      }
      event "10mins STEL Limit": Value Change {
        n1001 = event-data() -> ("NewVal"=w2365:i32)  [unwired: 1 in]
        n1002 = Bundle(cluster=T4 {"Message"="", "Message Data"=variant} ("Message Cluster"), "Message"="10mins STEL Limit", "Message Data"=w2365) -> (w2369:T4)
        n1003 = Enqueue Element(queue=w2368, element=w2369, error in (no error)=w2367) -> (error out=w2366:errorcluster)  [unwired: 1 in, 2 out]
      }
      event "8hr TWA Limit": Value Change {
        n1004 = event-data() -> ("NewVal"=w2372:i32)  [unwired: 1 in]
        n1005 = Bundle(cluster=T4 {"Message"="", "Message Data"=variant} ("Message Cluster"), "Message"="8hr TWA Limit", "Message Data"=w2372) -> (w2376:T4)
        n1006 = Enqueue Element(queue=w2375, element=w2376, error in (no error)=w2374) -> (error out=w2373:errorcluster)  [unwired: 1 in, 2 out]
      }
      event "SO2 Zero": Value Change {
        n1007 = event-data() -> ("NewVal"=w2379:dbl)  [unwired: 1 in]
        n1008 = Bundle(cluster=T4 {"Message"="", "Message Data"=variant} ("Message Cluster"), "Message"="Offset", "Message Data"=w2379) -> (w2383:T4)
        n1009 = Enqueue Element(queue=w2382, element=w2383, error in (no error)=w2381) -> (error out=w2380:errorcluster)  [unwired: 1 in, 2 out]
      }
      event "SO2 Sensitivity": Value Change {
        n1010 = event-data() -> ("NewVal"=w2386:dbl)  [unwired: 1 in]
        n1011 = Bundle(cluster=T4 {"Message"="", "Message Data"=variant} ("Message Cluster"), "Message"="Slope", "Message Data"=w2386) -> (w2390:T4)
        n1012 = Enqueue Element(queue=w2389, element=w2390, error in (no error)=w2388) -> (error out=w2387:errorcluster)  [unwired: 1 in, 2 out]
      }
      event "Confirm Flight Number": Value Change {
        n1013 = event-data() -> ()  [unwired: 1 in, 6 out]
        n1014 = flat-sequence {
          tunnel: w2396 -> [w2399]
          tunnel: w2397 -> [w2400]
          tunnel: [w2400] -> w2394
          tunnel: [w2399] -> w2393
          tunnel: [w2402] -> w2395
          tunnel: w2394 -> [w2404]
          tunnel: w2393 -> [w2403]
          frame #0 {
            n1015 = local write "cRIO File IO Stop\n(USB Flash Drive Unmount)"(FALSE ("cRIO File IO Stop\n(USB Flash Drive Unmount)")) -> ()
          }
          frame #1 {
            n1016 = local read "Flight Number"() -> (w2401:string)
            n1017 = Bundle(cluster=T4 {"Message"="", "Message Data"=variant} ("Message Cluster"), "Message"="Flight Number", "Message Data"=w2401) -> (w2405:T4)
            n1018 = Enqueue Element(queue=w2404, element=w2405, error in (no error)=w2403) -> (error out=w2402:errorcluster)  [unwired: 1 in, 2 out]
          }
        }
      }
      event "cRIO File IO Stop\n(USB Flash Drive Unmount)": Value Change {
        n1019 = event-data() -> ("NewVal"=w2408:bool)  [unwired: 1 in]
        n1020 = Bundle(cluster=T4 {"Message"="", "Message Data"=variant} ("Message Cluster"), "Message"="Stop File Write", "Message Data"=w2408) -> (w2412:T4)
        n1021 = Enqueue Element(queue=w2411, element=w2412, error in (no error)=w2410) -> (error out=w2409:errorcluster)  [unwired: 1 in, 2 out]
      }
    }
    "SO2 Event error out" <- w1716
  }
  n1022 = Create Network Stream Writer Endpoint(6:w45, 7:10 ("writer buffer size"), 9:w40, 10:"//192.168.101.17/command/reader/SO2" ("reader url"), 11:"/command/writer/SO2" ("writer name")) -> (0:w44:errorcluster, 3:w43:refnum<k21>)  [unwired: 2 in]
  n1023 = while {
    tunnel: w4 -> [w2419]
    tunnel: w3 -> [w2418]
    stop <- FALSE stop-if-true
    # "SO2 Auto Zero Handler Loop"
    n1024 = local read "Network disconnected"() -> (w2416:bool)
    n1025 = local read "SO2 Zero CAL"() -> (w2423:bool)
    n1026 = Equal?(x=w2423, y=FALSE) -> (x = y?=w2421:bool)
    n1027 = Equal?(x=w2416, y=FALSE) -> (x = y?=w2415:bool)
    n1028 = Compound Arithmetic op=AND("SO2 Auto Zeroing", w2421, w2415) -> (w2424:bool)
    n1029 = case shown="False" w2424 {
      tunnel: w2419 -> [_ w2443]
      tunnel: w2418 -> [_ w2442]
      frame False {
        n1030 = local write "Auto Zero\nIndicator"("Auto Zero Inactive; Manual Zero Allow" ("Auto Zero Indicator")) -> ()
        n1031 = local write "SO2 Pause\nAuto Zeroing"(FALSE ("SO2 Pause\nAuto Zeroing")) -> ()
        n1032 = property on="SO2 Zero CAL" class="Bool (strict)"("Visible"=TRUE) -> ()  [unwired: 2 in, 2 out]
      }
      frame True {
        n1033 = flat-sequence {
          tunnel: w2442 -> [w2452]
          tunnel: w2443 -> [w2453]
          tunnel: [w2453] -> w2441
          tunnel: [w2452] -> w2440
          tunnel: w2441 -> [w2462]
          tunnel: w2440 -> [w2461]
          tunnel: [w2460] -> w2439
          tunnel: [w2459] -> w2438
          tunnel: [w2468] -> w2449
          tunnel: [w2467] -> w2448
          tunnel: w2439 -> [w2472]
          tunnel: w2438 -> [w2473]
          tunnel: w2449 -> [w2477]
          tunnel: [w2476] -> w2447
          tunnel: w2448 -> [w2478]
          tunnel: [w2475] -> w2446
          tunnel: w2447 -> [w2486]
          tunnel: w2446 -> [w2488]
          tunnel: [w2484] -> w2431
          tunnel: [w2483] -> w2430
          tunnel: [w2538] -> w2445
          tunnel: [w2537] -> w2444
          tunnel: w2431 -> [w2540]
          tunnel: w2430 -> [w2539]
          tunnel: w2445 -> [w2556]
          tunnel: w2444 -> [w2555]
          tunnel: [w2553] -> w2436
          tunnel: [w2552] -> w2435
          tunnel: [w2561] -> w2437
          tunnel: w2436 -> [w2561]
          tunnel: w2435 -> [w2560]
          tunnel: [w2560] -> w2434
          tunnel: [w2566] -> w2433
          tunnel: w2434 -> [w2565]
          tunnel: w2437 -> [w2566]
          tunnel: [w2565] -> w2432
          tunnel: w2433 -> [w2600]
          tunnel: w2432 -> [w2599]
          frame #0 {
            n1034 = local write "Auto Zero\nIndicator"("Auto Zero In Progress" ("Auto Zero\nIndicator")) -> ()
            n1035 = while {
              stop <- w2454 stop-if-true
              n1036 = local read "eV9"() -> (w2456:bool)
              n1037 = Equal?(x=w2456, y=FALSE) -> (x = y?=w2454:bool)
              n1038 = Wait (ms)(milliseconds to wait=u32 1000) -> ()  [unwired: 1 out]
            }
            n1039 = property on="SO2 Zero CAL" class="Bool (strict)"("Visible"=FALSE) -> ()  [unwired: 2 in, 2 out]
          }
          frame #1 {
            n1040 = Bundle(cluster=T4 {"Message"="", "Message Data"=variant} ("Message Cluster"), "Message"="Auto_zero", "Message Data"=TRUE) -> (w2463:T4)
            n1041 = Enqueue Element(queue=w2462, element=w2463, error in (no error)=w2461) -> (queue out=w2459:refnum<queue>, error out=w2460:errorcluster)  [unwired: 1 in, 1 out]
          }
          frame #2 {
            w2466 = TRUE ("SO2 Flush")
            n1042 = Bundle(cluster=T4 {"Message"="", "Message Data"=variant} ("Message Cluster"), "Message"="V9", "Message Data"=w2466) -> (w2469:T4)
            n1043 = local write "eV9"(w2466) -> ()
            n1044 = Enqueue Element(queue=w2473, element=w2469, error in (no error)=w2472) -> (queue out=w2467:refnum<queue>, error out=w2468:errorcluster)  [unwired: 1 in, 1 out]
          }
          frame #3 {
            n1045 = local read "MFC_2 User Set Value"() -> (w2474:dbl)
            n1046 = local write "MFC_2 User Set Value"(w2474) -> ()
            n1047 = Bundle(cluster=T4 {"Message"="", "Message Data"=variant} ("Message Cluster"), "Message"="MFC_2", "Message Data"=w2474) -> (w2479:T4)
            n1048 = Enqueue Element(queue=w2478, element=w2479, error in (no error)=w2477) -> (queue out=w2475:refnum<queue>, error out=w2476:errorcluster)  [unwired: 1 in, 1 out]
          }
          frame #4 {
            n1049 = local read "eV9 flush User\nset time (sec)"() -> (w2489:i32)
            n1050 = for {
              N: w2489 -> [w2531]
              tunnel: [w2522] -> w2487
              tunnel: w2488 -> [w2522]
              tunnel: [w2521] -> w2485
              tunnel: w2486 -> [w2521]
              tunnel: [w2520] -> w2482
              i -> [w2530]
              stop <- w2520 stop-if-true
              n1051 = local read "Network disconnected"() -> (w2524:bool)
              n1052 = local read "SO2 Calibration Abort"() -> (w2525:bool)
              n1053 = case shown="True" w2525 {
                selector: w2525 -> [w2534 _]
                tunnel: [w2534 w2535] -> w2523
                frame False {
                }
                frame True {
                  n1054 = Two Button Dialog(message="Are you sure to abort SO2 Cal?") -> (T button?=w2535:bool)  [unwired: 2 in]
                }
              }
              n1055 = Subtract(x=w2531, y=w2530) -> (x-y=w2529:i32)
              n1056 = Decrement(x=w2529) -> (x-1=w2527:i32)
              n1057 = Or(x=w2523, y=w2524) -> (x .or. y?=w2520:bool)
              n1058 = Wait (ms)(milliseconds to wait=u32 1000) -> ()  [unwired: 1 out]
              n1059 = Select(t=0, s=w2520, f=w2527) -> (s? t:f=w2526:i32)
              n1060 = local write "SO2 Zero CAL Flush\nTime Remain (sec)"(w2526) -> ()
              n1061 = case shown="False" w2523 {
                selector: w2523 -> [w2533 _]
                frame False {
                  n1062 = local write "SO2 Calibration Abort"(w2533) -> ()
                }
                frame True {
                }
              }
            }
            n1063 = case shown="False" w2482 {
              tunnel: w2487 -> [w2495 w2519]
              tunnel: w2485 -> [w2494 w2518]
              tunnel: [w2493 w2519] -> w2484
              tunnel: [w2491 w2518] -> w2483
              frame False {
                w2496 = TRUE ("SO2 Flush")
                # "carry on cal when no connection problem or abort not confirmed"
                n1064 = Bundle(cluster=T4 {"Message"="", "Message Data"=variant} ("Message Cluster"), "Message"="V8", "Message Data"=w2496) -> (w2497:T4)
                n1065 = local write "eV8"(w2496) -> ()
                n1066 = Enqueue Element(queue=w2495, element=w2497, error in (no error)=w2494) -> (queue out=w2492:refnum<queue>, error out=w2490:errorcluster)  [unwired: 1 in, 1 out]
                n1067 = local read "eV8 User\nset time (sec)"() -> (w2500:i32)
                n1068 = for {
                  N: w2500 -> [w2512]
                  tunnel: w2492 -> [w2502]
                  tunnel: [w2502] -> w2493
                  tunnel: w2490 -> [w2501]
                  tunnel: [w2501] -> w2491
                  i -> [w2511]
                  stop <- w2503 stop-if-true
                  n1069 = local read "Network disconnected"() -> (w2507:bool)
                  n1070 = local read "SO2 Calibration Abort"() -> (w2509:bool)
                  n1071 = case shown="True" w2509 {
                    selector: w2509 -> [w2515 _]
                    tunnel: [w2515 w2516] -> w2504
                    frame False {
                    }
                    frame True {
                      n1072 = Two Button Dialog(message="Are you sure to abort SO2 Cal?") -> (T button?=w2516:bool)  [unwired: 2 in]
                    }
                  }
                  n1073 = Subtract(x=w2512, y=w2511) -> (x-y=w2510:i32)
                  n1074 = Decrement(x=w2510) -> (x-1=w2505:i32)
                  n1075 = Or(x=w2504, y=w2507) -> (x .or. y?=w2503:bool)
                  n1076 = Wait (ms)(milliseconds to wait=u32 1000) -> ()  [unwired: 1 out]
                  n1077 = Select(t=0, s=w2503, f=w2505) -> (s? t:f=w2506:i32)
                  n1078 = case shown="False" w2504 {
                    selector: w2504 -> [w2514 _]
                    frame False {
                      n1079 = local write "SO2 Calibration Abort"(w2514) -> ()
                    }
                    frame True {
                    }
                  }
                  n1080 = local write "SO2 Zero CAL\nTime Remain (sec)"(w2506) -> ()
                }
              }
              frame True {
                # "Ignore cal when connection problem or abort confirmed"
              }
            }
          }
          frame #5 {
            n1081 = Cluster To Array(cluster=cluster{"Message":string, "Message 2":string} {"Message"="V8", "Message 2"="V9"}) -> (array=w2542:string[])
            n1082 = for {
              tunnel: w2542 -> [w2549] mode=indexing
              tunnel: FALSE ("SO2 Flush") -> [w2548]
              tunnel: w2540 -> [w2547]
              tunnel: w2539 -> [w2546]
              tunnel: [w2545] -> w2538
              tunnel: [w2544] -> w2537
              n1083 = Bundle(cluster=T4 {"Message"="", "Message Data"=variant} ("Message Cluster"), "Message"=w2549, "Message Data"=w2548) -> (w2550:T4)
              n1084 = Enqueue Element(queue=w2547, element=w2550, error in (no error)=w2546) -> (queue out=w2545:refnum<queue>, error out=w2544:errorcluster)  [unwired: 1 in, 1 out]
            }
          }
          frame #6 {
            w2554 = 0.0 ("MFC_2\nSLPM Value")
            n1085 = local write "MFC_2\nSLPM Value"(w2554) -> ()
            n1086 = Bundle(cluster=T4 {"Message"="", "Message Data"=variant} ("Message Cluster"), "Message"="MFC_2", "Message Data"=w2554) -> (w2557:T4)
            n1087 = Enqueue Element(queue=w2556, element=w2557, error in (no error)=w2555) -> (queue out=w2553:refnum<queue>, error out=w2552:errorcluster)  [unwired: 1 in, 1 out]
          }
          frame #7 {
            w2562 = FALSE ("SO2 Flush")
            n1088 = local write "eV8"(w2562) -> ()
            n1089 = local write "eV9"(w2562) -> ()
          }
          frame #8 {
            n1090 = for {
              N: "Auto Zeroing \ninterval (sec)" -> [w2578]
              tunnel: [w2573] -> w2563
              i -> [w2577]
              stop <- w2573 stop-if-true
              n1091 = local read "SO2 Pause\nAuto Zeroing"() -> (w2571:bool)
              n1092 = Subtract(x=w2578, y=w2577) -> (x-y=w2579:i32)
              n1093 = Equal?(x=w2571, y=TRUE) -> (x = y?=w2569:bool)
              n1094 = Decrement(x=w2579) -> (x-1=→"Next Auto Zero\nStarts in (sec)":i32)
              n1095 = Wait (ms)(milliseconds to wait=u32 1000) -> ()  [unwired: 1 out]
              n1096 = case shown="True" w2569 {
                selector: w2569 -> [w2581 _]
                tunnel: [w2581 FALSE] -> w2568
                frame False {
                }
                frame True {
                  n1097 = for {
                    N: "Pause Auto Zero Count \nDown set time (sec)" -> [w2595]
                    tunnel: [w2587] -> w2583
                    i -> [w2594]
                    stop <- w2587 stop-if-true
                    w2588 = FALSE
                    n1098 = local read "SO2 Pause\nAuto Zeroing"() -> (w2590:bool)
                    n1099 = local read "SO2 Auto Zeroing"() -> (w2591:bool)
                    n1100 = Subtract(x=w2595, y=w2594) -> (x-y=w2596:i32)
                    n1101 = Decrement(x=w2596) -> (x-1=→"SO2 Resume Zeroing\nCount down timer (sec)":i32)
                    n1102 = Wait (ms)(milliseconds to wait=u32 1000) -> ()  [unwired: 1 out]
                    n1103 = Equal?(x=w2591, y=w2588) -> (x = y?=w2592:bool)
                    n1104 = Equal?(x=w2590, y=w2588) -> (x = y?=w2589:bool)
                    n1105 = Or(x=w2592, y=w2589) -> (x .or. y?=w2587:bool)
                  }
                  n1106 = case shown="True" w2583 {
                    frame False {
                    }
                    frame True {
                      n1107 = local write "SO2 Resume Zeroing\nCount down timer (sec)"(u32 0 ("SO2 Resume Zeroing\nCount down timer (sec)")) -> ()
                    }
                  }
                  n1108 = local write "Auto Zero\nIndicator"("Auto Zero Paused" ("Auto Zero\nIndicator")) -> ()
                }
              }
              n1109 = local write "Auto Zero\nIndicator"("Waiting For The Next Zeroing\nInterrupt Waiting by Pressing Pause Auto Zeroing button " ("Auto Zero\nIndicator")) -> ()
              n1110 = local read "SO2 Auto Zeroing"() -> (w2574:bool)
              n1111 = local write "SO2 Pause\nAuto Zeroing"(w2568) -> ()
              n1112 = Equal?(x=w2574, y=FALSE) -> (x = y?=w2573:bool)
            }
            n1113 = case shown="True" w2563 {
              frame False {
              }
              frame True {
                n1114 = local write "Next Auto Zero\nStarts in (sec)"(u32 0 ("Next Auto Zero\nStarts in (sec)")) -> ()
              }
            }
          }
          frame #9 {
            n1115 = local write "SO2 Calibration Abort"(FALSE) -> ()
            n1116 = Bundle(cluster=T4 {"Message"="", "Message Data"=variant} ("Message Cluster"), "Message"="Auto_zero", "Message Data"=FALSE) -> (w2603:T4)
            n1117 = Enqueue Element(queue=w2600, element=w2603, error in (no error)=w2599) -> ()  [unwired: 1 in, 3 out]
          }
        }
      }
    }
    n1118 = Wait (ms)(milliseconds to wait=u32 100) -> ()  [unwired: 1 out]
  }
  n1119 = while {
    tunnel: w4 -> [w2612]
    shift-right: [w2607] -> _
    shift-left: w43 -> [w2609]
    shift-right: [w2605] -> w41
    shift-left: w44 -> [w2611]
    tunnel: w3 -> [w2606]
    stop <- w2605 stop-if-true
    # "SO2 UI Command Sender"
    n1120 = Dequeue Element(queue=w2612, error in (no error)=w2606) -> (element=w2608:T4)  [unwired: 1 in, 3 out]
    n1121 = Unbundle By Name(w2608) -> ("Message"=w2610:string)
    n1122 = case shown="\"zeroing_interval\"" w2610 {
      tunnel: w2611 -> [w2613 w2617 w2624 w2631 w2638 w2645 w2652 w2659 w2666 w2673 w2680 w2687 w2694 w2701 w2708 w2715 w2722 w2729 w2736 w2743 w2750 w2757 w2764 w2771 w2778 w2785]
      tunnel: w2609 -> [w2614 w2620 w2627 w2634 w2641 w2648 w2655 w2662 w2669 w2676 w2683 w2690 w2697 w2704 w2711 w2718 w2725 w2732 w2739 w2746 w2753 w2760 w2767 w2774 w2781 w2788]
      tunnel: w2608 -> [_ w2619 w2626 w2633 w2640 w2647 w2654 w2661 w2668 w2675 w2682 w2689 w2696 w2703 w2710 w2717 w2724 w2731 w2738 w2745 w2752 w2759 w2766 w2773 w2780 w2787]
      tunnel: [w2613 w2616 w2623 w2630 w2637 w2644 w2651 w2658 w2665 w2672 w2679 w2686 w2693 w2700 w2707 w2714 w2721 w2728 w2735 w2742 w2749 w2756 w2763 w2770 w2777 w2784] -> w2605
      tunnel: [w2614 w2615 w2622 w2629 w2636 w2643 w2650 w2657 w2664 w2671 w2678 w2685 w2692 w2699 w2706 w2713 w2720 w2727 w2734 w2741 w2748 w2755 w2762 w2769 w2776 w2783] -> w2607
      frame "False", Default {
      }
      frame "V9" {
        n1123 = shared-variable-write(w2620, w2617, w2619) -> (w2618:refnum<k21>, w2621:errorcluster)  [unwired: 1 in, 1 out]
        n1124 = Flush Stream(8:w2621, 11:w2618) -> (0:w2616:errorcluster, 3:w2615:refnum<k21>)  [unwired: 2 in, 1 out]
      }
      frame "MFC_2" {
        n1125 = shared-variable-write(w2627, w2624, w2626) -> (w2625:refnum<k21>, w2628:errorcluster)  [unwired: 1 in, 1 out]
        n1126 = Flush Stream(8:w2628, 11:w2625) -> (0:w2623:errorcluster, 3:w2622:refnum<k21>)  [unwired: 2 in, 1 out]
      }
      frame "MFC_3" {
        n1127 = shared-variable-write(w2634, w2631, w2633) -> (w2632:refnum<k21>, w2635:errorcluster)  [unwired: 1 in, 1 out]
        n1128 = Flush Stream(8:w2635, 11:w2632) -> (0:w2630:errorcluster, 3:w2629:refnum<k21>)  [unwired: 2 in, 1 out]
      }
      frame "V6" {
        n1129 = shared-variable-write(w2641, w2638, w2640) -> (w2639:refnum<k21>, w2642:errorcluster)  [unwired: 1 in, 1 out]
        n1130 = Flush Stream(8:w2642, 11:w2639) -> (0:w2637:errorcluster, 3:w2636:refnum<k21>)  [unwired: 2 in, 1 out]
      }
      frame "Simulate Conc" {
        n1131 = shared-variable-write(w2648, w2645, w2647) -> (w2646:refnum<k21>, w2649:errorcluster)  [unwired: 1 in, 1 out]
        n1132 = Flush Stream(8:w2649, 11:w2646) -> (0:w2644:errorcluster, 3:w2643:refnum<k21>)  [unwired: 2 in, 1 out]
      }
      frame "Simulate STEL Conc" {
        n1133 = shared-variable-write(w2655, w2652, w2654) -> (w2653:refnum<k21>, w2656:errorcluster)  [unwired: 1 in, 1 out]
        n1134 = Flush Stream(8:w2656, 11:w2653) -> (0:w2651:errorcluster, 3:w2650:refnum<k21>)  [unwired: 2 in, 1 out]
      }
      frame "Simulate TWA Conc" {
        n1135 = shared-variable-write(w2662, w2659, w2661) -> (w2660:refnum<k21>, w2663:errorcluster)  [unwired: 1 in, 1 out]
        n1136 = Flush Stream(8:w2663, 11:w2660) -> (0:w2658:errorcluster, 3:w2657:refnum<k21>)  [unwired: 2 in, 1 out]
      }
      frame "10mins STEL Limit" {
        n1137 = shared-variable-write(w2669, w2666, w2668) -> (w2667:refnum<k21>, w2670:errorcluster)  [unwired: 1 in, 1 out]
        n1138 = Flush Stream(8:w2670, 11:w2667) -> (0:w2665:errorcluster, 3:w2664:refnum<k21>)  [unwired: 2 in, 1 out]
      }
      frame "8hr TWA Limit" {
        n1139 = shared-variable-write(w2676, w2673, w2675) -> (w2674:refnum<k21>, w2677:errorcluster)  [unwired: 1 in, 1 out]
        n1140 = Flush Stream(8:w2677, 11:w2674) -> (0:w2672:errorcluster, 3:w2671:refnum<k21>)  [unwired: 2 in, 1 out]
      }
      frame "Offset" {
        n1141 = shared-variable-write(w2683, w2680, w2682) -> (w2681:refnum<k21>, w2684:errorcluster)  [unwired: 1 in, 1 out]
        n1142 = Flush Stream(8:w2684, 11:w2681) -> (0:w2679:errorcluster, 3:w2678:refnum<k21>)  [unwired: 2 in, 1 out]
      }
      frame "eV8_user_set_time" {
        n1143 = shared-variable-write(w2690, w2687, w2689) -> (w2688:refnum<k21>, w2691:errorcluster)  [unwired: 1 in, 1 out]
        n1144 = Flush Stream(8:w2691, 11:w2688) -> (0:w2686:errorcluster, 3:w2685:refnum<k21>)  [unwired: 2 in, 1 out]
      }
      frame "mean_cal_status" {
        n1145 = shared-variable-write(w2697, w2694, w2696) -> (w2695:refnum<k21>, w2698:errorcluster)  [unwired: 1 in, 1 out]
        n1146 = Flush Stream(8:w2698, 11:w2695) -> (0:w2693:errorcluster, 3:w2692:refnum<k21>)  [unwired: 2 in, 1 out]
      }
      frame "SO2_MOCCA_Alarm" {
        n1147 = shared-variable-write(w2704, w2701, w2703) -> (w2702:refnum<k21>, w2705:errorcluster)  [unwired: 1 in, 1 out]
        n1148 = Flush Stream(8:w2705, 11:w2702) -> (0:w2700:errorcluster, 3:w2699:refnum<k21>)  [unwired: 2 in, 1 out]
      }
      frame "MOCCA_window_delay_time" {
        n1149 = shared-variable-write(w2711, w2708, w2710) -> (w2709:refnum<k21>, w2712:errorcluster)  [unwired: 1 in, 1 out]
        n1150 = Flush Stream(8:w2712, 11:w2709) -> (0:w2707:errorcluster, 3:w2706:refnum<k21>)  [unwired: 2 in, 1 out]
      }
      frame "MOCCA_limit" {
        n1151 = shared-variable-write(w2718, w2715, w2717) -> (w2716:refnum<k21>, w2719:errorcluster)  [unwired: 1 in, 1 out]
        n1152 = Flush Stream(8:w2719, 11:w2716) -> (0:w2714:errorcluster, 3:w2713:refnum<k21>)  [unwired: 2 in, 1 out]
      }
      frame "calcon_save" {
        n1153 = shared-variable-write(w2725, w2722, w2724) -> (w2723:refnum<k21>, w2726:errorcluster)  [unwired: 1 in, 1 out]
        n1154 = Flush Stream(8:w2726, 11:w2723) -> (0:w2721:errorcluster, 3:w2720:refnum<k21>)  [unwired: 2 in, 1 out]
      }
      frame "Auto_zero" {
        n1155 = shared-variable-write(w2732, w2729, w2731) -> (w2730:refnum<k21>, w2733:errorcluster)  [unwired: 1 in, 1 out]
        n1156 = Flush Stream(8:w2733, 11:w2730) -> (0:w2728:errorcluster, 3:w2727:refnum<k21>)  [unwired: 2 in, 1 out]
      }
      frame "zeroing_interval" {
        n1157 = shared-variable-write(w2739, w2736, w2738) -> (w2737:refnum<k21>, w2740:errorcluster)  [unwired: 1 in, 1 out]
        n1158 = Flush Stream(8:w2740, 11:w2737) -> (0:w2735:errorcluster, 3:w2734:refnum<k21>)  [unwired: 2 in, 1 out]
      }
      frame "cal_gas_cylin_conc" {
        n1159 = shared-variable-write(w2746, w2743, w2745) -> (w2744:refnum<k21>, w2747:errorcluster)  [unwired: 1 in, 1 out]
        n1160 = Flush Stream(8:w2747, 11:w2744) -> (0:w2742:errorcluster, 3:w2741:refnum<k21>)  [unwired: 2 in, 1 out]
      }
      frame "sim_MOCCA_conc" {
        n1161 = shared-variable-write(w2753, w2750, w2752) -> (w2751:refnum<k21>, w2754:errorcluster)  [unwired: 1 in, 1 out]
        n1162 = Flush Stream(8:w2754, 11:w2751) -> (0:w2749:errorcluster, 3:w2748:refnum<k21>)  [unwired: 2 in, 1 out]
      }
      frame "Slope" {
        n1163 = shared-variable-write(w2760, w2757, w2759) -> (w2758:refnum<k21>, w2761:errorcluster)  [unwired: 1 in, 1 out]
        n1164 = Flush Stream(8:w2761, 11:w2758) -> (0:w2756:errorcluster, 3:w2755:refnum<k21>)  [unwired: 2 in, 1 out]
      }
      frame "Flight Number" {
        n1165 = shared-variable-write(w2767, w2764, w2766) -> (w2765:refnum<k21>, w2768:errorcluster)  [unwired: 1 in, 1 out]
        n1166 = Flush Stream(8:w2768, 11:w2765) -> (0:w2763:errorcluster, 3:w2762:refnum<k21>)  [unwired: 2 in, 1 out]
      }
      frame "Stop File Write" {
        n1167 = shared-variable-write(w2774, w2771, w2773) -> (w2772:refnum<k21>, w2775:errorcluster)  [unwired: 1 in, 1 out]
        n1168 = Flush Stream(8:w2775, 11:w2772) -> (0:w2770:errorcluster, 3:w2769:refnum<k21>)  [unwired: 2 in, 1 out]
      }
      frame "UDP Time Offset" {
        n1169 = shared-variable-write(w2781, w2778, w2780) -> (w2779:refnum<k21>, w2782:errorcluster)  [unwired: 1 in, 1 out]
        n1170 = Flush Stream(8:w2782, 11:w2779) -> (0:w2777:errorcluster, 3:w2776:refnum<k21>)  [unwired: 2 in, 1 out]
      }
      frame "V8" {
        n1171 = shared-variable-write(w2788, w2785, w2787) -> (w2786:refnum<k21>, w2789:errorcluster)  [unwired: 1 in, 1 out]
        n1172 = Flush Stream(8:w2789, 11:w2786) -> (0:w2784:errorcluster, 3:w2783:refnum<k21>)  [unwired: 2 in, 1 out]
      }
    }
  }
  "SO2 command sender \nerror out" <- w41
  n1173 = Obtain Queue(name (unnamed)="TEi43c_Command", element data type=w29) -> (queue out=w38:refnum<queue>, error out=w31:errorcluster)  [unwired: 3 in, 1 out]
  n1174 = Create Network Stream Writer Endpoint(6:w35, 7:10 ("writer buffer size"), 9:w29, 10:"//192.168.101.17/command/reader/TEi43c" ("reader url"), 11:"/command/writer/TEi43c" ("writer name")) -> (0:w34:errorcluster, 3:w33:refnum<k21>)  [unwired: 2 in]
  n1175 = while {
    tunnel: w38 -> [w2793]
    tunnel: w31 -> [w2792]
    tunnel: [w2790] -> _
    stop <- FALSE stop-if-true
    # "TEi43c Ozone UI Event Handler Loop"
    n1176 = event shown="[0] \"Ozone Zeroing\": Value Change" {
      selector: _ -> [_ _ _ _ _]
      dyn-events: _ -> [_ _ _ _ _]
      timeout: _ -> [_ _ _ _ _]
      tunnel: w2793 -> [w2801 w2839 w2847 w2854 w2862]
      tunnel: w2792 -> [w2800 w2838 w2846 w2853 w2861]
      tunnel: [w2799 w2837 w2845 w2852 w2860] -> w2790
      event "Ozone Zeroing": Value Change {
        n1177 = event-data() -> ()  [unwired: 1 in, 6 out]
        n1178 = flat-sequence {
          tunnel: w2801 -> [w2806]
          tunnel: w2800 -> [w2805]
          tunnel: [w2804] -> w2798
          tunnel: [w2802] -> w2794
          tunnel: w2798 -> [w2812]
          tunnel: [w2812] -> w2797
          tunnel: [w2810] -> w2795
          tunnel: w2794 -> [w2810]
          tunnel: w2797 -> [w2830]
          tunnel: [w2829] -> w2796
          tunnel: w2795 -> [w2831]
          tunnel: [w2836] -> w2799
          tunnel: w2796 -> [w2836]
          frame #0 {
            w2803 = TRUE
            n1179 = local write "Ozone eV6"(w2803) -> ()
            n1180 = Bundle(cluster=T4 {"Message"="", "Message Data"=variant} ("Message Cluster"), "Message"="V6", "Message Data"=w2803) -> (w2807:T4)
            n1181 = Enqueue Element(queue=w2806, element=w2807, error in (no error)=w2805) -> (queue out=w2802:refnum<queue>, error out=w2804:errorcluster)  [unwired: 1 in, 1 out]
          }
          frame #1 {
            # "10 Mins Count down"
            n1182 = for {
              N: 600 -> [w2822]
              i -> [w2821]
              stop <- w2814 stop-if-true
              n1183 = local read "Ozone Zeroing Abort"() -> (w2816:bool)
              n1184 = Subtract(x=w2822, y=w2821) -> (x-y=w2820:i32)
              n1185 = Decrement(x=w2820) -> (x-1=w2818:i32)
              n1186 = Wait (ms)(milliseconds to wait=u32 1000) -> ()  [unwired: 1 out]
              n1187 = case shown="True" w2816 {
                selector: w2816 -> [w2825 _]
                tunnel: [w2825 w2826] -> w2813
                frame False {
                }
                frame True {
                  n1188 = Two Button Dialog(message="Are you sure to abort Ozone Zeroing?") -> (T button?=w2826:bool)  [unwired: 2 in]
                }
              }
              n1189 = local read "Network disconnected"() -> (w2815:bool)
              n1190 = Or(x=w2815, y=w2813) -> (x .or. y?=w2814:bool)
              n1191 = Select(t=0, s=w2814, f=w2818) -> (s? t:f=→"Ozone Zeroing\nTime Remain (sec)":i32)
              n1192 = case shown="False" w2813 {
                selector: w2813 -> [w2824 _]
                frame False {
                  n1193 = local write "Ozone Zeroing Abort"(w2824) -> ()
                }
                frame True {
                }
              }
            }
          }
          frame #2 {
            w2828 = FALSE
            n1194 = local write "Ozone eV6"(w2828) -> ()
            n1195 = Bundle(cluster=T4 {"Message"="", "Message Data"=variant} ("Message Cluster"), "Message"="V6", "Message Data"=w2828) -> (w2832:T4)
            n1196 = Enqueue Element(queue=w2831, element=w2832, error in (no error)=w2830) -> (error out=w2829:errorcluster)  [unwired: 1 in, 2 out]
          }
          frame #3 {
            w2835 = FALSE ("Ozone Zeroing")
            n1197 = local write "Ozone Zeroing Abort"(w2835) -> ()
            n1198 = local write "Ozone Zeroing"(w2835) -> ()
          }
        }
      }
      event "Ozone eV6": Value Change {
        n1199 = event-data() -> ("NewVal"=w2840:bool)  [unwired: 1 in]
        n1200 = Bundle(cluster=T4 {"Message"="", "Message Data"=variant} ("Message Cluster"), "Message"="V6", "Message Data"=w2840) -> (w2841:T4)
        n1201 = Enqueue Element(queue=w2839, element=w2841, error in (no error)=w2838) -> (error out=w2837:errorcluster)  [unwired: 1 in, 2 out]
      }
      event "cRIO File IO Stop\n(USB Flash Drive Unmount)": Value Change {
        n1202 = event-data() -> ("NewVal"=w2844:bool)  [unwired: 1 in]
        n1203 = Bundle(cluster=T4 {"Message"="", "Message Data"=variant} ("Message Cluster"), "Message"="Stop File Write", "Message Data"=w2844) -> (w2848:T4)
        n1204 = Enqueue Element(queue=w2847, element=w2848, error in (no error)=w2846) -> (error out=w2845:errorcluster)  [unwired: 1 in, 2 out]
      }
      event "Ozone UDP Time Offset": Value Change {
        n1205 = event-data() -> ("NewVal"=w2851:i32)  [unwired: 1 in]
        n1206 = Bundle(cluster=T4 {"Message"="", "Message Data"=variant} ("Message Cluster"), "Message"="UDP Time Offset", "Message Data"=w2851) -> (w2855:T4)
        n1207 = Enqueue Element(queue=w2854, element=w2855, error in (no error)=w2853) -> (error out=w2852:errorcluster)  [unwired: 1 in, 2 out]
      }
      event "Confirm Flight Number": Value Change {
        n1208 = event-data() -> ()  [unwired: 1 in, 5 out]
        n1209 = flat-sequence {
          tunnel: w2861 -> [w2864]
          tunnel: w2862 -> [w2865]
          tunnel: [w2865] -> w2859
          tunnel: [w2864] -> w2858
          tunnel: [w2867] -> w2860
          tunnel: w2859 -> [w2869]
          tunnel: w2858 -> [w2868]
          frame #0 {
            n1210 = local write "cRIO File IO Stop\n(USB Flash Drive Unmount)"(FALSE ("cRIO File IO Stop\n(USB Flash Drive Unmount)")) -> ()
          }
          frame #1 {
            n1211 = local read "Flight Number"() -> (w2866:string)
            n1212 = Bundle(cluster=T4 {"Message"="", "Message Data"=variant} ("Message Cluster"), "Message"="Flight Number", "Message Data"=w2866) -> (w2870:T4)
            n1213 = Enqueue Element(queue=w2869, element=w2870, error in (no error)=w2868) -> (error out=w2867:errorcluster)  [unwired: 1 in, 2 out]
          }
        }
      }
    }
    "Ozone Event error out" <- w2790
  }
  n1214 = while {
    tunnel: w38 -> [w2880]
    shift-right: [w2875] -> _
    shift-left: w33 -> [w2877]
    shift-right: [w2873] -> w30
    shift-left: w34 -> [w2879]
    tunnel: w31 -> [w2874]
    stop <- w2873 stop-if-true
    # "TEi43c Ozone UI Command Sender"
    n1215 = Dequeue Element(queue=w2880, error in (no error)=w2874) -> (element=w2876:T4)  [unwired: 1 in, 3 out]
    n1216 = Unbundle By Name(w2876) -> ("Message"=w2878:string)
    n1217 = case shown="\"UDP Time Offset\"" w2878 {
      tunnel: w2879 -> [w2881 w2885 w2892 w2899 w2906]
      tunnel: w2877 -> [w2882 w2888 w2895 w2902 w2909]
      tunnel: w2876 -> [_ w2887 w2894 w2901 w2908]
      tunnel: [w2881 w2884 w2891 w2898 w2905] -> w2873
      tunnel: [w2882 w2883 w2890 w2897 w2904] -> w2875
      frame "False", Default {
      }
      frame "V6" {
        n1218 = shared-variable-write(w2888, w2885, w2887) -> (w2886:refnum<k21>, w2889:errorcluster)  [unwired: 1 in, 1 out]
        n1219 = Flush Stream(8:w2889, 11:w2886) -> (0:w2884:errorcluster, 3:w2883:refnum<k21>)  [unwired: 2 in, 1 out]
      }
      frame "Stop File Write" {
        n1220 = shared-variable-write(w2895, w2892, w2894) -> (w2893:refnum<k21>, w2896:errorcluster)  [unwired: 1 in, 1 out]
        n1221 = Flush Stream(8:w2896, 11:w2893) -> (0:w2891:errorcluster, 3:w2890:refnum<k21>)  [unwired: 2 in, 1 out]
      }
      frame "Flight Number" {
        n1222 = shared-variable-write(w2902, w2899, w2901) -> (w2900:refnum<k21>, w2903:errorcluster)  [unwired: 1 in, 1 out]
        n1223 = Flush Stream(8:w2903, 11:w2900) -> (0:w2898:errorcluster, 3:w2897:refnum<k21>)  [unwired: 2 in, 1 out]
      }
      frame "UDP Time Offset" {
        n1224 = shared-variable-write(w2909, w2906, w2908) -> (w2907:refnum<k21>, w2910:errorcluster)  [unwired: 1 in, 1 out]
        n1225 = Flush Stream(8:w2910, 11:w2907) -> (0:w2905:errorcluster, 3:w2904:refnum<k21>)  [unwired: 2 in, 1 out]
      }
    }
  }
  "Ozone command sender error out" <- w30
  n1226 = Obtain Queue(name (unnamed)="2BOzone_Command", element data type=w17) -> (queue out=w26:refnum<queue>, error out=w19:errorcluster)  [unwired: 3 in, 1 out]
  n1227 = Create Network Stream Writer Endpoint(6:w23, 7:10 ("writer buffer size"), 9:w17, 10:"//192.168.101.17/command/reader/2BOzone" ("reader url"), 11:"/command/writer/2BOzone" ("writer name")) -> (0:w22:errorcluster, 3:w21:refnum<k21>)  [unwired: 2 in]
  n1228 = while {
    tunnel: w26 -> [w2914]
    tunnel: w19 -> [w2913]
    tunnel: [w2911] -> _
    stop <- FALSE stop-if-true
    # "2BOzone UI Event Handler Loop"
    n1229 = event shown="[2] \"Simulate Inst Conc\": Value Change" {
      selector: _ -> [_ _ _ _ _ _ _ _]
      dyn-events: _ -> [_ _ _ _ _ _ _ _]
      timeout: _ -> [_ _ _ _ _ _ _ _]
      tunnel: w2914 -> [w2918 w2925 w2932 w2939 w2946 w2953 w2960 w2968]
      tunnel: w2913 -> [w2917 w2924 w2931 w2938 w2945 w2952 w2959 w2967]
      tunnel: [w2916 w2923 w2930 w2937 w2944 w2951 w2958 w2966] -> w2911
      event "Ambient = OFF\nCabin = ON": Value Change {
        n1230 = event-data() -> ("NewVal"=w2915:bool)  [unwired: 1 in]
        n1231 = Bundle(cluster=T4 {"Message"="", "Message Data"=variant} ("Message Cluster"), "Message"="Ambient/Cabin", "Message Data"=w2915) -> (w2919:T4)
        n1232 = Enqueue Element(queue=w2918, element=w2919, error in (no error)=w2917) -> (error out=w2916:errorcluster)  [unwired: 1 in, 2 out]
      }
      event "Simulate 2B Conc": Value Change {
        n1233 = event-data() -> ("NewVal"=w2922:bool)  [unwired: 1 in]
        n1234 = Bundle(cluster=T4 {"Message"="", "Message Data"=variant} ("Message Cluster"), "Message"="Simulate_conc", "Message Data"=w2922) -> (w2926:T4)
        n1235 = Enqueue Element(queue=w2925, element=w2926, error in (no error)=w2924) -> (error out=w2923:errorcluster)  [unwired: 1 in, 2 out]
      }
      event "Simulate Inst Conc": Value Change {
        n1236 = event-data() -> ("NewVal"=w2929:i32)  [unwired: 1 in]
        n1237 = Bundle(cluster=T4 {"Message"="", "Message Data"=variant} ("Message Cluster"), "Message"="Simulate_inst_conc", "Message Data"=w2929) -> (w2933:T4)
        n1238 = Enqueue Element(queue=w2932, element=w2933, error in (no error)=w2931) -> (error out=w2930:errorcluster)  [unwired: 1 in, 2 out]
      }
      event "Inst_alm_thresh": Value Change {
        n1239 = event-data() -> ("NewVal"=w2936:i32)  [unwired: 1 in]
        n1240 = Bundle(cluster=T4 {"Message"="", "Message Data"=variant} ("Message Cluster"), "Message"="Inst_alm_thresh", "Message Data"=w2936) -> (w2940:T4)
        n1241 = Enqueue Element(queue=w2939, element=w2940, error in (no error)=w2938) -> (error out=w2937:errorcluster)  [unwired: 1 in, 2 out]
      }
      event "3hr_alm_thresh": Value Change {
        n1242 = event-data() -> ("NewVal"=w2943:i32)  [unwired: 1 in]
        n1243 = Bundle(cluster=T4 {"Message"="", "Message Data"=variant} ("Message Cluster"), "Message"="3hr_alm_thresh", "Message Data"=w2943) -> (w2947:T4)
        n1244 = Enqueue Element(queue=w2946, element=w2947, error in (no error)=w2945) -> (error out=w2944:errorcluster)  [unwired: 1 in, 2 out]
      }
      event "Simulate 3hr Average Conc": Value Change {
        n1245 = event-data() -> ("NewVal"=w2950:dbl)  [unwired: 1 in]
        n1246 = Bundle(cluster=T4 {"Message"="", "Message Data"=variant} ("Message Cluster"), "Message"="Simulate_3hr_av_conc", "Message Data"=w2950) -> (w2954:T4)
        n1247 = Enqueue Element(queue=w2953, element=w2954, error in (no error)=w2952) -> (error out=w2951:errorcluster)  [unwired: 1 in, 2 out]
      }
      event "cRIO File IO Stop\n(USB Flash Drive Unmount)": Value Change {
        n1248 = event-data() -> ("NewVal"=w2957:bool)  [unwired: 1 in]
        n1249 = Bundle(cluster=T4 {"Message"="", "Message Data"=variant} ("Message Cluster"), "Message"="Stop File Write", "Message Data"=w2957) -> (w2961:T4)
        n1250 = Enqueue Element(queue=w2960, element=w2961, error in (no error)=w2959) -> (error out=w2958:errorcluster)  [unwired: 1 in, 2 out]
      }
      event "Confirm Flight Number": Value Change {
        n1251 = event-data() -> ()  [unwired: 1 in, 5 out]
        n1252 = flat-sequence {
          tunnel: w2967 -> [w2970]
          tunnel: w2968 -> [w2971]
          tunnel: [w2971] -> w2965
          tunnel: [w2970] -> w2964
          tunnel: [w2973] -> w2966
          tunnel: w2965 -> [w2975]
          tunnel: w2964 -> [w2974]
          frame #0 {
            n1253 = local write "cRIO File IO Stop\n(USB Flash Drive Unmount)"(FALSE ("cRIO File IO Stop\n(USB Flash Drive Unmount)")) -> ()
          }
          frame #1 {
            n1254 = local read "Flight Number"() -> (w2972:string)
            n1255 = Bundle(cluster=T4 {"Message"="", "Message Data"=variant} ("Message Cluster"), "Message"="Flight Number", "Message Data"=w2972) -> (w2976:T4)
            n1256 = Enqueue Element(queue=w2975, element=w2976, error in (no error)=w2974) -> (error out=w2973:errorcluster)  [unwired: 1 in, 2 out]
          }
        }
      }
    }
    "2BOzone Event error out" <- w2911
  }
  n1257 = while {
    tunnel: w26 -> [w2986]
    shift-right: [w2981] -> _
    shift-left: w21 -> [w2983]
    shift-right: [w2979] -> w18
    shift-left: w22 -> [w2985]
    tunnel: w19 -> [w2980]
    stop <- w2979 stop-if-true
    # "2BOzone UI Command Sender"
    n1258 = Dequeue Element(queue=w2986, error in (no error)=w2980) -> (element=w2982:T4)  [unwired: 1 in, 3 out]
    n1259 = Unbundle By Name(w2982) -> ("Message"=w2984:string)
    n1260 = case shown="\"3hr_alm_thresh\"" w2984 {
      tunnel: w2985 -> [w2987 w2991 w2998 w3005 w3012 w3019 w3026 w3033 w3040]
      tunnel: w2983 -> [w2988 w2994 w3001 w3008 w3015 w3022 w3029 w3036 w3043]
      tunnel: w2982 -> [_ w2993 w3000 w3007 w3014 w3021 w3028 w3035 w3042]
      tunnel: [w2987 w2990 w2997 w3004 w3011 w3018 w3025 w3032 w3039] -> w2979
      tunnel: [w2988 w2989 w2996 w3003 w3010 w3017 w3024 w3031 w3038] -> w2981
      frame "False", Default {
      }
      frame "Ambient/Cabin" {
        n1261 = shared-variable-write(w2994, w2991, w2993) -> (w2992:refnum<k21>, w2995:errorcluster)  [unwired: 1 in, 1 out]
        n1262 = Flush Stream(8:w2995, 11:w2992) -> (0:w2990:errorcluster, 3:w2989:refnum<k21>)  [unwired: 2 in, 1 out]
      }
      frame "Simulate_conc" {
        n1263 = shared-variable-write(w3001, w2998, w3000) -> (w2999:refnum<k21>, w3002:errorcluster)  [unwired: 1 in, 1 out]
        n1264 = Flush Stream(8:w3002, 11:w2999) -> (0:w2997:errorcluster, 3:w2996:refnum<k21>)  [unwired: 2 in, 1 out]
      }
      frame "Simulate_inst_conc" {
        n1265 = shared-variable-write(w3008, w3005, w3007) -> (w3006:refnum<k21>, w3009:errorcluster)  [unwired: 1 in, 1 out]
        n1266 = Flush Stream(8:w3009, 11:w3006) -> (0:w3004:errorcluster, 3:w3003:refnum<k21>)  [unwired: 2 in, 1 out]
      }
      frame "Inst_alm_thresh" {
        n1267 = shared-variable-write(w3015, w3012, w3014) -> (w3013:refnum<k21>, w3016:errorcluster)  [unwired: 1 in, 1 out]
        n1268 = Flush Stream(8:w3016, 11:w3013) -> (0:w3011:errorcluster, 3:w3010:refnum<k21>)  [unwired: 2 in, 1 out]
      }
      frame "3hr_alm_thresh" {
        n1269 = shared-variable-write(w3022, w3019, w3021) -> (w3020:refnum<k21>, w3023:errorcluster)  [unwired: 1 in, 1 out]
        n1270 = Flush Stream(8:w3023, 11:w3020) -> (0:w3018:errorcluster, 3:w3017:refnum<k21>)  [unwired: 2 in, 1 out]
      }
      frame "Simulate_3hr_av_conc" {
        n1271 = shared-variable-write(w3029, w3026, w3028) -> (w3027:refnum<k21>, w3030:errorcluster)  [unwired: 1 in, 1 out]
        n1272 = Flush Stream(8:w3030, 11:w3027) -> (0:w3025:errorcluster, 3:w3024:refnum<k21>)  [unwired: 2 in, 1 out]
      }
      frame "Stop File Write" {
        n1273 = shared-variable-write(w3036, w3033, w3035) -> (w3034:refnum<k21>, w3037:errorcluster)  [unwired: 1 in, 1 out]
        n1274 = Flush Stream(8:w3037, 11:w3034) -> (0:w3032:errorcluster, 3:w3031:refnum<k21>)  [unwired: 2 in, 1 out]
      }
      frame "Flight Number" {
        n1275 = shared-variable-write(w3043, w3040, w3042) -> (w3041:refnum<k21>, w3044:errorcluster)  [unwired: 1 in, 1 out]
        n1276 = Flush Stream(8:w3044, 11:w3041) -> (0:w3039:errorcluster, 3:w3038:refnum<k21>)  [unwired: 2 in, 1 out]
      }
    }
  }
  "2BOzone command sender error out" <- w18
